vi "Main_Marvin Remake.vi"() -> ()   [LabVIEW 2017]
uses:
  PCAN_Driver/ControlCAN.llb/DevType.ctl
  PCAN_Driver/ControlCAN.llb/CAN Channel.ctl
  PCAN_Driver/ControlCAN.llb/VCI_INIT_CONFIG.ctl
  PCAN_Driver/ControlCAN.llb/InitFlag.ctl
  PCAN_Driver/ControlCAN.llb/Fliter.ctl
  PCAN_Driver/ControlCAN.llb/Mode.ctl
  <vilib>/Utility/miscctls.llb/LVRowAndColumnTypeDef.ctl
  <vilib>/Utility/config.llb/Read Key (String).vi
  <vilib>/Utility/config.llb/Write Key (String).vi
  <vilib>/Utility/cursorutil.llb/Set Cursor (Icon Pict).vi
  PCAN_Driver/ControlCAN.lvlib
  <vilib>/Utility/config.llb/NI_LVConfig.lvlib
panel:
  out "UUT from ID":u8
  out "UUT SN Report":string
  out "Automation":bool
  out "Test Failed":bool
  out "AuxiOFFResult":bool
  out "AuxiONResult":bool
  out "SensCalResult":bool
  out "VisualInspectionResult":bool
  out "BurnResult":bool
  out "BurnSpeed":bool
  out "BurnTemp":bool
  out "BurnDC":bool
  out "TempControlResult":bool
  out "MotorTempResult":bool
  out "StopTimeResult":bool
  out "SpeedResult":bool=TRUE
  out "VenableDirectionResult":bool
  out "VenableResult":bool
  out "ComTestResult":bool=TRUE
  out "UUT SoftwareVer":string
  out "Next SN":i32
  in  "SetSN":bool
  out "Current SN":i32
  out "Cal":dbl
  out "AO[1]Meas":dbl
  out "FullSpeed2 Speed":dbl
  out "FullSpeed2 Current":dbl
  out "FullSpeed1 Current":dbl
  out "FullSpeed1 Speed":dbl
  out "MaxBurnInTempVal":dbl
  in  "Stop Burn-in":bool
  out "VISA Tester":refnum<visa-resource-name>
  out "UUT":u8
  out "CAN Status":bool
  in  "Channel 2":T1 caption="Channel" items=["Channel 1", "Channel 2"]
  out "Config_CANAT":T7 {"DevType" items=["USB-CAN"=3, "USB-CAN2"=4]; "CanIndex" items=["通道1", "通道2"]; "VCI_INIT_CONFIG"."Fliter" items=["接收所有类型"=3, "只接收标准帧"=4, "只接收扩展帧"=7]; "VCI_INIT_CONFIG"."Mode" items=["正常工作", "自测模式（环回）", "仅侦听模式"]; "VCI_INIT_CONFIG"."InitFlag" items=["使用Flash参数", "使用界面设置参数"]}
  out "Array":u64[][](array[numeric]) format="%016x"
  out "Motor Phase Current RMS":dbl
  out "Ambient Temperature":dbl
  out "Speed error":bool
  out "Commutation err":bool
  out "Under voltage/Over voltage":bool
  out "Derated drive temp":bool
  out "Motor Over temperature":bool
  out "Motor Sensor temp Fauilre":bool
  out "Drive Over temperature":bool
  out "Drive Sensor temp Failure":bool
  out "Ambient Over temp":bool
  out "Ambient Sensor temp":bool
  out "DC Voltage":dbl
  out "DC Current":dbl
  out "Power transistor Heat sink Temp.":dbl
  out "Motor Stator Temp.":dbl
  out "Motor Speed RPM":dbl
  out "ECS State":u16
  out "UUT":string="EBAY"
  in  "Logger Path":path
  in  "Report":bool
  in  "Start":bool
  in  "ATR":string[][](table)=[["Test Communication", "-", "-", "-", "-", ""], ["Set S/N", "-", "-", "-", "-", ""], ["Set Board Number", "-", "-", "-", "-", ""], [" ", "", "", "", "", ""], ["Test Communication", "-", "-", "-", "-", ""], ["Get S/N", "-", "-", "-", "", ""], ["Get Board Number", "-", "-", "-", "", ""], ["Get FW", "-", "-", "-", "", ""], ["Enable Motor", "", "", "", "", ""], ["Small position command", "", "", "", "", ""], ["Measure delta", "", "", "", "", ""], ["Velocity command", "", "", "", "", ""]]
  in  "Settings":bool
  in  "Refresh Button":bool
  out "Status":bool
  in  "VISA Marvin":refnum<visa-resource-name>="COM6"
  in  "Serial Com":bool
  in  "Help Button":bool
  out "Pannel User Message":string
  in  "Stop Button":bool
  # "Marvin"
  # "REDLER TECHNOLOGIES LTD"
  # "ver 1.2j"
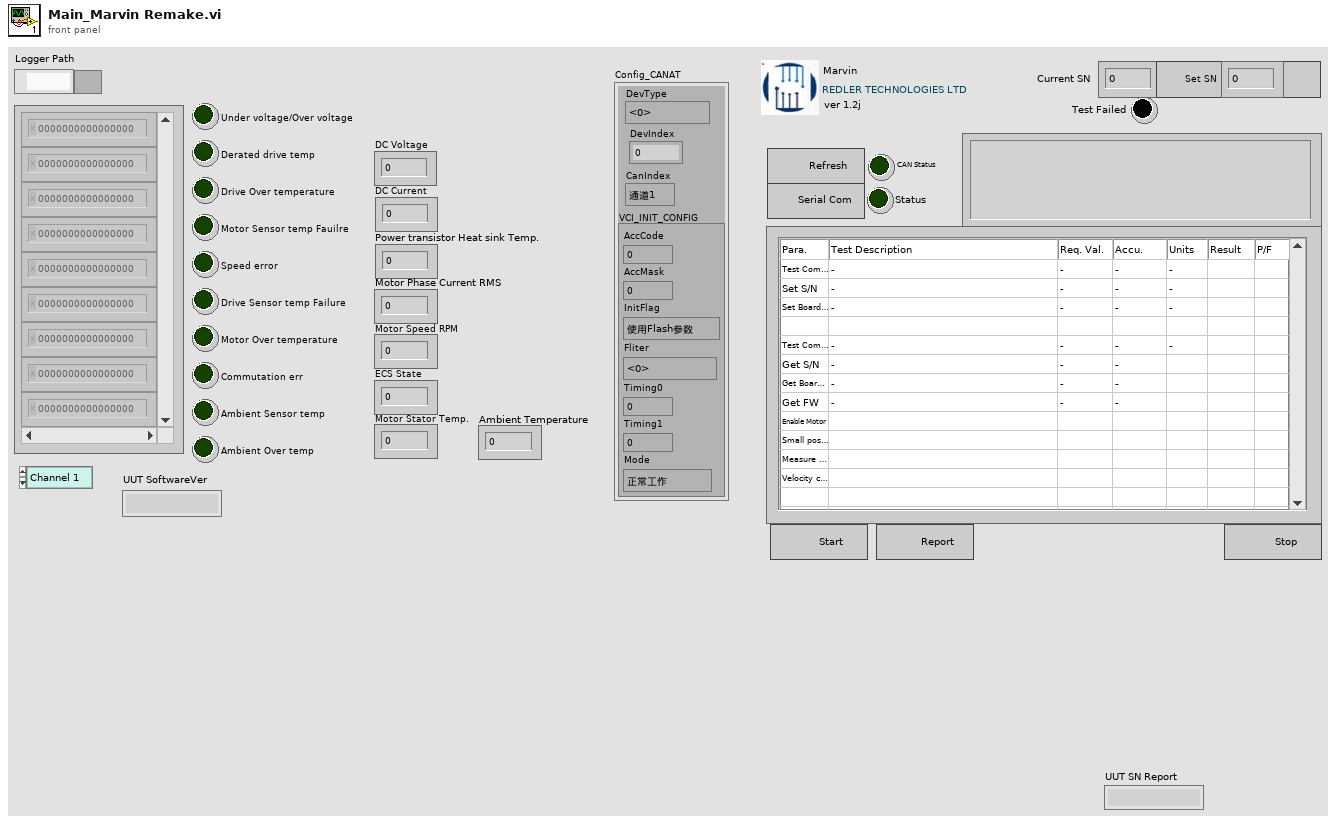
[diagram p1: front panel]
types:
  T1 = typedef "ControlCAN.lvlib/CAN Channel.ctl" = u32
  T2 = typedef "ControlCAN.lvlib/DevType.ctl" = u32
  T3 = typedef "ControlCAN.lvlib/VCI_INIT_CONFIG.ctl" = cluster{"AccCode":u32, "AccMask":u32, "InitFlag":T4, "Fliter":T5, "Timing0":u8, "Timing1":u8, "Mode":T6}
  T4 = typedef "ControlCAN.lvlib/InitFlag.ctl" = u32
  T5 = typedef "ControlCAN.lvlib/Fliter.ctl" = u8
  T6 = typedef "ControlCAN.lvlib/Mode.ctl" = u8
  T7 = cluster{"DevType":T2, "DevIndex":u32, "CanIndex":T1, "VCI_INIT_CONFIG":T3}
  T8 = cluster{"VISA":refnum<visa-resource-name>, "Array Test":enum16{"Auxiliary", "Temp Sens Cal", "Com Test", "Enable Test", "Speed Command", "Stop Time", "Temp Control", "Burn in", "Visual Inspec", "Empty"}[]}
  T9 = cluster{"ID":u32, "MSGTYPE":u8, "LEN":u8, "aDATA":u8[]}[]
  T10 = enum16{"Erase ATR Table", "Stop", "MainProgram", "Initialize"}
  T11 = enum16{"K15", "K16", "K17", "Venable", "Firmeware", "Fan", "Power", "120C", "110C", "100C", "90C", "80C", "70C", "60C", "50C", "40C", "30C", "25C", "20C", "10C", "0C"}
  T12 = enum16{"Stop", "Result", "FullSpeed2", "MD[1]=1", "FullSpeed1", "MD[1]=0"}
  T13 = enum8{"Term1", "Term2", "Current", "Fan", "TempCPU"}
  T14 = enum16{"Stop", "AO[1]=Meas.", "TA[5]", "AO[1]=0", "Start"}
  T15 = enum16{"Stop", "BurnIn", "Ambient Temp", "MotorSpeed", "DC Current Measure", "Start"}
  T16 = enum16{"Auxiliary", "Temp Sens Cal", "Com Test", "Enable Test", "Speed Command", "Stop Time", "Temp Control", "Burn in", "Visual Inspec", "Empty"}[]
  T17 = enum16{"K15", "K16", "K17", "Venable", "Firmeware", "Fan", "Power", "120C", "110C", "100C", "90C", "80C", "70C", "60C", "50C", "40C", "30C", "25C", "20C", "10C", "0C"}[]
  T18 = enum8{"Enabled", "Disabled", "Disabled and Grayed Out"}
  T19 = typedef "LVRowAndColumnTypeDef.ctl" = cluster{"Row":i32, "Column":i32}
  T20 = enum16{"Auxiliary", "Temp Sens Cal", "Com Test", "Enable Test", "Speed Command", "Stop Time", "Temp Control", "Burn in", "Visual Inspec", "Empty"}
  T21 = cluster{"ID":u32, "MSGTYPE":u8, "LEN":u8, "aDATA":u8[]}
  T22 = enum16{"open", "replace", "create", "open or create", "replace or create", "replace or create with confirmation"}
  T23 = enum32{"Invalid", "Standard", "Closed", "Hidden", "Minimized", "Maximized"}
  T24 = typedef "NI_LVConfig.lvlib/Config Data RefNum.ctl" = refnum<k1>
  T25 = typedef "ControlCAN.lvlib/VCI_CAN_OBJ.ctl" = cluster{"ID":u32, "TimeStamp":u32, "TimeFlag":u8, "SendType":u8, "RemoteFlag":u8, "ExternFlag":u8, "DataLen":u8, "Data":u8[], "Reserved":u8[]}
  T26 = cluster{"Type":enum16{"接收", "发送"}, "Channel":T1, "Time":timestamp, "VCI_CAN_OBJ":T25}[]
  T27 = cluster{"Type":enum16{"接收", "发送"}, "Channel":T1, "Time":timestamp, "VCI_CAN_OBJ":T25}
  T28 = typedef "LVPoint32TypeDef.ctl" = cluster{"Horizontal":i32, "Vertical":i32}
  T29 = enum8{"Term1", "Term2", "Current", "Fan", "TempCPU"}[]
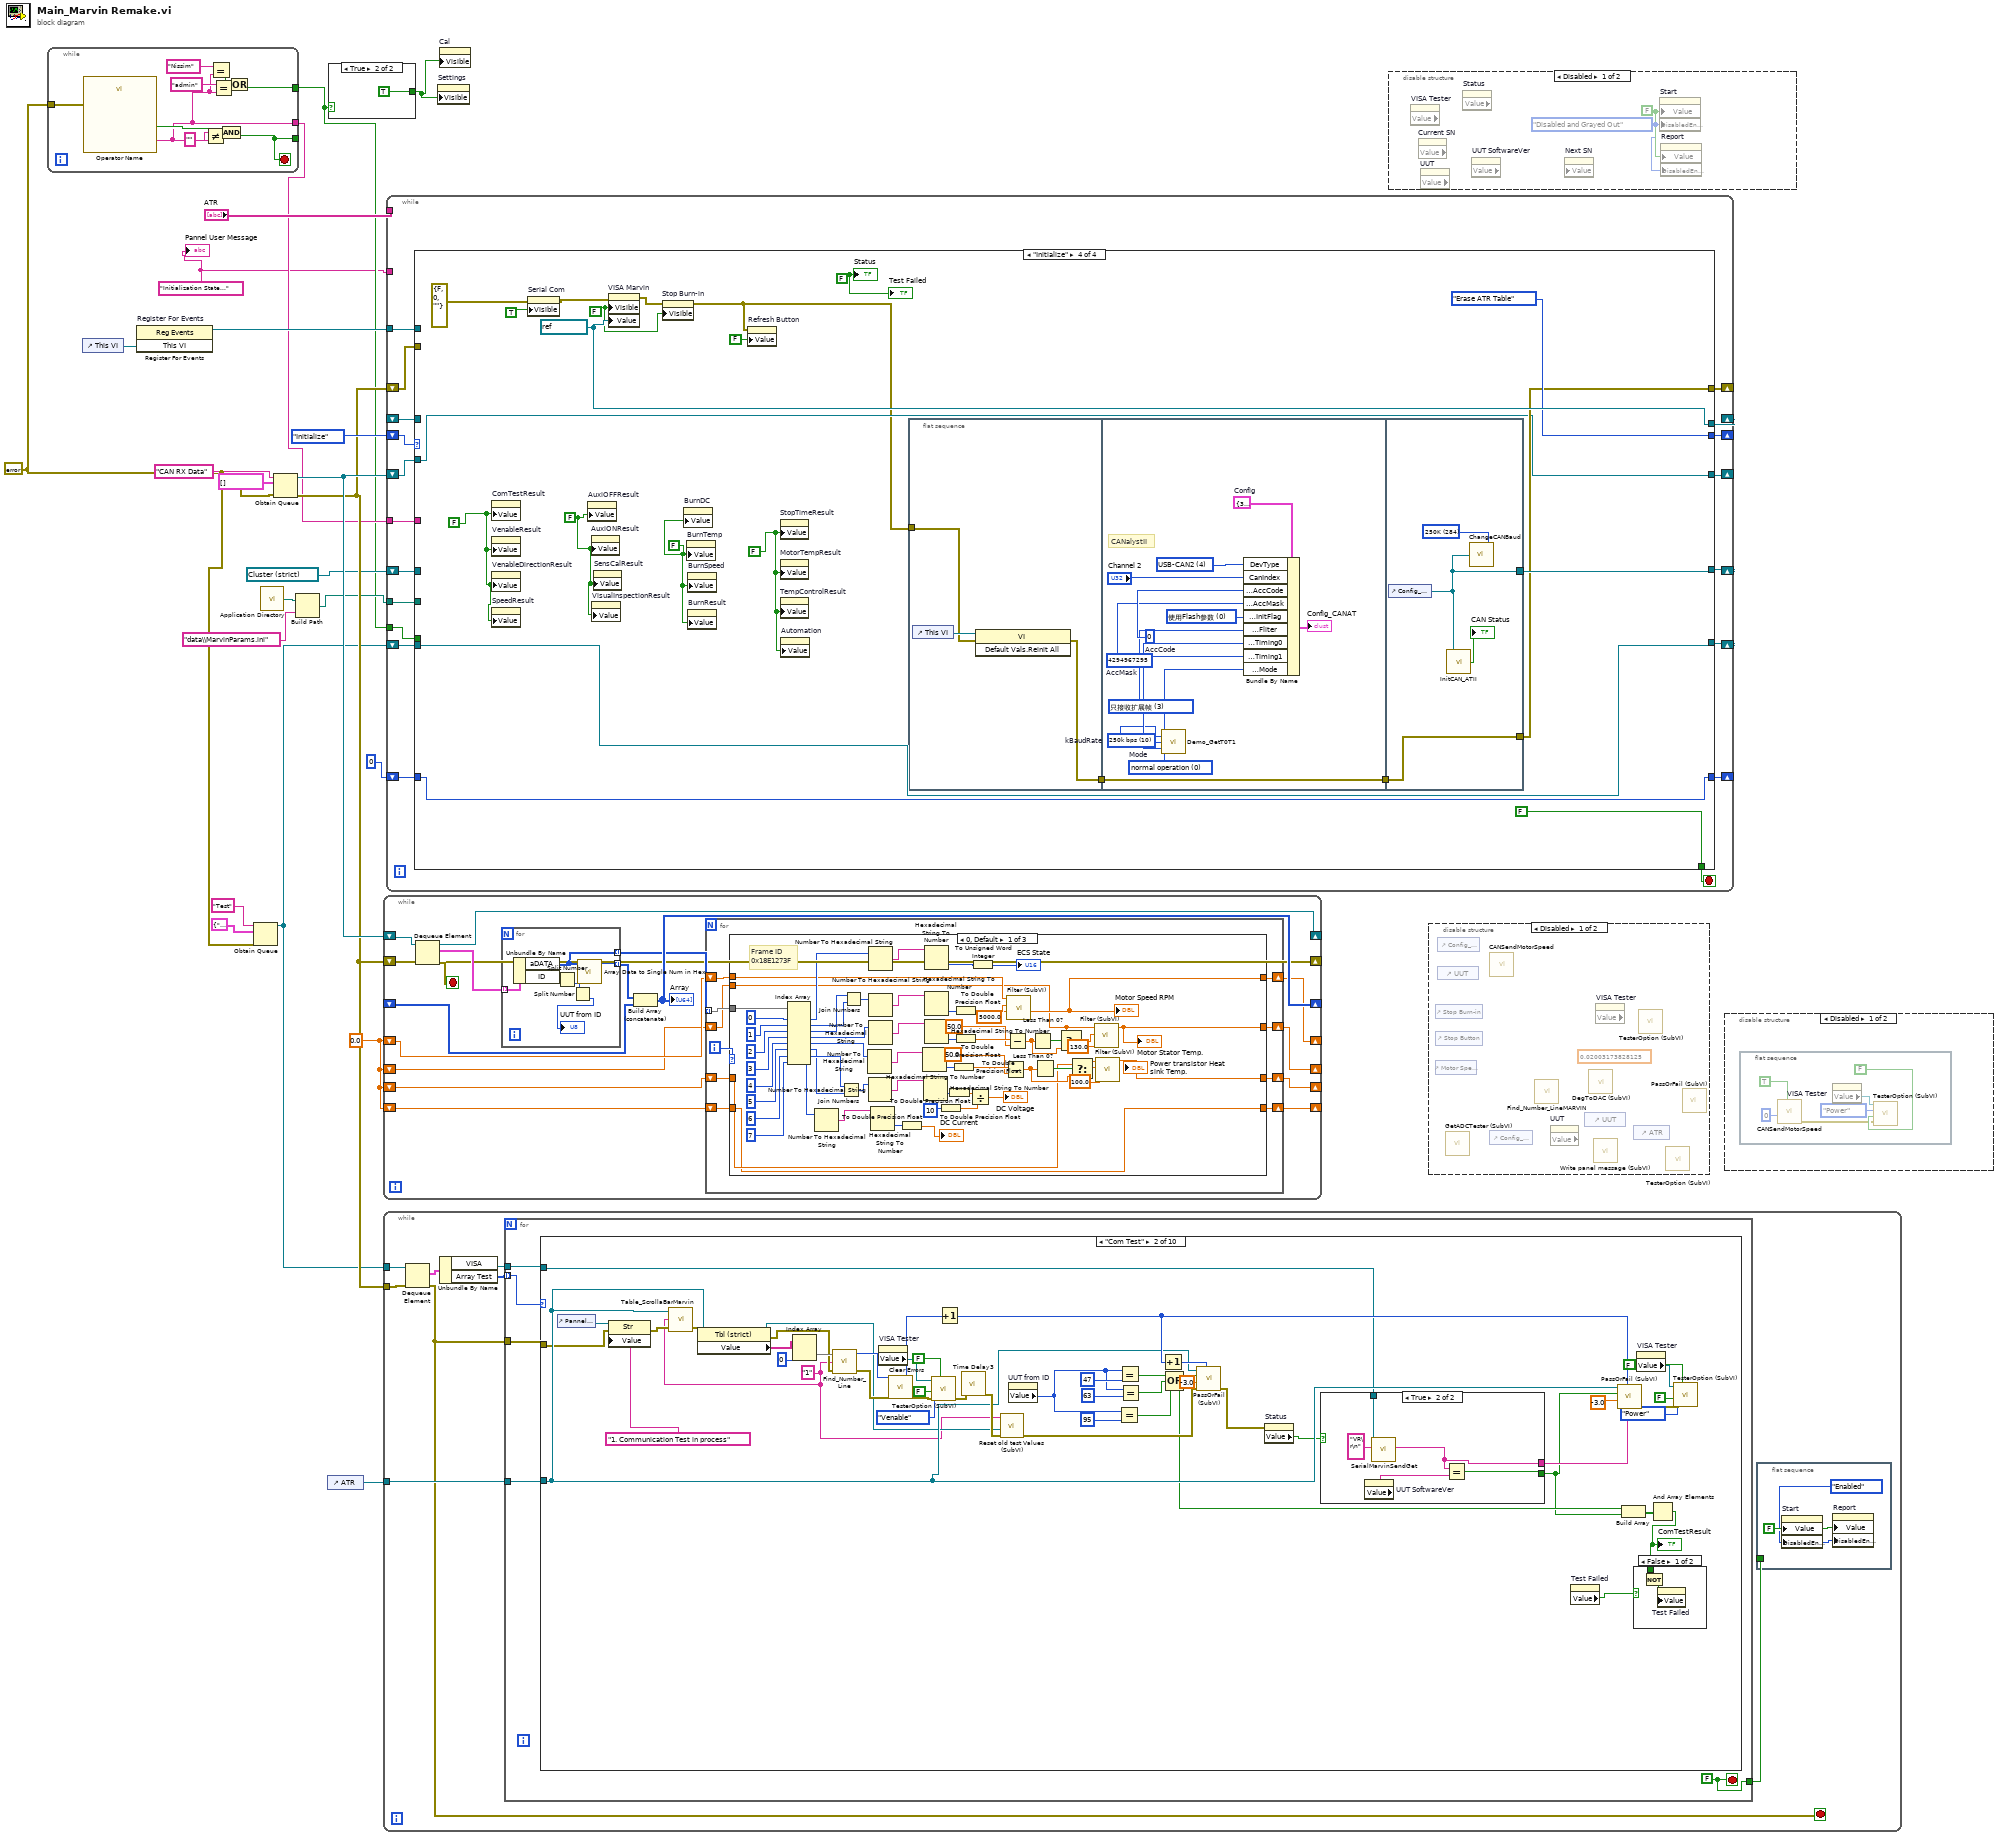
[diagram p0: block diagram]
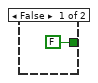
[diagram p2: hidden frame]
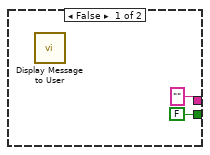
[diagram p8: hidden frame]
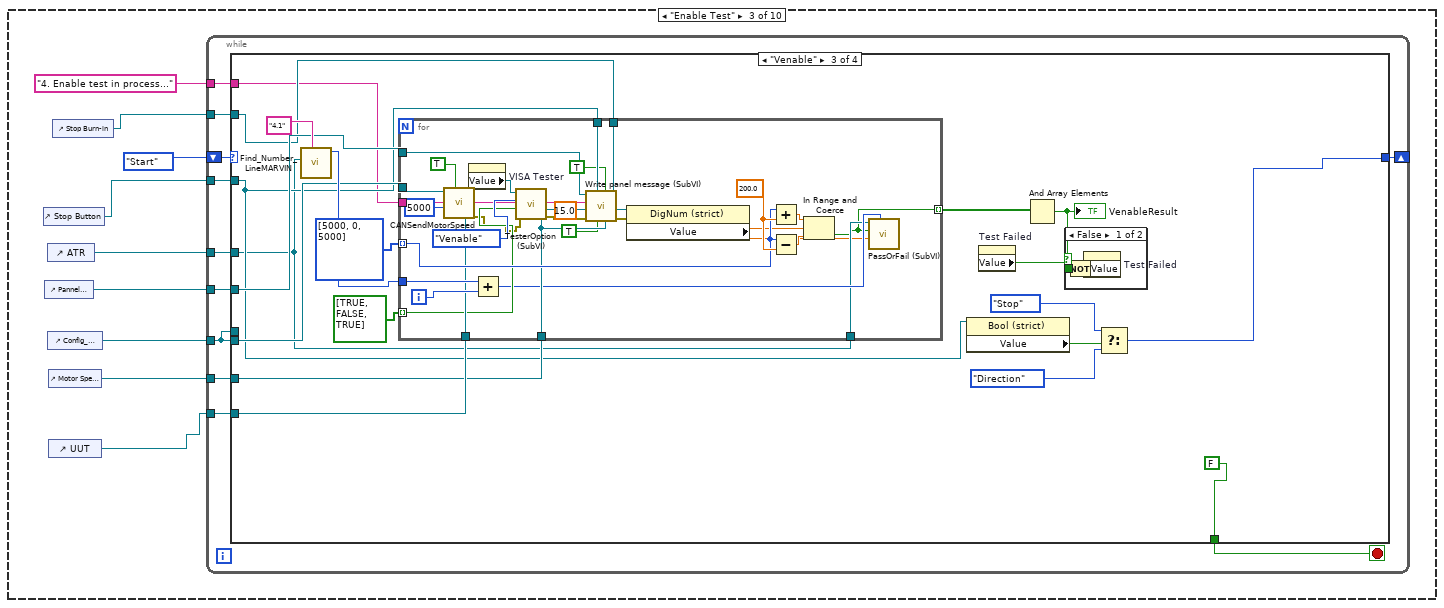
[diagram p9: hidden frame]
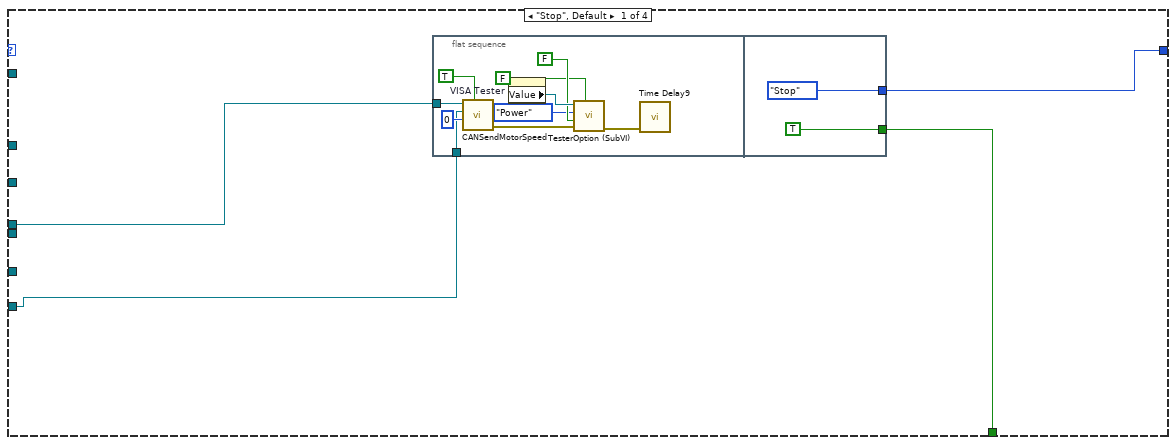
[diagram p10: hidden frame]
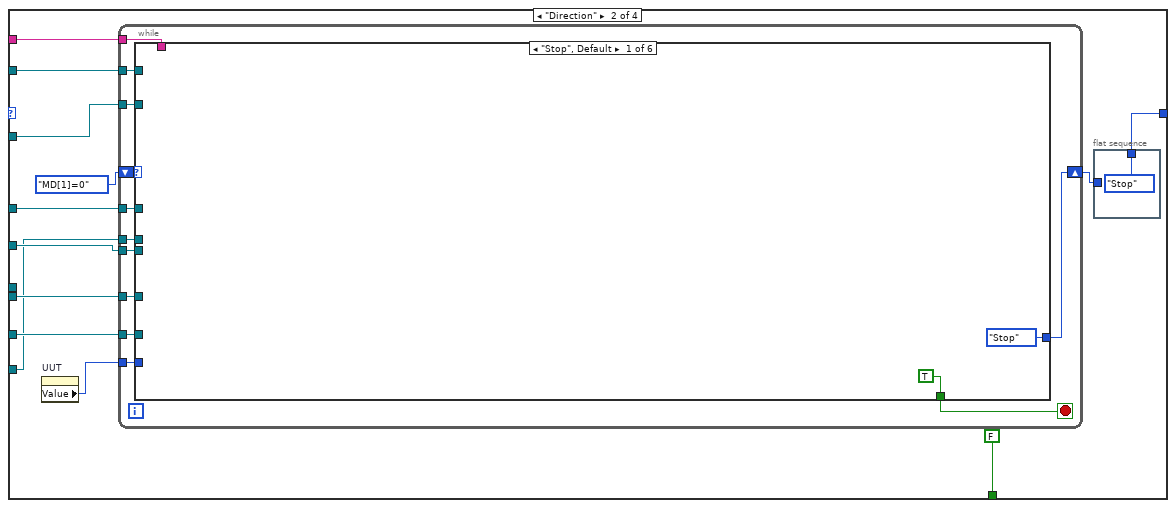
[diagram p11: hidden frame]
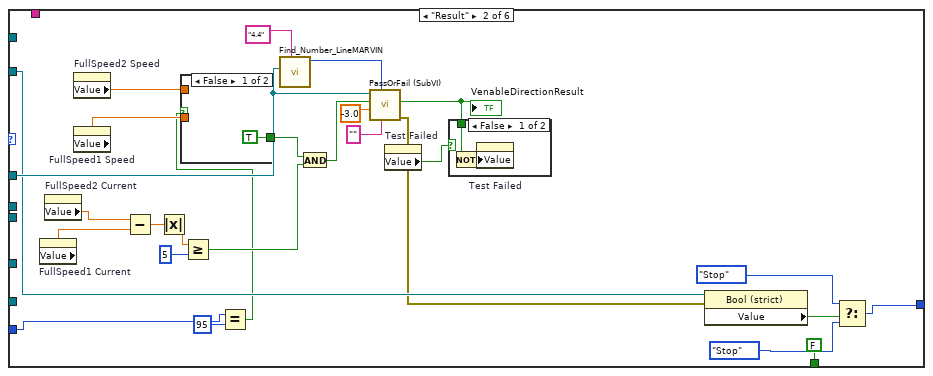
[diagram p12: hidden frame]
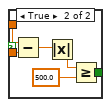
[diagram p14: hidden frame]
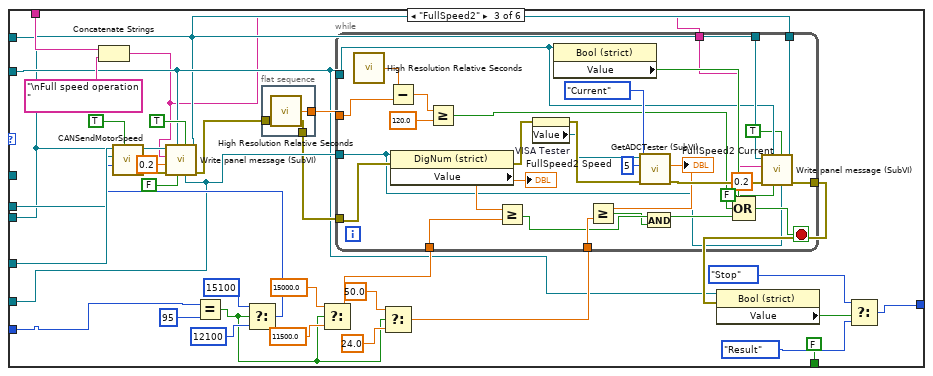
[diagram p15: hidden frame]
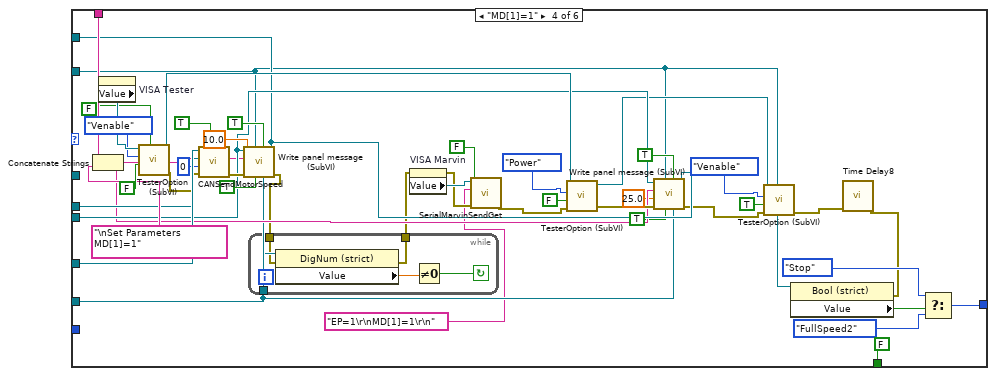
[diagram p16: hidden frame]
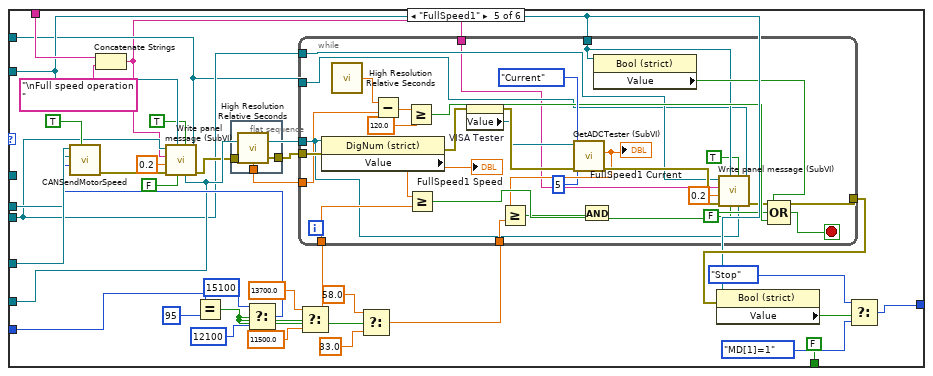
[diagram p17: hidden frame]
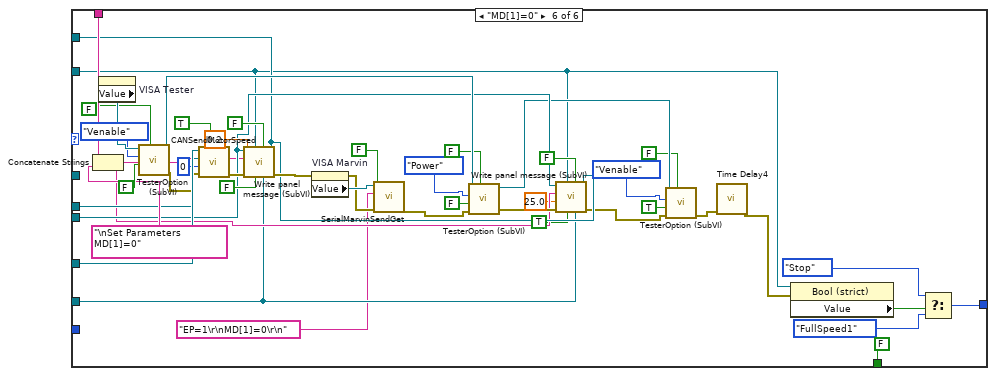
[diagram p18: hidden frame]
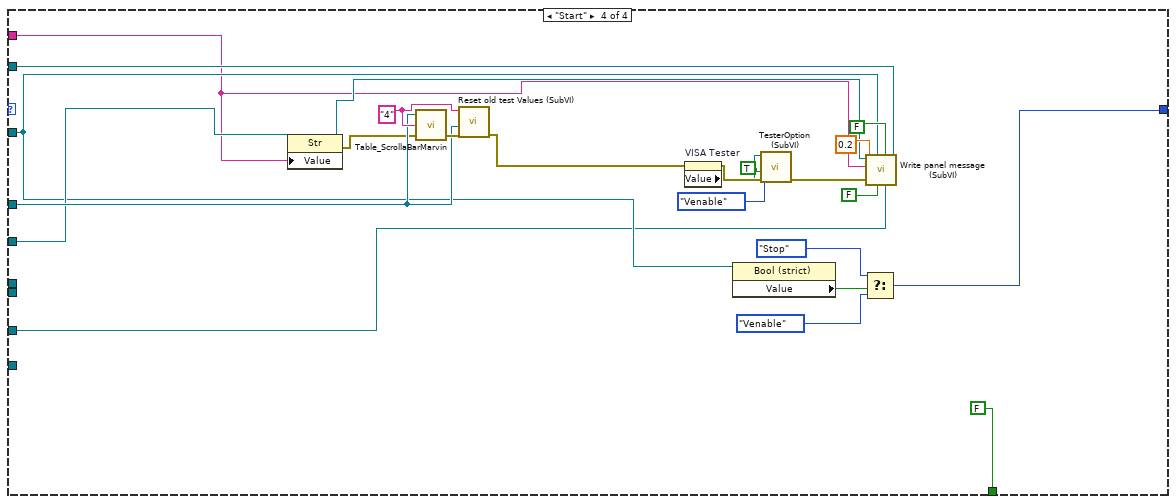
[diagram p20: hidden frame]
diagram:
  w1 = "Initialization State..."
  w12 = 0.0
  w11 = errorcluster {"status"=FALSE, "code"=0, "source"=""} ("error in (no error)")
  n1 = while {
    tunnel: [w31] -> _
    tunnel: [w27] -> w6
    tunnel: [w28] -> w2
    tunnel: w11 -> [w24]
    stop <- w31 stop-if-true
    n2 = call "Operator Name"("error in (no error)"=w24) -> ("Operator Name"=w27:string, "OK"=w32:bool)  [unwired: 16 in, 1 out]
    n3 = Not Equal?(x=w27, y="") -> (x != y?=w33:bool)
    n4 = Equal?(x="Nissim", y=w27) -> (x = y?=w25:bool)
    n5 = Equal?(x="admin", y=w27) -> (x = y?=w29:bool)
    n6 = And(x=w32, y=w33) -> (x .and. y?=w31:bool)
    n7 = Or(x=w25, y=w29) -> (x .or. y?=w28:bool)
  }
  n8 = control-ref of="This VI"() -> (w8:refnum<vi>)
  n9 = register-events "Register For Events"(w8) -> (reference out=w7:refnum<event-registration>)  [unwired: 2 in, 1 out]
  n10 = Obtain Queue(name (unnamed)="Test", element data type=T8 {"VISA"="COM1", "Array Test"=[]}, error in (no error)=w11) -> (queue out=w16:refnum<queue>)  [unwired: 2 in, 2 out]
  n11 = call <vilib>:"Application Directory.vi"() -> ("Application Directory"=w10:path)
  n12 = Obtain Queue(name (unnamed)="CAN RX Data", element data type=T9 [], error in (no error)=w11) -> (queue out=w20:refnum<queue>, error out=w17:errorcluster)  [unwired: 2 in, 1 out]
  n13 = Build Path(base path=w10, name or relative path="data\\MarvinParams.ini") -> (appended path=w4:path)
  n14 = control-ref of="ATR"() -> (w18:refnum<vi>)
  n15 = case shown="True" w2 {
    tunnel: [FALSE TRUE] -> w3
    frame False {
    }
    frame True {
    }
  }
  n16 = while {
    shift-right: [w51] -> _
    shift-left: w20 -> [w53]
    shift-right: [w49] -> _
    shift-left: _ -> [w50]
    shift-right: [w45] -> _
    shift-left: w17 -> [w45]
    shift-right: [w43] -> _
    shift-left: w12 -> [w44]
    shift-right: [w42] -> _
    shift-left: w12 -> [w41]
    shift-right: [w40] -> _
    shift-left: w12 -> [w39]
    shift-right: [w38] -> _
    shift-left: w12 -> [w37]
    stop <- w52 stop-if-true
    n17 = Dequeue Element(queue=w53, error in (no error)=w45) -> (queue out=w51:refnum<queue>, element=w46:T9, error out=w52:errorcluster)  [unwired: 1 in, 1 out]
    n18 = for {
      tunnel: [w185] -> w48 mode=indexing
      tunnel: w46 -> [w184] mode=indexing
      tunnel: [w183] -> w47 mode=indexing
      n19 = Unbundle By Name(w184) -> ("aDATA"=w183:u8[], "ID"=w181:u32)
      n20 = Split Number(x=w181) -> (lo(x)=w182:u16)  [unwired: 1 out]
      n21 = Split Number(x=w182) -> (lo(x)=→"UUT from ID":u8)  [unwired: 1 out]
      n22 = call "Array Data to Single Num in Hex.vi"("aDATA"=w183) -> ("Numeric"=w185:u64)  [unwired: 10 in]
    }
    n23 = Build Array (concatenate)(w48, w50) -> (w49:u64[][])
    "Array" <- w49
    n24 = for {
      tunnel: w47 -> [w63] mode=indexing
      shift-right: [w60] -> w43
      shift-left: w44 -> [w61]
      shift-right: [w59] -> w42
      shift-left: w41 -> [w58]
      shift-right: [w57] -> w40
      shift-left: w39 -> [w56]
      shift-right: [w55] -> w38
      shift-left: w37 -> [w54]
      i -> [w62]
      n25 = case shown="0, Default" w62 {
        tunnel: w63 -> [w103 w136 w175]
        tunnel: w61 -> [w77 w125 w164]
        tunnel: [w75 w125 w164] -> w60
        tunnel: [w72 w124 w163] -> w59
        tunnel: w58 -> [w71 w124 w163]
        tunnel: [w66 w123 w162] -> w57
        tunnel: w56 -> [w65 w123 w162]
        tunnel: [w64 w122 w157] -> w55
        tunnel: w54 -> [w64 w122 w156]
        frame 0, Default {
          # "Frame ID\n0x18E1273F"
          n26 = Index Array(array=w103, index #1=0 ("index"), index #2=1 ("index"), index #3=2 ("index"), index #4=3 ("index"), index #5=4 ("index"), index #6=5 ("index"), index #7=6 ("index"), index #8=7 ("index")) -> (element #1=w87:u8, element #2=w89:u8, element #3=w90:u8, element #4=w94:u8, element #5=w97:u8, element #6=w101:u8, element #7=w102:u8, element #8=w100:u8)
          n27 = Number To Hexadecimal String(2:w100) -> (0:w114:string)  [unwired: 1 in]
          n28 = Join Numbers(hi=w102, lo=w101) -> ((hi.lo)=w121:u16)
          n29 = Join Numbers(hi=w90, lo=w89) -> ((hi.lo)=w91:u16)
          n30 = Number To Hexadecimal String(2:w97) -> (0:w98:string)  [unwired: 1 in]
          n31 = Number To Hexadecimal String(2:w121) -> (0:w120:string)  [unwired: 1 in]
          n32 = Number To Hexadecimal String(2:w87) -> (0:w88:string)  [unwired: 1 in]
          n33 = Number To Hexadecimal String(2:w91) -> (0:w92:string)  [unwired: 1 in]
          n34 = Number To Hexadecimal String(2:w94) -> (0:w95:string)  [unwired: 1 in]
          n35 = Hexadecimal String To Number(string=w114) -> (number=w113:u32)  [unwired: 2 in, 1 out]
          n36 = To Double Precision Float(number=w113) -> (double precision float=→"DC Current":dbl)
          n37 = Hexadecimal String To Number(string=w98) -> (number=w99:u32)  [unwired: 2 in, 1 out]
          n38 = Hexadecimal String To Number(string=w120) -> (number=w119:u32)  [unwired: 2 in, 1 out]
          n39 = Hexadecimal String To Number(string=w88) -> (number=w85:u32)  [unwired: 2 in, 1 out]
          n40 = Hexadecimal String To Number(string=w92) -> (number=w93:u32)  [unwired: 2 in, 1 out]
          n41 = Hexadecimal String To Number(string=w95) -> (number=w96:u32)  [unwired: 2 in, 1 out]
          n42 = To Double Precision Float(number=u32 10 ("y")) -> (double precision float=w117:dbl)
          n43 = To Double Precision Float(number=w119) -> (double precision float=w116:dbl)
          n44 = To Double Precision Float(number=w99) -> (double precision float=w82:dbl)
          n45 = To Double Precision Float(number=w93) -> (double precision float=w78:dbl)
          n46 = To Double Precision Float(number=w96) -> (double precision float=w84:dbl)
          n47 = Divide(x=w116, y=w117) -> (x/y=→"DC Voltage":dbl)
          n48 = To Unsigned Word Integer(number=w85) -> (unsigned 16bit integer=→"ECS State":u16)
          n49 = Subtract(x=w82, y=50.0 ("x")) -> (x-y=w70:dbl)
          n50 = Subtract(x=w84, y=50.0 ("x")) -> (x-y=w73:dbl)
          n51 = call "Filter (SubVI).vi"("Delta"=5000.0, "NewVal"=w78, "OldVal"=w77) -> ("Val"=w75:dbl)  [unwired: 8 in]
          "Motor Speed RPM" <- w75
          n52 = Less Than 0?(x=w73) -> (x < 0?=w80:bool)
          n53 = Less Than 0?(x=w70) -> (x < 0?=w79:bool)
          n54 = Select(t=w71, s=w80, f=w73) -> (s? t:f=w74:dbl)
          n55 = Select(t=w65, s=w79, f=w70) -> (s? t:f=w69:dbl)
          n56 = call "Filter (SubVI).vi"("Delta"=130.0, "NewVal"=w74, "OldVal"=w71) -> ("Val"=w72:dbl)  [unwired: 8 in]
          "Motor Stator Temp." <- w72
          n57 = call "Filter (SubVI).vi"("Delta"=100.0, "NewVal"=w69, "OldVal"=w65) -> ("Val"=w66:dbl)  [unwired: 8 in]
          "Power transistor Heat sink Temp." <- w66
        }
        frame 1 {
          # "Framde ID\n0x18E3273F"
          n58 = control-ref of="UUT"() -> (w126:refnum<vi>)
          n59 = property on="Property Node" class="DigNum (strict)"(reference=w126) -> ("Value"=w127:u8)  [unwired: 1 in, 2 out]
          n60 = Index Array(array=w136, index #1=0 ("index"), index #2=1 ("index")) -> (element #1=w134:u8, element #2=w129:u8)
          n61 = Number To Boolean Array(number=w134) -> (Boolean array=w133:bool[])
          n62 = Number To Boolean Array(number=w129) -> (Boolean array=w131:bool[])
          n63 = Boolean To (0,1)(Boolean=w131) -> (0, 1=w128:i16[])
          n64 = Boolean To (0,1)(Boolean=w133) -> (0, 1=w132:i16[])
          n65 = case shown="95" w127 {
            tunnel: w128 -> [_ w137]
            frame 0, Default {
            }
            frame 95 {
              n66 = for {
                tunnel: w137 -> [w142] mode=indexing
                i -> [w138]
                stop <- w140 stop-if-true
                n67 = Not Equal To 0?(x=w142) -> (x != 0?=w141:bool)
                n68 = case shown="0, Default" w138 {
                  tunnel: w141 -> [w143 w144]
                  frame 0, Default {
                    "Ambient Sensor temp" <- w143
                  }
                  frame 1 {
                    "Ambient Over temp" <- w144
                  }
                }
                n69 = Equal?(x=w138, y=1.0) -> (x = y?=w140:bool)
              }
            }
          }
          n70 = for {
            tunnel: w132 -> [w146] mode=indexing
            i -> [w147]
            n71 = Not Equal To 0?(x=w146) -> (x != 0?=w145:bool)
            n72 = case shown="1" w147 {
              tunnel: w145 -> [w148 w149 w150 w151 w152 w153 w154 w155]
              frame 0, Default {
                "Drive Sensor temp Failure" <- w148
              }
              frame 1 {
                "Drive Over temperature" <- w149
              }
              frame 2 {
                "Motor Sensor temp Fauilre" <- w150
              }
              frame 3 {
                "Motor Over temperature" <- w151
              }
              frame 4 {
                "Derated drive temp" <- w152
              }
              frame 5 {
                "Under voltage/Over voltage" <- w153
              }
              frame 6 {
                "Commutation err" <- w154
              }
              frame 7 {
                "Speed error" <- w155
              }
            }
          }
        }
        frame 2 {
          # "Frame ID\n0x18E2273F"
          n73 = Index Array(array=w175, index #1=0 ("index"), index #2=1 ("index")) -> (element #1=w172:u8, element #2=w169:u8)
          n74 = disable-structure shown="Enabled" {
            disable-tunnel: [w178 w179] -> w173
            disable-tunnel: w172 -> [w177 w179]
            frame Disabled {
              n75 = Number To Hexadecimal String(2:w177) -> (0:w176:string)  [unwired: 1 in]
              n76 = Hexadecimal String To Number(string=w176) -> (number=w178:u32)  [unwired: 2 in, 1 out]
            }
            frame Enabled {
            }
          }
          n77 = Number To Hexadecimal String(2:w169) -> (0:w167:string)  [unwired: 1 in]
          n78 = Hexadecimal String To Number(string=w167) -> (number=w168:u32)  [unwired: 2 in, 1 out]
          n79 = To Double Precision Float(number=w168) -> (double precision float=w166:dbl)
          n80 = To Double Precision Float(number=w173) -> (double precision float=→"Motor Phase Current RMS":dbl)
          n81 = Subtract(x=w166, y=50.0) -> (x-y=w160:dbl)
          n82 = Less Than 0?(x=w160) -> (x < 0?=w161:bool)
          n83 = Select(t=w156, s=w161, f=w160) -> (s? t:f=w159:dbl)
          n84 = call "Filter (SubVI).vi"("Delta"=65.0, "NewVal"=w159, "OldVal"=w156) -> ("Val"=w157:dbl)  [unwired: 8 in]
          "Ambient Temperature" <- w157
        }
      }
    }
  }
  n85 = while {
    tunnel: w18 -> [w193]
    tunnel: w17 -> [w191]
    tunnel: w16 -> [w192]
    stop <- w187 stop-if-true
    n86 = Dequeue Element(queue=w192, error in (no error)=w191) -> (element=w190:T8, error out=w187:errorcluster)  [unwired: 1 in, 2 out]
    n87 = Unbundle By Name(w190) -> ("VISA"=w189:refnum<visa-resource-name>, "Array Test"=w188:T16)
    n88 = for {
      tunnel: w188 -> [w197] mode=indexing
      tunnel: w189 -> [w200]
      tunnel: w193 -> [w199]
      tunnel: w187 -> [w198]
      tunnel: [w196] -> w186
      stop <- w196 stop-if-true
      w196 = FALSE
      n89 = case shown="\"Com Test\"" w197 {
        tunnel: w200 -> [_ w226 _ _ w831 _ _ _ w1406 _]
        tunnel: w199 -> [_ w233 _ w660 w827 w993 _ w1388 w1413 w1628]
        tunnel: w198 -> [_ w230 _ w675 w837 w991 _ w1387 w1411 w1627]
        frame "Empty", Default {
        }
        frame "Com Test" {
          w207 = "1" ("Test Paragraph")
          n90 = control-ref of="Pannel User Message"() -> (w231:refnum<vi>)
          n91 = property class="Str"(reference=w231, error in=w230, "Value"="1. Communication Test in process") -> (error out=w229:errorcluster)  [unwired: 1 out]
          n92 = call "Table_ScrollaBarMarvin.vi"("error in"=w229, "Line to focus"=w207, "reference in"=w233) -> ("error out"=w232:errorcluster)  [unwired: 2 out]
          n93 = property class="Tbl (strict)"(reference=w233, error in=w232) -> (reference out=w208:refnum<vi>, error out=w245:errorcluster, "Value"=w246:string[][])
          n94 = Index Array(array=w246, index (col)=0 ("disabled index (col)")) -> (element=w247:string[])  [unwired: 1 in]
          n95 = call "Find_Number_Line.vi"("error in"=w245, "Test Paragraph"=w207, "Row Headers[]"=w247) -> ("error out"=w243:errorcluster, "Line number"=w242:i32)  [unwired: 1 out]
          n96 = property on="VISA Tester" class="VISAName"() -> ("Value"=w219:refnum<visa-resource-name>)  [unwired: 2 in, 2 out]
          n97 = call <vilib>:"Clear Errors.vi"("error in (no error)"=w243) -> ("error out"=w221:errorcluster)  [unwired: 5 in, 1 out]
          n98 = call "TesterOption (SubVI).vi"("2 Options"=FALSE, "error in (no error)"=w221, "On/Off"=FALSE, "Tester Option"=T11."Venable", "VISA Refnum in"=w219) -> ("error out"=w220:errorcluster)  [unwired: 5 in, 1 out]
          n99 = Increment(x=w242) -> (x+1=w236:i32)
          n100 = call "Time Delay3"("error in (no error)"=w220) -> ("error out"=w234:errorcluster)  [unwired: 10 in]
          n101 = call "Reset old test Values (SubVI).vi"("error in"=w234, "Atr in"=w208, "Test Paragraph"=w207) -> ("error out"=w209:errorcluster)  [unwired: 8 in]
          n102 = property on="UUT from ID" class="DigNum (strict)"() -> ("Value"=w201:u8)  [unwired: 2 in, 2 out]
          n103 = Equal?(x=w201, y=u8 95) -> (x = y?=w224:bool)
          n104 = Equal?(x=w201, y=u8 47) -> (x = y?=w238:bool)
          n105 = Equal?(x=w201, y=u8 63) -> (x = y?=w237:bool)
          n106 = Increment(x=w236) -> (x+1=w235:i32)
          n107 = Compound Arithmetic op=OR(w238, w237, w224) -> (w205:bool)
          n108 = call "PassOrFail (SubVI).vi"("index (row)"=w235, "error in (no error)"=w209, "Data in"=-3.0, "Pass?Fail"=w205, "Table in"=w233) -> ("error out"=w225:errorcluster)  [unwired: 6 in]
          n109 = property on="Status" class="Bool (strict)"(error in=w225) -> ("Value"=w227:bool)  [unwired: 1 in, 2 out]
          n110 = case shown="True" w227 {
            tunnel: w226 -> [_ w256]
            tunnel: [FALSE w253] -> w204
            tunnel: ["" ("read buffer") w252] -> w223
            frame False {
              n111 = call "Display Message to User"() -> ()  [unwired: 10 in, 2 out]
            }
            frame True {
              n112 = property on="UUT SoftwareVer" class="Str"() -> ("Value"=w254:string)  [unwired: 2 in, 2 out]
              n113 = call "SerialMarvinSendGet.vi"("write buffer"="VR\r\n", "VISA resource name"=w256) -> ("read buffer"=w252:string)  [unwired: 8 in, 1 out]
              n114 = Equal?(x=w252, y=w254) -> (x = y?=w253:bool)
            }
          }
          n115 = property on="Test Failed" class="Bool (strict)"() -> ("Value"=w202:bool)  [unwired: 2 in, 2 out]
          n116 = call "PassOrFail (SubVI).vi"("String Res"=w223, "index (row)"=w236, "Data in"=-3.0, "Pass?Fail"=w204, "Table in"=w233) -> ("error out"=w215:errorcluster)  [unwired: 6 in]
          n117 = Build Array(w205, w204) -> (w206:bool[])
          n118 = property on="VISA Tester" class="VISAName"() -> ("Value"=w214:refnum<visa-resource-name>)  [unwired: 2 in, 2 out]
          n119 = And Array Elements(Boolean array=w206) -> (logical AND=w203:bool)
          "ComTestResult" <- w203
          n120 = case shown="False" w202 {
            tunnel: w203 -> [w249 _]
            frame False {
              n121 = Not(x=w249) -> (.not. x?=w248:bool)
              n122 = property on="Test Failed" class="Bool (strict)"("Value"=w248) -> ()  [unwired: 2 in, 2 out]
            }
            frame True {
            }
          }
          n123 = call "TesterOption (SubVI).vi"("2 Options"=FALSE, "error in (no error)"=w215, "On/Off"=FALSE, "Tester Option"=T11."Power", "VISA Refnum in"=w214) -> ()  [unwired: 5 in, 2 out]
        }
        frame "Enable Test" {
          n124 = control-ref of="Stop Button"() -> (w259:refnum<vi>)
          n125 = control-ref of="Pannel User Message"() -> (w261:refnum<vi>)
          n126 = control-ref of="ATR"() -> (w260:refnum<vi>)
          n127 = control-ref of="Config_CANAT"() -> (w262:refnum<vi>)
          n128 = control-ref of="Motor Speed RPM"() -> (w263:refnum<vi>)
          n129 = control-ref of="UUT"() -> (w264:refnum<vi>)
          n130 = control-ref of="Stop Burn-in"() -> (w265:refnum<vi>)
          n131 = while {
            shift-right: [w270] -> _
            shift-left: enum16{"Stop", "Direction", "Venable", "Start"}."Start" -> [w276]
            tunnel: w259 -> [w275]
            tunnel: w260 -> [w274]
            tunnel: w261 -> [w273]
            tunnel: w262 -> [w266]
            tunnel: w263 -> [w272]
            tunnel: w264 -> [w267]
            tunnel: w265 -> [w269]
            tunnel: "4. Enable test in process..." ("Strin") -> [w268]
            stop <- w271 stop-if-true
            n132 = case shown="\"Venable\"" w276 {
              tunnel: w275 -> [_ w303 w592 w639]
              tunnel: w274 -> [_ w298 w590 w646]
              tunnel: w273 -> [_ w301 w594 w645]
              tunnel: w266 -> [_ w304 w597 _]
              tunnel: w272 -> [_ w300 w595 w637]
              tunnel: w267 -> [w277 w294 w596 _]
              tunnel: [w280 FALSE FALSE FALSE] -> w271
              tunnel: [w278 w297 w591 w643] -> w270
              tunnel: w269 -> [_ w302 w593 w638]
              tunnel: w268 -> [_ w299 w589 w636]
              tunnel: w266 -> [w279 _ _ _]
              frame "Stop", Default {
                n133 = flat-sequence {
                  tunnel: w277 -> [w286]
                  tunnel: w279 -> [w285]
                  tunnel: [TRUE] -> w280
                  tunnel: [enum16{"Stop", "Direction", "Venable", "Start"}."Stop"] -> w278
                  frame #0 {
                    n134 = call "CANSendMotorSpeed.vi"("Remote"=TRUE, "Motor Speed RPM"=u16 0, "UUT"=w286, "CAN Cluster in"=w285) -> ("error out"=w289:errorcluster)  [unwired: 7 in]
                    n135 = property on="VISA Tester" class="VISAName"() -> ("Value"=w290:refnum<visa-resource-name>)  [unwired: 2 in, 2 out]
                    n136 = call "TesterOption (SubVI).vi"("2 Options"=FALSE, "error in (no error)"=w289, "On/Off"=FALSE, "Tester Option"=T11."Power", "VISA Refnum in"=w290) -> ("error out"=w281:errorcluster)  [unwired: 5 in, 1 out]
                    n137 = call "Time Delay9"("error in (no error)"=w281) -> ()  [unwired: 10 in, 1 out]
                  }
                  frame #1 {
                  }
                }
              }
              frame "Direction" {
                n138 = property on="UUT" class="DigNum (strict)"() -> ("Value"=w293:u8)  [unwired: 2 in, 2 out]
                n139 = while {
                  shift-right: [w317] -> w296
                  shift-left: T12."MD[1]=0" -> [w318]
                  tunnel: w304 -> [w315]
                  tunnel: w294 -> [w314]
                  tunnel: w303 -> [w313]
                  tunnel: w302 -> [w312]
                  tunnel: w301 -> [w311]
                  tunnel: w300 -> [w310]
                  tunnel: w299 -> [w309]
                  tunnel: w298 -> [w308]
                  tunnel: w293 -> [w307]
                  stop <- w316 stop-if-true
                  n140 = case shown="\"Stop\", Default" w318 {
                    tunnel: [T12."Stop" w343 w387 w466 w504 w584] -> w317
                    tunnel: [TRUE FALSE FALSE FALSE FALSE FALSE] -> w316
                    tunnel: w315 -> [_ _ w385 w460 w502 w578]
                    tunnel: w314 -> [_ _ w381 w439 w498 w556]
                    tunnel: w313 -> [_ w330 w360 w430 w480 w546]
                    tunnel: w312 -> [_ _ w358 w440 w478 w557]
                    tunnel: w311 -> [_ _ w359 w441 w479 w558]
                    tunnel: w310 -> [_ _ w376 w428 w494 w552]
                    tunnel: w309 -> [_ _ w371 w449 w492 w566]
                    tunnel: w308 -> [_ w334 _ _ _ _]
                    tunnel: w307 -> [_ w321 w356 _ w473 _]
                    frame "Stop", Default {
                    }
                    frame "Result" {
                      n141 = property on="FullSpeed1 Current" class="DigNum (strict)"() -> ("Value"=w338:dbl)  [unwired: 2 in, 2 out]
                      n142 = property on="FullSpeed2 Current" class="DigNum (strict)"() -> ("Value"=w339:dbl)  [unwired: 2 in, 2 out]
                      n143 = property on="FullSpeed2 Speed" class="DigNum (strict)"() -> ("Value"=w341:dbl)  [unwired: 2 in, 2 out]
                      n144 = property on="FullSpeed1 Speed" class="DigNum (strict)"() -> ("Value"=w340:dbl)  [unwired: 2 in, 2 out]
                      n145 = Subtract(x=w339, y=w338) -> (x-y=w337:dbl)
                      n146 = Absolute Value(x=w337) -> (abs(x)=w326:dbl)
                      n147 = Greater Or Equal?(x=w326, y=u32 5) -> (x >= y?=w332:bool)
                      n148 = Equal?(x=w321, y=u8 95) -> (x = y?=w324:bool)
                      n149 = case shown="False" w324 {
                        tunnel: w341 -> [_ w354]
                        tunnel: w340 -> [_ w353]
                        tunnel: [TRUE w350] -> w333
                        frame False {
                        }
                        frame True {
                          n150 = Subtract(x=w354, y=w353) -> (x-y=w355:dbl)
                          n151 = Absolute Value(x=w355) -> (abs(x)=w352:dbl)
                          n152 = Greater Or Equal?(x=w352, y=500.0) -> (x >= y?=w350:bool)
                        }
                      }
                      n153 = call "Find_Number_LineMARVIN.vi"("Test Paragraph"="4.4", "TableIn"=w334) -> ("Line number"=w331:i32)  [unwired: 3 in, 3 out]
                      n154 = And(x=w333, y=w332) -> (x .and. y?=w323:bool)
                      "VenableDirectionResult" <- w323
                      n155 = call "PassOrFail (SubVI).vi"("String Res"="", "index (row)"=w331, "Data in"=-3.0, "Pass?Fail"=w323, "Table in"=w334) -> ("error out"=w329:errorcluster)  [unwired: 6 in]
                      n156 = property on="Test Failed" class="Bool (strict)"() -> ("Value"=w322:bool)  [unwired: 2 in, 2 out]
                      n157 = case shown="False" w322 {
                        tunnel: w323 -> [w348 _]
                        frame False {
                          n158 = Not(x=w348) -> (.not. x?=w347:bool)
                          n159 = property on="Test Failed" class="Bool (strict)"("Value"=w347) -> ()  [unwired: 2 in, 2 out]
                        }
                        frame True {
                        }
                      }
                      n160 = property class="Bool (strict)"(reference=w330, error in=w329) -> ("Value"=w346:bool)  [unwired: 2 out]
                      n161 = Select(t=T12."Stop", s=w346, f=T12."Stop") -> (s? t:f=w343:T12)
                    }
                    frame "FullSpeed2" {
                      n162 = Concatenate Strings(w371, "\nFull speed operation " ("string")) -> (w357:string)
                      n163 = Equal?(x=w356, y=u8 95) -> (x = y?=w366:bool)
                      n164 = Select(t=u16 15100, s=w366, f=u16 12100 ("y")) -> (s? t:f=w380:u16)
                      n165 = call "CANSendMotorSpeed.vi"("Remote"=TRUE, "Motor Speed RPM"=w380, "UUT"=w381, "CAN Cluster in"=w385) -> ("error out"=w378:errorcluster)  [unwired: 7 in]
                      n166 = call "Write panel message (SubVI).vi"("Stop BurnIn"=w358, 4:"rpm"=w376, 5:"rpm"=TRUE ("rpm"), "PrintTime"=FALSE, "Stop"=w360, "error in (no error)"=w378, "Time to wait"=0.2, "Strin"=w357, "String in"=w359) -> ("error out"=w363:errorcluster)  [unwired: 2 in]
                      n167 = flat-sequence {
                        tunnel: w363 -> [w392]
                        tunnel: [w392] -> w362
                        tunnel: [w391] -> w361
                        frame #0 {
                          n168 = call <vilib>:"High Resolution Relative Seconds.vi"() -> ("relative seconds"=w391:dbl)
                        }
                      }
                      n169 = Select(t=15000.0, s=w366, f=11500.0) -> (s? t:f=w365:dbl)
                      n170 = Select(t=50.0, s=w366, f=24.0) -> (s? t:f=w364:dbl)
                      n171 = while {
                        tunnel: w376 -> [w394]
                        tunnel: w362 -> [w422]
                        tunnel: [w402] -> w373
                        tunnel: w365 -> [w415]
                        tunnel: w364 -> [w414]
                        tunnel: w361 -> [w410]
                        tunnel: w360 -> [w400]
                        tunnel: w359 -> [w401]
                        tunnel: w358 -> [w398]
                        tunnel: w357 -> [w397]
                        stop <- w412 stop-if-true
                        n172 = call <vilib>:"High Resolution Relative Seconds.vi"() -> ("relative seconds"=w411:dbl)
                        n173 = Subtract(x=w411, y=w410) -> (x-y=w409:dbl)
                        n174 = property class="DigNum (strict)"(reference=w394, error in=w422) -> (error out=w421:errorcluster, "Value"=w416:dbl)  [unwired: 1 out]
                        "FullSpeed2 Speed" <- w416
                        n175 = Greater Or Equal?(x=w409, y=120.0) -> (x >= y?=w407:bool)
                        n176 = Greater Or Equal?(x=w416, y=w415) -> (x >= y?=w406:bool)
                        n177 = property on="VISA Tester" class="VISAName"(error in=w421) -> (error out=w420:errorcluster, "Value"=w419:refnum<visa-resource-name>)  [unwired: 1 in, 1 out]
                        n178 = property class="Bool (strict)"(reference=w400) -> ("Value"=w405:bool)  [unwired: 1 in, 2 out]
                        n179 = call "GetADCTester (SubVI).vi"("error in (no error)"=w420, "GetADCTester"=T13."Current", "TimeToGet"=5, "VISA Refnum in"=w419) -> ("error out"=w417:errorcluster, "ADCValOutput Single"=w413:dbl)  [unwired: 5 in, 1 out]
                        "FullSpeed2 Current" <- w413
                        n180 = Greater Or Equal?(x=w413, y=w414) -> (x >= y?=w403:bool)
                        n181 = And(x=w406, y=w403) -> (x .and. y?=w404:bool)
                        n182 = Compound Arithmetic op=OR(w405, w407, w404) -> (w412:bool)
                        n183 = call "Write panel message (SubVI).vi"("Stop BurnIn"=w398, 4:"rpm"=w394, 5:"rpm"=TRUE ("rpm"), "PrintTime"=FALSE, "Stop"=w400, "error in (no error)"=w417, "Time to wait"=0.2, "Strin"=w397, "String in"=w401) -> ("error out"=w402:errorcluster)  [unwired: 2 in]
                      }
                      n184 = property class="Bool (strict)"(reference=w360, error in=w373) -> ("Value"=w390:bool)  [unwired: 2 out]
                      n185 = Select(t=T12."Stop", s=w390, f=T12."Result") -> (s? t:f=w387:T12)
                    }
                    frame "MD[1]=1" {
                      n186 = Concatenate Strings(w449, "\nSet Parameters MD[1]=1" ("Strin")) -> (w438:string)
                      n187 = property on="VISA Tester" class="VISAName"() -> ("Value"=w454:refnum<visa-resource-name>)  [unwired: 2 in, 2 out]
                      n188 = call "TesterOption (SubVI).vi"("2 Options"=FALSE, "On/Off"=FALSE, "Tester Option"=T11."Venable", "VISA Refnum in"=w454) -> ("error out"=w455:errorcluster, "VISA Refnum out"=w445:refnum<visa-resource-name>)  [unwired: 6 in]
                      n189 = call "CANSendMotorSpeed.vi"("Remote"=TRUE, "error in (no error)"=w455, "Motor Speed RPM"=u16 0, "UUT"=w439, "CAN Cluster in"=w460) -> ("error out"=w457:errorcluster)  [unwired: 6 in]
                      n190 = call "Write panel message (SubVI).vi"("Stop BurnIn"=w440, 4:"rpm"=w428, 5:"rpm"=TRUE ("rpm"), "PrintTime"=TRUE, "Stop"=w430, "error in (no error)"=w457, "Time to wait"=10.0, "Strin"=w438, "String in"=w441) -> ("error out"=w427:errorcluster)  [unwired: 2 in]
                      n191 = while {
                        tunnel: w428 -> [w472]
                        tunnel: w427 -> [w469]
                        tunnel: [w468] -> w426
                        stop <- w470 continue-if-true
                        n192 = property class="DigNum (strict)"(reference=w472, error in=w469) -> (error out=w468:errorcluster, "Value"=w471:dbl)  [unwired: 1 out]
                        n193 = Not Equal To 0?(x=w471) -> (x != 0?=w470:bool)
                      }
                      n194 = property on="VISA Marvin" class="VISAName"(error in=w426) -> (error out=w456:errorcluster, "Value"=w462:refnum<visa-resource-name>)  [unwired: 1 in, 1 out]
                      n195 = call "SerialMarvinSendGet.vi"("error in (no error)"=w456, "Clear Log"=FALSE, "write buffer"="EP=1\r\nMD[1]=1\r\n", "VISA resource name"=w462) -> ("error out"=w444:errorcluster)  [unwired: 6 in, 1 out]
                      n196 = call "TesterOption (SubVI).vi"("error in (no error)"=w444, "On/Off"=FALSE, "Tester Option"=T11."Power", "VISA Refnum in"=w445) -> ("error out"=w442:errorcluster, "VISA Refnum out"=w431:refnum<visa-resource-name>)  [unwired: 6 in]
                      n197 = call "Write panel message (SubVI).vi"("Stop BurnIn"=w440, 4:"rpm"=w428, 5:"rpm"=TRUE ("rpm"), "PrintTime"=TRUE, "Stop"=w430, "error in (no error)"=w442, "Time to wait"=25.0, "Strin"=w438, "String in"=w441) -> ("error out"=w432:errorcluster)  [unwired: 2 in]
                      n198 = call "TesterOption (SubVI).vi"("error in (no error)"=w432, "On/Off"=TRUE, "Tester Option"=T11."Venable", "VISA Refnum in"=w431) -> ("error out"=w429:errorcluster)  [unwired: 6 in, 1 out]
                      n199 = call "Time Delay8"("error in (no error)"=w429) -> ("error out"=w424:errorcluster)  [unwired: 10 in]
                      n200 = property class="Bool (strict)"(reference=w430, error in=w424) -> ("Value"=w467:bool)  [unwired: 2 out]
                      n201 = Select(t=T12."Stop", s=w467, f=T12."FullSpeed2") -> (s? t:f=w466:T12)
                    }
                    frame "FullSpeed1" {
                      n202 = Concatenate Strings(w492, "\nFull speed operation " ("string")) -> (w477:string)
                      n203 = Equal?(x=w473, y=u8 95) -> (x = y?=w490:bool)
                      n204 = flat-sequence {
                        tunnel: w483 -> [w509]
                        tunnel: [w509] -> w482
                        tunnel: [w508] -> w481
                        frame #0 {
                          n205 = call <vilib>:"High Resolution Relative Seconds.vi"() -> ("relative seconds"=w508:dbl)
                        }
                      }
                      n206 = Select(t=u16 15100, s=w490, f=u16 12100 ("y")) -> (s? t:f=w497:u16)
                      n207 = call "CANSendMotorSpeed.vi"("Remote"=TRUE, "Motor Speed RPM"=w497, "UUT"=w498, "CAN Cluster in"=w502) -> ("error out"=w495:errorcluster)  [unwired: 7 in]
                      n208 = call "Write panel message (SubVI).vi"("Stop BurnIn"=w478, 4:"rpm"=w494, 5:"rpm"=TRUE ("rpm"), "PrintTime"=FALSE, "Stop"=w480, "error in (no error)"=w495, "Time to wait"=0.2, "Strin"=w477, "String in"=w479) -> ("error out"=w483:errorcluster)  [unwired: 2 in]
                      n209 = Select(t=13700.0, s=w490, f=11500.0) -> (s? t:f=w485:dbl)
                      n210 = Select(t=58.0, s=w490, f=33.0) -> (s? t:f=w484:dbl)
                      n211 = while {
                        tunnel: w494 -> [w511]
                        tunnel: w482 -> [w539]
                        tunnel: [w519] -> w493
                        tunnel: w485 -> [w531]
                        tunnel: w484 -> [w528]
                        tunnel: w481 -> [w526]
                        tunnel: w480 -> [w517]
                        tunnel: w479 -> [w518]
                        tunnel: w478 -> [w515]
                        tunnel: w477 -> [w514]
                        stop <- w533 stop-if-true
                        n212 = property class="DigNum (strict)"(reference=w511, error in=w539) -> (error out=w538:errorcluster, "Value"=w532:dbl)  [unwired: 1 out]
                        "FullSpeed1 Speed" <- w532
                        n213 = call <vilib>:"High Resolution Relative Seconds.vi"() -> ("relative seconds"=w527:dbl)
                        n214 = Subtract(x=w527, y=w526) -> (x-y=w525:dbl)
                        n215 = Greater Or Equal?(x=w525, y=120.0) -> (x >= y?=w523:bool)
                        n216 = Greater Or Equal?(x=w532, y=w531) -> (x >= y?=w530:bool)
                        n217 = property on="VISA Tester" class="VISAName"(error in=w538) -> (error out=w537:errorcluster, "Value"=w536:refnum<visa-resource-name>)  [unwired: 1 in, 1 out]
                        n218 = call "GetADCTester (SubVI).vi"("error in (no error)"=w537, "GetADCTester"=T13."Current", "TimeToGet"=5, "VISA Refnum in"=w536) -> ("error out"=w534:errorcluster, "ADCValOutput Single"=w529:dbl)  [unwired: 5 in, 1 out]
                        "FullSpeed1 Current" <- w529
                        n219 = Greater Or Equal?(x=w529, y=w528) -> (x >= y?=w520:bool)
                        n220 = And(x=w520, y=w530) -> (x .and. y?=w521:bool)
                        n221 = property class="Bool (strict)"(reference=w517) -> ("Value"=w522:bool)  [unwired: 1 in, 2 out]
                        n222 = call "Write panel message (SubVI).vi"("Stop BurnIn"=w515, 4:"rpm"=w511, 5:"rpm"=TRUE ("rpm"), "PrintTime"=FALSE, "Stop"=w517, "error in (no error)"=w534, "Time to wait"=0.2, "Strin"=w514, "String in"=w518) -> ("error out"=w519:errorcluster)  [unwired: 2 in]
                        n223 = Compound Arithmetic op=OR(w522, w521, w523) -> (w533:bool)
                      }
                      n224 = property class="Bool (strict)"(reference=w480, error in=w493) -> ("Value"=w507:bool)  [unwired: 2 out]
                      n225 = Select(t=T12."Stop", s=w507, f=T12."MD[1]=1") -> (s? t:f=w504:T12)
                    }
                    frame "MD[1]=0" {
                      n226 = Concatenate Strings(w566, "\nSet Parameters MD[1]=0" ("Strin")) -> (w555:string)
                      n227 = property on="VISA Tester" class="VISAName"() -> ("Value"=w572:refnum<visa-resource-name>)  [unwired: 2 in, 2 out]
                      n228 = call "TesterOption (SubVI).vi"("2 Options"=FALSE, "On/Off"=FALSE, "Tester Option"=T11."Venable", "VISA Refnum in"=w572) -> ("error out"=w573:errorcluster, "VISA Refnum out"=w562:refnum<visa-resource-name>)  [unwired: 6 in]
                      n229 = call "CANSendMotorSpeed.vi"("Remote"=TRUE, "error in (no error)"=w573, "Motor Speed RPM"=u16 0, "UUT"=w556, "CAN Cluster in"=w578) -> ("error out"=w575:errorcluster)  [unwired: 6 in]
                      n230 = call "Write panel message (SubVI).vi"("Stop BurnIn"=w557, 4:"rpm"=w552, 5:"rpm"=FALSE ("rpm"), "PrintTime"=FALSE, "Stop"=w546, "error in (no error)"=w575, "Time to wait"=0.2, "Strin"=w555, "String in"=w558) -> ("error out"=w569:errorcluster)  [unwired: 2 in]
                      n231 = property on="VISA Marvin" class="VISAName"(error in=w569) -> (error out=w574:errorcluster, "Value"=w580:refnum<visa-resource-name>)  [unwired: 1 in, 1 out]
                      n232 = call "SerialMarvinSendGet.vi"("error in (no error)"=w574, "Clear Log"=FALSE, "write buffer"="EP=1\r\nMD[1]=0\r\n", "VISA resource name"=w580) -> ("error out"=w561:errorcluster)  [unwired: 6 in, 1 out]
                      n233 = call "TesterOption (SubVI).vi"("2 Options"=FALSE, "error in (no error)"=w561, "On/Off"=FALSE, "Tester Option"=T11."Power", "VISA Refnum in"=w562) -> ("error out"=w559:errorcluster, "VISA Refnum out"=w547:refnum<visa-resource-name>)  [unwired: 5 in]
                      n234 = call "Write panel message (SubVI).vi"("Stop BurnIn"=w557, 4:"rpm"=w552, 5:"rpm"=FALSE ("rpm"), "PrintTime"=TRUE, "Stop"=w546, "error in (no error)"=w559, "Time to wait"=25.0, "Strin"=w555, "String in"=w558) -> ("error out"=w548:errorcluster)  [unwired: 2 in]
                      n235 = call "TesterOption (SubVI).vi"("2 Options"=FALSE, "error in (no error)"=w548, "On/Off"=TRUE, "Tester Option"=T11."Venable", "VISA Refnum in"=w547) -> ("error out"=w545:errorcluster)  [unwired: 5 in, 1 out]
                      n236 = call "Time Delay4"("error in (no error)"=w545) -> ("error out"=w541:errorcluster)  [unwired: 10 in]
                      n237 = property class="Bool (strict)"(reference=w546, error in=w541) -> ("Value"=w585:bool)  [unwired: 2 out]
                      n238 = Select(t=T12."Stop", s=w585, f=T12."FullSpeed1") -> (s? t:f=w584:T12)
                    }
                  }
                }
                n239 = flat-sequence {
                  tunnel: [enum16{"Stop", "Direction", "Venable", "Start"}."Stop"] -> w297
                  tunnel: w296 -> [_]
                  frame #0 {
                  }
                }
              }
              frame "Venable" {
                n240 = call "Find_Number_LineMARVIN.vi"("Test Paragraph"="4.1", "TableIn"=w590) -> ("Line number"=w598:i32)  [unwired: 3 in, 3 out]
                n241 = for {
                  tunnel: u16[] [5000, 0, 5000] -> [w629] mode=indexing
                  tunnel: bool[] [TRUE, FALSE, TRUE] -> [w624] mode=indexing
                  tunnel: w598 -> [w630]
                  tunnel: w597 -> [w628]
                  tunnel: w596 -> [w627]
                  tunnel: w595 -> [w615]
                  tunnel: w594 -> [w619]
                  tunnel: w592 -> [w618]
                  tunnel: w593 -> [w617]
                  tunnel: w590 -> [w611]
                  tunnel: w589 -> [w609]
                  tunnel: [w608] -> w588 mode=indexing
                  i -> [w631]
                  w633 = 200.0 ("y")
                  n242 = call "CANSendMotorSpeed.vi"("Remote"=TRUE, "Motor Speed RPM"=u16 5000, "UUT"=w627, "CAN Cluster in"=w628) -> ("error out"=w623:errorcluster)  [unwired: 7 in]
                  n243 = property on="VISA Tester" class="VISAName"() -> ("Value"=w622:refnum<visa-resource-name>)  [unwired: 2 in, 2 out]
                  n244 = Add(x=w630, y=w631) -> (x+y=w612:i32)
                  n245 = call "TesterOption (SubVI).vi"("error in (no error)"=w623, "On/Off"=w624, "Tester Option"=T11."Venable", "VISA Refnum in"=w622) -> ("error out"=w621:errorcluster)  [unwired: 6 in, 1 out]
                  n246 = call "Write panel message (SubVI).vi"("Stop BurnIn"=w617, 4:"rpm"=w615, 5:"rpm"=TRUE ("rpm"), "PrintTime"=TRUE, "Stop"=w618, "error in (no error)"=w621, "Time to wait"=15.0, "Strin"=w609, "String in"=w619) -> ("error out"=w620:errorcluster)  [unwired: 2 in]
                  n247 = property class="DigNum (strict)"(reference=w615, error in=w620) -> ("Value"=w610:dbl)  [unwired: 2 out]
                  n248 = Add(x=w629, y=w633) -> (x+y=w635:dbl)
                  n249 = Subtract(x=w629, y=w633) -> (x-y=w634:dbl)
                  n250 = In Range and Coerce(upper limit=w635, x=w610, lower limit=w634) -> (In Range?=w608:bool)  [unwired: 1 out]
                  n251 = call "PassOrFail (SubVI).vi"("index (row)"=w612, "Data in"=w610, "Pass?Fail"=w608, "Table in"=w611) -> ()  [unwired: 7 in, 1 out]
                }
                n252 = property class="Bool (strict)"(reference=w592) -> ("Value"=w605:bool)  [unwired: 1 in, 2 out]
                n253 = property on="Test Failed" class="Bool (strict)"() -> ("Value"=w586:bool)  [unwired: 2 in, 2 out]
                n254 = And Array Elements(Boolean array=w588) -> (logical AND=w587:bool)
                "VenableResult" <- w587
                n255 = case shown="False" w586 {
                  tunnel: w587 -> [w607 _]
                  frame False {
                    n256 = Not(x=w607) -> (.not. x?=w606:bool)
                    n257 = property on="Test Failed" class="Bool (strict)"("Value"=w606) -> ()  [unwired: 2 in, 2 out]
                  }
                  frame True {
                  }
                }
                n258 = Select(t=enum16{"Stop", "Direction", "Venable", "Start"}."Stop", s=w605, f=enum16{"Stop", "Direction", "Venable", "Start"}."Direction") -> (s? t:f=w591:enum16{"Stop", "Direction", "Venable", "Start"})
              }
              frame "Start" {
                w654 = "4" ("Test Paragraph")
                n259 = property class="Str"(reference=w645, "Value"=w636) -> (reference out=w655:refnum<vi>, error out=w642:errorcluster)  [unwired: 1 in]
                n260 = call "Table_ScrollaBarMarvin.vi"("error in"=w642, "Line to focus"=w654, "reference in"=w646) -> ("error out"=w651:errorcluster)  [unwired: 2 out]
                n261 = call "Reset old test Values (SubVI).vi"("error in"=w651, "Atr in"=w646, "Test Paragraph"=w654) -> ("error out"=w650:errorcluster)  [unwired: 8 in]
                n262 = property on="VISA Tester" class="VISAName"(error in=w650) -> (error out=w649:errorcluster, "Value"=w648:refnum<visa-resource-name>)  [unwired: 1 in, 1 out]
                n263 = property class="Bool (strict)"(reference=w639) -> ("Value"=w659:bool)  [unwired: 1 in, 2 out]
                n264 = call "TesterOption (SubVI).vi"("error in (no error)"=w649, "On/Off"=TRUE, "Tester Option"=T11."Venable", "VISA Refnum in"=w648) -> ("error out"=w647:errorcluster)  [unwired: 6 in, 1 out]
                n265 = Select(t=enum16{"Stop", "Direction", "Venable", "Start"}."Stop", s=w659, f=enum16{"Stop", "Direction", "Venable", "Start"}."Venable") -> (s? t:f=w643:enum16{"Stop", "Direction", "Venable", "Start"})
                n266 = call "Write panel message (SubVI).vi"("Stop BurnIn"=w638, 4:"rpm"=w637, 5:"rpm"=FALSE ("rpm"), "PrintTime"=FALSE, "Stop"=w639, "error in (no error)"=w647, "Time to wait"=0.2, "Strin"=w636, "String in"=w655) -> ()  [unwired: 2 in, 1 out]
              }
            }
          }
        }
        frame "Speed Command" {
          w664 = "5. Speed Command Test in process..." ("Value")
          w661 = "5" ("Test Paragraph")
          n267 = control-ref of="Pannel User Message"() -> (w676:refnum<vi>)
          n268 = property class="Str"(reference=w676, error in=w675, "Value"=w664) -> (error out=w674:errorcluster)  [unwired: 1 out]
          n269 = call "Table_ScrollaBarMarvin.vi"("error in"=w674, "Line to focus"=w661, "reference in"=w660) -> ("error out"=w677:errorcluster)  [unwired: 2 out]
          n270 = property class="Tbl (strict)"(reference=w660, error in=w677) -> (error out=w679:errorcluster, "Value"=w680:string[][])  [unwired: 1 out]
          n271 = Index Array(array=w680, index (col)=0 ("disabled index (col)")) -> (element=w681:string[])  [unwired: 1 in]
          n272 = call "Find_Number_Line.vi"("error in"=w679, "Test Paragraph"=w661, "Row Headers[]"=w681) -> ("error out"=w662:errorcluster, "Line number"=w665:i32)  [unwired: 1 out]
          n273 = call "Reset old test Values (SubVI).vi"("error in"=w662, "Atr in"=w660, "Test Paragraph"=w661) -> ()  [unwired: 8 in, 1 out]
          n274 = control-ref of="Pannel User Message"() -> (w669:refnum<vi>)
          n275 = control-ref of="Stop Burn-in"() -> (w673:refnum<vi>)
          n276 = control-ref of="Config_CANAT"() -> (w670:refnum<vi>)
          n277 = control-ref of="Motor Speed RPM"() -> (w671:refnum<vi>)
          n278 = control-ref of="UUT"() -> (w672:refnum<vi>)
          n279 = control-ref of="Stop Button"() -> (w667:refnum<vi>)
          n280 = control-ref of="ATR"() -> (w668:refnum<vi>)
          n281 = property on="UUT" class="DigNum (strict)"() -> ("Value"=w663:u8)  [unwired: 2 in, 2 out]
          n282 = while {
            shift-right: [w693] -> _
            shift-left: enum16{"Stop", "StopTime", "Speeds", "Start"}."Start" -> [w694]
            tunnel: w667 -> [w692]
            tunnel: w668 -> [w691]
            tunnel: w669 -> [w690]
            tunnel: w670 -> [w689]
            tunnel: w671 -> [w688]
            tunnel: w672 -> [w687]
            tunnel: w673 -> [w686]
            tunnel: w665 -> [w685]
            tunnel: w664 -> [w684]
            tunnel: w663 -> [w682]
            stop <- w683 stop-if-true
            n283 = case shown="\"Start\"" w694 {
              tunnel: [w698 w728 w772 w818] -> w693
              tunnel: w692 -> [_ w723 w776 w816]
              tunnel: w691 -> [_ w713 w780 _]
              tunnel: w690 -> [_ w724 w777 _]
              tunnel: w689 -> [w696 w726 w779 _]
              tunnel: w688 -> [_ w721 w774 _]
              tunnel: w687 -> [w697 w725 w771 _]
              tunnel: w686 -> [_ w722 w775 _]
              tunnel: w685 -> [_ _ w781 _]
              tunnel: w684 -> [_ _ w778 _]
              tunnel: [w695 w727 w773 FALSE ("Value")] -> w683
              tunnel: w682 -> [_ _ w764 _]
              frame "Stop", Default {
                n284 = flat-sequence {
                  tunnel: w697 -> [w701]
                  tunnel: w696 -> [w700]
                  tunnel: [enum16{"Stop", "StopTime", "Speeds", "Start"}."Stop"] -> w698
                  tunnel: [TRUE] -> w695
                  frame #0 {
                    n285 = call "CANSendMotorSpeed.vi"("Remote"=TRUE, "Motor Speed RPM"=u16 0, "UUT"=w701, "CAN Cluster in"=w700) -> ("error out"=w706:errorcluster)  [unwired: 7 in]
                    n286 = property on="VISA Tester" class="VISAName"() -> ("Value"=w707:refnum<visa-resource-name>)  [unwired: 2 in, 2 out]
                    n287 = call "TesterOption (SubVI).vi"("2 Options"=FALSE, "error in (no error)"=w706, "On/Off"=FALSE, "Tester Option"=T11."Power", "VISA Refnum in"=w707) -> ()  [unwired: 5 in, 2 out]
                  }
                  frame #1 {
                  }
                }
              }
              frame "StopTime" {
                n288 = call "Table_ScrollaBarMarvin.vi"("Line to focus"="6", "reference in"=w713) -> ("error out"=w714:errorcluster)  [unwired: 1 in, 2 out]
                n289 = call "CANSendMotorSpeed.vi"("Remote"=TRUE, "error in (no error)"=w714, "Motor Speed RPM"=u16 0, "UUT"=w725, "CAN Cluster in"=w726) -> ("error out"=w732:errorcluster)  [unwired: 6 in]
                n290 = flat-sequence {
                  tunnel: [w760] -> w731
                  tunnel: w732 -> [w759]
                  tunnel: [w759] -> w733
                  frame #0 {
                    n291 = call <vilib>:"High Resolution Relative Seconds.vi"() -> ("relative seconds"=w760:dbl)
                  }
                }
                n292 = while {
                  tunnel: [w755] -> w727
                  tunnel: w724 -> [w753]
                  tunnel: w723 -> [w752]
                  tunnel: w722 -> [w750]
                  tunnel: w721 -> [w749]
                  tunnel: "6. Stop Time Test in process...\n" ("Value") -> [w737]
                  tunnel: [w745] -> w711
                  tunnel: w733 -> [w757]
                  tunnel: [w746] -> w719
                  tunnel: w731 -> [w756]
                  tunnel: [w744] -> w715
                  stop <- w736 stop-if-true
                  n293 = call "Write panel message (SubVI).vi"("Stop BurnIn"=w750, 4:"rpm"=w749, 5:"rpm"=TRUE ("rpm"), "PrintTime"=FALSE, "Stop"=w752, "error in (no error)"=w757, "Time to wait"=0.1, "Strin"=w737, "String in"=w753) -> ("error out"=w754:errorcluster)  [unwired: 2 in]
                  n294 = control-ref of="Motor Speed RPM"() -> (w743:refnum<vi>)
                  n295 = property class="DigNum (strict)"(reference=w743, error in=w754) -> (error out=w746:errorcluster, "Value"=w742:dbl)  [unwired: 1 out]
                  n296 = call <vilib>:"High Resolution Relative Seconds.vi"() -> ("relative seconds"=w740:dbl)
                  n297 = property class="Bool (strict)"(reference=w752) -> ("Value"=w755:bool)  [unwired: 1 in, 2 out]
                  n298 = Subtract(x=w740, y=w756) -> (x-y=w744:dbl)
                  n299 = Greater Or Equal?(x=w744, y=50.0) -> (x >= y?=w738:bool)
                  n300 = Less Or Equal?(x=w742, y=0.0) -> (x <= y?=w745:bool)
                  n301 = Compound Arithmetic op=OR(w745, w738, w755) -> (w736:bool)
                }
                "StopTimeResult" <- w711
                n302 = call "Find_Number_LineMARVIN.vi"("Test Paragraph"="6.1", "TableIn"=w713) -> ("Line number"=w716:i32)  [unwired: 3 in, 3 out]
                n303 = property on="Test Failed" class="Bool (strict)"() -> ("Value"=w710:bool)  [unwired: 2 in, 2 out]
                n304 = call "PassOrFail (SubVI).vi"("index (row)"=w716, "error in (no error)"=w719, "Data in"=w715, "Pass?Fail"=w711, "Table in"=w713) -> ("error out"=w718:errorcluster)  [unwired: 6 in]
                n305 = flat-sequence {
                  tunnel: [enum16{"Stop", "StopTime", "Speeds", "Start"}."Stop"] -> w728
                  tunnel: w718 -> [_]
                  frame #0 {
                  }
                }
                n306 = case shown="False" w710 {
                  tunnel: w711 -> [w735 _]
                  frame False {
                    n307 = Not(x=w735) -> (.not. x?=w734:bool)
                    n308 = property on="Test Failed" class="Bool (strict)"("Value"=w734) -> ()  [unwired: 2 in, 2 out]
                  }
                  frame True {
                  }
                }
              }
              frame "Speeds" {
                n309 = Equal?(x=w764, y=u8 95) -> (x = y?=w769:bool)
                n310 = Select(t=u16[] [6000, 11500, 15100], s=w769, f=u16[] [6000, 9000, 12100]) -> (s? t:f=w766:u16[])
                n311 = for {
                  tunnel: w766 -> [w809] mode=indexing
                  tunnel: w781 -> [w802]
                  tunnel: w780 -> [w801]
                  tunnel: w771 -> [w800]
                  tunnel: w779 -> [w799]
                  tunnel: w778 -> [w798]
                  tunnel: w777 -> [w797]
                  tunnel: w776 -> [w796]
                  tunnel: w775 -> [w794]
                  tunnel: w774 -> [w792]
                  tunnel: [w790] -> w773
                  tunnel: [w789] -> w765
                  tunnel: [w788] -> w763 mode=indexing
                  i -> [w808]
                  stop <- w790 stop-if-true
                  w810 = 200.0 ("y")
                  n312 = Increment(x=w808) -> (x+1=w807:i32)
                  n313 = Add(x=w802, y=w807) -> (x+y=w803:i32)
                  n314 = call "CANSendMotorSpeed.vi"("Remote"=TRUE, "Motor Speed RPM"=w809, "UUT"=w800, "CAN Cluster in"=w799) -> ("error out"=w814:errorcluster)  [unwired: 7 in]
                  n315 = control-ref of="Motor Speed RPM"() -> (w815:refnum<vi>)
                  n316 = call "Write panel message (SubVI).vi"("Stop BurnIn"=w794, 4:"rpm"=w792, 5:"rpm"=TRUE ("rpm"), "PrintTime"=TRUE, "Stop"=w796, "error in (no error)"=w814, "Time to wait"=25.0 ("Delay Time (sec)"), "Strin"=w798, "String in"=w797) -> ("error out"=w806:errorcluster)  [unwired: 2 in]
                  n317 = property class="DigNum (strict)"(reference=w815, error in=w806) -> (error out=w813:errorcluster, "Value"=w791:dbl)  [unwired: 1 out]
                  n318 = property class="Bool (strict)"(reference=w796) -> ("Value"=w790:bool)  [unwired: 1 in, 2 out]
                  n319 = Add(x=w809, y=w810) -> (x+y=w812:dbl)
                  n320 = Subtract(x=w809, y=w810) -> (x-y=w811:dbl)
                  n321 = In Range and Coerce(upper limit=w812, x=w791, lower limit=w811) -> (In Range?=w788:bool)  [unwired: 1 out]
                  n322 = call "PassOrFail (SubVI).vi"("index (row)"=w803, "error in (no error)"=w813, "Data in"=w791, "Pass?Fail"=w788, "Table in"=w801) -> ("error out"=w789:errorcluster)  [unwired: 6 in]
                }
                n323 = flat-sequence {
                  tunnel: w773 -> [w787]
                  tunnel: [w785] -> w772
                  tunnel: w765 -> [_]
                  frame #0 {
                    n324 = Select(t=enum16{"Stop", "StopTime", "Speeds", "Start"}."Stop", s=w787, f=enum16{"Stop", "StopTime", "Speeds", "Start"}."StopTime") -> (s? t:f=w785:enum16{"Stop", "StopTime", "Speeds", "Start"})
                  }
                }
                n325 = property on="Test Failed" class="Bool (strict)"() -> ("Value"=w761:bool)  [unwired: 2 in, 2 out]
                n326 = And Array Elements(Boolean array=w763) -> (logical AND=w762:bool)
                "SpeedResult" <- w762
                n327 = case shown="False" w761 {
                  tunnel: w762 -> [w783 _]
                  frame False {
                    n328 = Not(x=w783) -> (.not. x?=w782:bool)
                    n329 = property on="Test Failed" class="Bool (strict)"("Value"=w782) -> ()  [unwired: 2 in, 2 out]
                  }
                  frame True {
                  }
                }
              }
              frame "Start" {
                n330 = property on="VISA Tester" class="VISAName"() -> ("Value"=w826:refnum<visa-resource-name>)  [unwired: 2 in, 2 out]
                n331 = call "TesterOption (SubVI).vi"("2 Options"=FALSE, "On/Off"=TRUE, "Tester Option"=T11."Venable", "VISA Refnum in"=w826) -> ("error out"=w817:errorcluster)  [unwired: 6 in, 1 out]
                n332 = property class="Bool (strict)"(reference=w816, error in=w817) -> ("Value"=w822:bool)  [unwired: 2 out]
                n333 = Select(t=enum16{"Stop", "StopTime", "Speeds", "Start"}."Stop", s=w822, f=enum16{"Stop", "StopTime", "Speeds", "Start"}."Speeds") -> (s? t:f=w818:enum16{"Stop", "StopTime", "Speeds", "Start"})
              }
            }
          }
        }
        frame "Stop Time" {
          w830 = "3. Motor Temperature test in process..." ("Value")
          w828 = "3" ("Test Paragraph")
          n334 = control-ref of="Pannel User Message"() -> (w838:refnum<vi>)
          n335 = property class="Str"(reference=w838, error in=w837, "Value"=w830) -> (error out=w836:errorcluster)  [unwired: 1 out]
          n336 = call "Table_ScrollaBarMarvin.vi"("error in"=w836, "Line to focus"=w828, "reference in"=w827) -> ("error out"=w840:errorcluster)  [unwired: 2 out]
          n337 = property class="Tbl (strict)"(reference=w827, error in=w840) -> (reference out=w833:refnum<vi>, error out=w842:errorcluster, "Value"=w843:string[][])
          n338 = Index Array(array=w843, index (col)=0 ("disabled index (col)")) -> (element=w844:string[])  [unwired: 1 in]
          n339 = call "Find_Number_LineMARVIN.vi"("Test Paragraph"=w828, "error in"=w842, "TableIn"=w827, "Row Headers[]"=w844) -> ("error out"=w839:errorcluster, "Line number"=w832:i32)  [unwired: 1 in, 2 out]
          n340 = call "Reset old test Values (SubVI).vi"("error in"=w839, "Atr in"=w827, "Test Paragraph"=w828) -> ("error out"=w829:errorcluster)  [unwired: 8 in]
          n341 = property on="Status" class="Bool (strict)"(error in=w829) -> (error out=w834:errorcluster, "Value"=w835:bool)  [unwired: 1 in, 1 out]
          n342 = case shown="True" w835 {
            selector: w835 -> [w848 _]
            tunnel: w834 -> [w850 _]
            tunnel: w833 -> [w847 _]
            tunnel: w832 -> [w846 w853]
            tunnel: w831 -> [_ w858]
            tunnel: w830 -> [_ w854]
            frame False {
              n343 = flat-sequence {
                tunnel: w850 -> [w851]
                tunnel: [w851] -> w849
                frame #0 {
                  n344 = One Button Dialog(message="Please establish RS connection.") -> ()  [unwired: 1 in, 1 out]
                }
              }
              n345 = Increment(x=w846) -> (x+1=w845:i32)
              n346 = call "PassOrFail (SubVI).vi"("index (row)"=w845, "error in (no error)"=w849, "Pass?Fail"=w848, "Table in"=w847) -> ()  [unwired: 7 in, 1 out]
            }
            frame True {
              n347 = control-ref of="Stop Burn-in"() -> (w860:refnum<vi>)
              n348 = control-ref of="Pannel User Message"() -> (w862:refnum<vi>)
              n349 = control-ref of="Config_CANAT"() -> (w856:refnum<vi>)
              n350 = control-ref of="ATR"() -> (w863:refnum<vi>)
              n351 = control-ref of="Motor Speed RPM"() -> (w864:refnum<vi>)
              n352 = control-ref of="UUT"() -> (w855:refnum<vi>)
              n353 = control-ref of="Stop Button"() -> (w861:refnum<vi>)
              n354 = property on="VISA Tester" class="VISAName"() -> ("Value"=w857:refnum<visa-resource-name>)  [unwired: 2 in, 2 out]
              n355 = while {
                shift-right: [w868] -> _
                shift-left: T14."Start" -> [w878]
                tunnel: w860 -> [w877]
                tunnel: w861 -> [w876]
                tunnel: w862 -> [w875]
                tunnel: w863 -> [w874]
                tunnel: w864 -> [w873]
                tunnel: w858 -> [w872]
                tunnel: w857 -> [w871]
                tunnel: w856 -> [w870]
                tunnel: w855 -> [w869]
                tunnel: w854 -> [w866]
                tunnel: w853 -> [w865]
                stop <- w867 stop-if-true
                n356 = case shown="\"TA[5]\"" w878 {
                  tunnel: w877 -> [_ w902 w963]
                  tunnel: w876 -> [_ w894 w965]
                  tunnel: w875 -> [_ w903 w967]
                  tunnel: w874 -> [_ w892 _]
                  tunnel: w873 -> [_ w901 w962]
                  tunnel: w872 -> [_ w906 _]
                  tunnel: w871 -> [w881 w905 w956]
                  tunnel: w870 -> [_ _ w973]
                  tunnel: w869 -> [_ _ w972]
                  tunnel: [w879 w895 w958] -> w868
                  tunnel: [w880 FALSE FALSE] -> w867
                  tunnel: w866 -> [_ w904 _]
                  tunnel: w865 -> [_ w891 _]
                  frame "Stop", Default {
                    n357 = flat-sequence {
                      tunnel: w881 -> [w882]
                      tunnel: [TRUE] -> w880
                      tunnel: [T14."Stop"] -> w879
                      frame #0 {
                        n358 = call "TesterOption (SubVI).vi"("2 Options"=FALSE, "On/Off"=FALSE, "Tester Option"=T11."Power", "VISA Refnum in"=w882) -> ()  [unwired: 6 in, 2 out]
                      }
                      frame #1 {
                      }
                    }
                  }
                  frame "TA[5]" {
                    w907 = T17 [enum."60C", enum."90C", enum."120C"] items=["K15", "K16", "K17", "Venable", "Firmeware", "Fan", "Power", "120C", "110C", "100C", "90C", "80C", "70C", "60C", "50C", "40C", "30C", "25C", "20C", "10C", "0C"]
                    n359 = for {
                      tunnel: w907 -> [w933] mode=indexing
                      tunnel: w906 -> [w932]
                      tunnel: w905 -> [w931]
                      tunnel: w904 -> [w930]
                      tunnel: w903 -> [w929]
                      tunnel: w894 -> [w928]
                      tunnel: w902 -> [w927]
                      tunnel: w901 -> [w926]
                      tunnel: dbl[] [60.0, 90.0, 120.0] -> [w916] mode=indexing
                      tunnel: [w915] -> w893
                      tunnel: w892 -> [w922]
                      tunnel: w891 -> [w921]
                      tunnel: [w910] -> w890 mode=indexing
                      i -> [w919]
                      w914 = 3.0 ("y")
                      n360 = for {
                        N: 5 -> [_]
                        tunnel: w933 -> [w935]
                        tunnel: w932 -> [w951]
                        tunnel: w931 -> [w947]
                        tunnel: w930 -> [w945]
                        tunnel: w929 -> [w944]
                        tunnel: w928 -> [w943]
                        tunnel: w927 -> [w941]
                        tunnel: w926 -> [w938]
                        tunnel: [w937] -> w925 mode=indexing
                        tunnel: [w936] -> w923
                        n361 = call "TesterOption (SubVI).vi"("2 Options"=FALSE, "On/Off"=TRUE, "Tester Option"=w935, "VISA Refnum in"=w947) -> ("error out"=w948:errorcluster)  [unwired: 6 in, 1 out]
                        n362 = call "Write panel message (SubVI).vi"("Stop BurnIn"=w941, 4:"rpm"=w938, 5:"rpm"=FALSE ("rpm"), "PrintTime"=FALSE, "Stop"=w943, "error in (no error)"=w948, "Time to wait"=1.0, "Strin"=w945, "String in"=w944) -> ("error out"=w946:errorcluster)  [unwired: 2 in]
                        n363 = call "SerialMarvinSendGet.vi"("error in (no error)"=w946, "write buffer"="TA[2]\r\n", "VISA resource name"=w951) -> ("error out"=w936:errorcluster, "read buffer"=w949:string)  [unwired: 7 in]
                        n364 = Fract/Exp String To Number(string=w949) -> (number=w937:dbl)  [unwired: 3 in, 1 out]
                      }
                      n365 = Increment(x=w919) -> (x+1=w918:i32)
                      n366 = Add Array Elements(numeric array=w925) -> (sum=w924:dbl)
                      n367 = Add(x=w916, y=w914) -> (x+y=w913:dbl)
                      n368 = Subtract(x=w916, y=w914) -> (x-y=w912:dbl)
                      n369 = Divide(x=w924, y=5.0) -> (x/y=w911:dbl)
                      n370 = In Range and Coerce(upper limit=w913, x=w911, lower limit=w912) -> (In Range?=w910:bool)  [unwired: 1 out]
                      n371 = Add(x=w921, y=w918) -> (x+y=w920:i32)
                      n372 = call "PassOrFail (SubVI).vi"("index (row)"=w920, "error in (no error)"=w923, "Data in"=w911, "Pass?Fail"=w910, "Table in"=w922) -> ("error out"=w915:errorcluster)  [unwired: 6 in]
                    }
                    n373 = property class="Bool (strict)"(reference=w894, error in=w893) -> ("Value"=w899:bool)  [unwired: 2 out]
                    n374 = Select(t=T14."Stop", s=w899, f=T14."Stop") -> (s? t:f=w895:T14)
                    n375 = property on="Test Failed" class="Bool (strict)"() -> ("Value"=w888:bool)  [unwired: 2 in, 2 out]
                    n376 = And Array Elements(Boolean array=w890) -> (logical AND=w889:bool)
                    "MotorTempResult" <- w889
                    n377 = case shown="False" w888 {
                      tunnel: w889 -> [w908 _]
                      frame False {
                        n378 = Not(x=w908) -> (.not. x?=w909:bool)
                        n379 = property on="Test Failed" class="Bool (strict)"("Value"=w909) -> ()  [unwired: 2 in, 2 out]
                      }
                      frame True {
                      }
                    }
                  }
                  frame "Start" {
                    n380 = call "Write panel message (SubVI).vi"("Stop BurnIn"=w963, 4:"rpm"=w962, 5:"rpm"=FALSE ("rpm"), "PrintTime"=FALSE, "Stop"=w965, "Time to wait"=0.1, "Strin"="3. Motor Temperature test in process...\nInitialization state...", "String in"=w967) -> ("error out"=w968:errorcluster)  [unwired: 3 in]
                    n381 = call "TesterOption (SubVI).vi"("2 Options"=FALSE, "error in (no error)"=w968, "On/Off"=FALSE, "Tester Option"=T11."Venable", "VISA Refnum in"=w956) -> ("error out"=w970:errorcluster)  [unwired: 5 in, 1 out]
                    n382 = call "CANSendMotorSpeed.vi"("Remote"=TRUE, "error in (no error)"=w970, "Motor Speed RPM"=u16 0, "UUT"=w972, "CAN Cluster in"=w973) -> ("error out"=w955:errorcluster)  [unwired: 6 in]
                    n383 = property class="Bool (strict)"(reference=w965, error in=w955) -> ("Value"=w977:bool)  [unwired: 2 out]
                    n384 = Select(t=T14."Stop", s=w977, f=T14."TA[5]") -> (s? t:f=w958:T14)
                  }
                }
              }
            }
          }
        }
        frame "Temp Control" {
          w980 = "7. Temperature controle test in process..." ("Value")
          w978 = "7" ("Test Paragraph")
          n385 = control-ref of="Pannel User Message"() -> (w992:refnum<vi>)
          n386 = property class="Str"(reference=w992, error in=w991, "Value"=w980) -> (error out=w990:errorcluster)  [unwired: 1 out]
          n387 = control-ref of="Pannel User Message"() -> (w985:refnum<vi>)
          n388 = control-ref of="Motor Speed RPM"() -> (w983:refnum<vi>)
          n389 = control-ref of="Stop Button"() -> (w987:refnum<vi>)
          n390 = control-ref of="ATR"() -> (w986:refnum<vi>)
          n391 = control-ref of="Config_CANAT"() -> (w984:refnum<vi>)
          n392 = control-ref of="UUT"() -> (w982:refnum<vi>)
          n393 = control-ref of="Stop Burn-in"() -> (w981:refnum<vi>)
          n394 = call "Table_ScrollaBarMarvin.vi"("error in"=w990, "Line to focus"=w978, "reference in"=w993) -> ("error out"=w989:errorcluster)  [unwired: 2 out]
          n395 = call "Reset old test Values (SubVI).vi"("error in"=w989, "Atr in"=w993, "Test Paragraph"=w978) -> ("error out"=w979:errorcluster)  [unwired: 8 in]
          n396 = while {
            tunnel: w979 -> [w1005]
            shift-right: [w1003] -> _
            shift-left: enum16{"Stop", "Algorithm", "Start"}."Start" -> [w1004]
            tunnel: w987 -> [w1002]
            tunnel: w986 -> [w1001]
            tunnel: w985 -> [w1000]
            tunnel: w984 -> [w999]
            tunnel: w983 -> [w998]
            tunnel: w982 -> [w997]
            tunnel: w981 -> [w995]
            tunnel: w980 -> [w994]
            stop <- w996 stop-if-true
            n397 = case shown="\"Algorithm\"" w1004 {
              tunnel: w1005 -> [_ _ w1126]
              tunnel: [w1006 w1026 w1115] -> w1003
              tunnel: w1002 -> [_ w1037 w1119]
              tunnel: w1001 -> [_ w1033 _]
              tunnel: w1000 -> [_ w1038 _]
              tunnel: w999 -> [w1009 _ w1111]
              tunnel: w998 -> [_ w1034 _]
              tunnel: w997 -> [w1008 _ w1110]
              tunnel: [w1007 FALSE FALSE] -> w996
              tunnel: w995 -> [_ w1036 _]
              tunnel: w994 -> [_ w1035 _]
              frame "Stop", Default {
                n398 = flat-sequence {
                  tunnel: w1009 -> [w1014]
                  tunnel: w1008 -> [w1011]
                  tunnel: [TRUE] -> w1007
                  tunnel: [enum16{"Stop", "Algorithm", "Start"}."Stop"] -> w1006
                  frame #0 {
                    n399 = property on="VISA Tester" class="VISAName"() -> ("Value"=w1018:refnum<visa-resource-name>)  [unwired: 2 in, 2 out]
                    n400 = call "TesterOption (SubVI).vi"("2 Options"=FALSE, "On/Off"=FALSE, "Tester Option"=T11."Power", "VISA Refnum in"=w1018) -> ("error out"=w1012:errorcluster)  [unwired: 6 in, 1 out]
                    n401 = call "CANSendMotorSpeed.vi"("Remote"=TRUE, "error in (no error)"=w1012, "Motor Speed RPM"=u16 0, "UUT"=w1011, "CAN Cluster in"=w1014) -> ()  [unwired: 6 in, 1 out]
                  }
                  frame #1 {
                  }
                  frame #2 {
                  }
                }
              }
              frame "Algorithm" {
                # "Speed Goal"
                # "Speed Ind"
                # "Temp Goal"
                # "50 Deg"
                n402 = for {
                  tunnel: w1038 -> [w1067]
                  tunnel: w1037 -> [w1066]
                  tunnel: w1036 -> [w1065]
                  tunnel: w1035 -> [w1064]
                  tunnel: w1034 -> [w1063]
                  tunnel: w1033 -> [w1050]
                  tunnel: string[] ["7.1", "7.3", "7.5", "7.7", "7.9"] -> [w1048] mode=indexing
                  shift-right: [w1060] -> _
                  shift-left: 1202.0 ("Rt") -> [w1061]
                  tunnel: dbl[] [68.0, 68.0, 88.0, 80.0, 60.0] -> [w1059] mode=indexing
                  tunnel: dbl[] [6000.0, 11500.0, 15100.0, 11500.0, 6000.0] -> [w1058] mode=indexing
                  tunnel: dbl[] [6000.0, 6400.0, 11700.0, 14600.0, 11000.0] -> [w1057] mode=indexing
                  tunnel: [w1045] -> w1027
                  tunnel: [w1044] -> w1023 mode=indexing
                  tunnel: [w1043] -> w1024 mode=indexing
                  i -> [w1046]
                  stop <- w1062 stop-if-true
                  n403 = call <vilib>:"High Resolution Relative Seconds.vi"() -> ("relative seconds"=w1056:dbl)
                  n404 = while {
                    tunnel: w1067 -> [w1095]
                    tunnel: w1066 -> [w1087]
                    tunnel: w1065 -> [w1094]
                    tunnel: w1064 -> [w1073]
                    tunnel: w1063 -> [w1096]
                    shift-right: [w1092] -> w1060
                    shift-left: w1061 -> [w1091]
                    tunnel: w1046 -> [w1093]
                    tunnel: w1059 -> [w1090]
                    tunnel: w1058 -> [w1089]
                    tunnel: w1057 -> [w1088]
                    tunnel: w1056 -> [w1084]
                    tunnel: [w1079] -> w1051
                    tunnel: [w1078] -> w1043
                    tunnel: [w1077] -> w1049
                    tunnel: [w1076] -> w1044
                    tunnel: [w1075] -> w1047
                    stop <- w1085 stop-if-true
                    n405 = call "DegToDAC (SubVI).vi"("R2"=0.0, "Rt"=w1091) -> ("error out"=w1103:errorcluster, "output array"=w1104:u8[])  [unwired: 8 in]
                    n406 = call <vilib>:"High Resolution Relative Seconds.vi"() -> ("relative seconds"=w1083:dbl)
                    n407 = property on="VISA Tester" class="VISAName"() -> ("Value"=w1106:refnum<visa-resource-name>)  [unwired: 2 in, 2 out]
                    n408 = Byte Array To String(unsigned byte array=w1104) -> (string=w1105:string)
                    n409 = Subtract(x=w1084, y=w1083) -> (x-y=w1082:dbl)
                    n410 = VISA Write(VISA resource name=w1106, write buffer=w1105, error in (no error)=w1103) -> (error out=w1102:errorcluster)  [unwired: 2 out]
                    n411 = Greater Or Equal?(x=w1082, y=120.0) -> (x >= y?=w1080:bool)
                    n412 = call <vilib>:"Clear Errors.vi"("error in (no error)"=w1102) -> ("error out"=w1101:errorcluster)  [unwired: 5 in, 1 out]
                    n413 = control-ref of="Ambient Temperature"() -> (w1074:refnum<vi>)
                    n414 = property class="DigNum (strict)"(reference=w1074) -> ("Value"=w1072:dbl)  [unwired: 1 in, 2 out]
                    n415 = property class="Bool (strict)"(reference=w1087) -> ("Value"=w1086:bool)  [unwired: 1 in, 2 out]
                    n416 = Number To Fractional String(number=w1072, precision (6)=i16 2) -> (F-format string=w1069:string)  [unwired: 2 in]
                    n417 = Concatenate Strings(w1073, "\nAmbient  Temp. [C]: " ("string"), w1069) -> (w1068:string)
                    n418 = call "Write panel message (SubVI).vi"("Stop BurnIn"=w1094, 4:"rpm"=w1096, 5:"rpm"=TRUE ("rpm"), "PrintTime"=TRUE, "Stop"=w1087, "error in (no error)"=w1101, "Time to wait"=3.0, "Strin"=w1068, "String in"=w1095) -> ("error out"=w1100:errorcluster)  [unwired: 2 in]
                    n419 = call "TempAlgoTest (SubVI).vi"("Temp"=w1074, "Speed Ind"=w1088, "Motor Speed RPM"=w1096, "Round"=w1093, "Temp Up In"=w1091, "error in (no error)"=w1100, "String in"=w1095, "Temp Goal"=w1090, "Stop"=w1087, "Speed Goal"=w1089, "Stop BurnIn"=w1094, "Strin"=w1068) -> (14:"Speed Pass/Fail"=w1078:bool, "Temp  Pass/Fail"=w1077:dbl, "Temp Up Out"=w1092:dbl, 17:"Speed Pass/Fail"=w1079:dbl, "Temp Pass/Fail"=w1076:bool, "error out"=w1075:errorcluster)  [unwired: 2 in]
                    n420 = Compound Arithmetic op=OR(w1080, w1078, w1086) -> (w1085:bool)
                  }
                  n421 = property class="Bool (strict)"(reference=w1066) -> ("Value"=w1062:bool)  [unwired: 1 in, 2 out]
                  n422 = call "Find_Number_LineMARVIN.vi"("Test Paragraph"=w1048, "error in"=w1047, "TableIn"=w1050) -> ("error out"=w1052:errorcluster, "Line number"=w1055:i32)  [unwired: 2 in, 2 out]
                  n423 = Increment(x=w1055) -> (x+1=w1054:i32)
                  n424 = call "PassOrFail (SubVI).vi"("index (row)"=w1054, "error in (no error)"=w1052, "Data in"=w1049, "Pass?Fail"=w1044, "Table in"=w1050) -> ("error out"=w1053:errorcluster)  [unwired: 6 in]
                  n425 = call "PassOrFail (SubVI).vi"("index (row)"=w1055, "error in (no error)"=w1053, "Data in"=w1051, "Pass?Fail"=w1043, "Table in"=w1050) -> ("error out"=w1045:errorcluster)  [unwired: 6 in]
                }
                n426 = property on="Test Failed" class="Bool (strict)"() -> ("Value"=w1021:bool)  [unwired: 2 in, 2 out]
                n427 = Build Array (concatenate)(w1024, w1023) -> (w1025:bool[])
                n428 = flat-sequence {
                  tunnel: w1027 -> [_]
                  tunnel: [enum16{"Stop", "Algorithm", "Start"}."Stop"] -> w1026
                  frame #0 {
                  }
                }
                n429 = And Array Elements(Boolean array=w1025) -> (logical AND=w1022:bool)
                "TempControlResult" <- w1022
                n430 = case shown="False" w1021 {
                  tunnel: w1022 -> [w1040 _]
                  frame False {
                    n431 = Not(x=w1040) -> (.not. x?=w1041:bool)
                    n432 = property on="Test Failed" class="Bool (strict)"("Value"=w1041) -> ()  [unwired: 2 in, 2 out]
                  }
                  frame True {
                  }
                }
              }
              frame "Start" {
                n433 = property on="VISA Tester" class="VISAName"() -> ("Value"=w1125:refnum<visa-resource-name>)  [unwired: 2 in, 2 out]
                n434 = call "TesterOption (SubVI).vi"("On/Off 2"=TRUE, "Tester Option 2"=T11."Venable", "2 Options"=TRUE, "error in (no error)"=w1126, "On/Off"=TRUE, "Tester Option"=T11."K16", "VISA Refnum in"=w1125) -> ("error out"=w1113:errorcluster)  [unwired: 3 in, 1 out]
                n435 = call "CANSendMotorSpeed.vi"("Remote"=FALSE, "error in (no error)"=w1113, "Motor Speed RPM"=u16 0, "UUT"=w1110, "CAN Cluster in"=w1111) -> ("error out"=w1112:errorcluster)  [unwired: 6 in]
                n436 = property class="Bool (strict)"(reference=w1119, error in=w1112) -> ("Value"=w1118:bool)  [unwired: 2 out]
                n437 = Select(t=enum16{"Stop", "Algorithm", "Start"}."Stop", s=w1118, f=enum16{"Stop", "Algorithm", "Start"}."Algorithm") -> (s? t:f=w1115:enum16{"Stop", "Algorithm", "Start"})
              }
            }
          }
        }
        frame "Burn in" {
          n438 = control-ref of="Stop Button"() -> (w1130:refnum<vi>)
          n439 = control-ref of="Pannel User Message"() -> (w1133:refnum<vi>)
          n440 = control-ref of="ATR"() -> (w1129:refnum<vi>)
          n441 = control-ref of="Config_CANAT"() -> (w1132:refnum<vi>)
          n442 = control-ref of="UUT"() -> (w1131:refnum<vi>)
          n443 = control-ref of="Stop Burn-in"() -> (w1128:refnum<vi>)
          n444 = property on="UUT" class="DigNum (strict)"() -> ("Value"=w1127:u8)  [unwired: 2 in, 2 out]
          n445 = while {
            tunnel: w1133 -> [w1144]
            tunnel: w1129 -> [w1143]
            tunnel: w1132 -> [w1142]
            tunnel: w1131 -> [w1141]
            tunnel: w1130 -> [w1140]
            shift-right: [w1139] -> _
            shift-left: T15."Start" -> [w1146]
            shift-right: [w1145] -> _
            shift-left: _ -> [w1137]
            tunnel: w1128 -> [w1136]
            tunnel: w1127 -> [w1135]
            stop <- w1138 stop-if-true
            n446 = case shown="\"Stop\", Default" w1146 {
              tunnel: [w1149 w1184 w1255 w1287 w1320 w1359] -> w1145
              tunnel: w1144 -> [_ w1176 _ _ _ w1358]
              tunnel: w1143 -> [_ w1179 w1228 w1274 w1306 w1345]
              tunnel: w1142 -> [_ w1175 _ _ _ w1357]
              tunnel: w1141 -> [_ w1172 _ _ _ w1336]
              tunnel: w1140 -> [_ _ w1257 w1289 w1324 w1351]
              tunnel: [w1147 T15."Stop" w1258 w1290 w1325 w1347] -> w1139
              tunnel: [w1148 FALSE FALSE FALSE FALSE FALSE] -> w1138
              tunnel: w1137 -> [w1149 w1184 w1255 w1287 w1320 _]
              tunnel: w1136 -> [_ _ _ _ _ w1341]
              tunnel: w1135 -> [_ w1164 w1219 w1266 w1298 w1335]
              frame "Stop", Default {
                n447 = flat-sequence {
                  tunnel: [TRUE] -> w1148
                  tunnel: [T15."Stop"] -> w1147
                  frame #0 {
                    n448 = property on="VISA Tester" class="VISAName"() -> ("Value"=w1153:refnum<visa-resource-name>)  [unwired: 2 in, 2 out]
                    n449 = call "TesterOption (SubVI).vi"("On/Off"=FALSE, "Tester Option"=T11."Power", "VISA Refnum in"=w1153) -> ("error out"=w1150:errorcluster)  [unwired: 7 in, 1 out]
                    n450 = property on="Stop Burn-in" class="Bool (strict)"(error in=w1150, "Visible"=FALSE) -> ()  [unwired: 1 in, 2 out]
                  }
                  frame #1 {
                  }
                }
              }
              frame "BurnIn" {
                w1168 = FALSE ("Stop Burn-in")
                n451 = control-ref of="Motor Speed RPM"() -> (w1178:refnum<vi>)
                n452 = control-ref of="Stop Button"() -> (w1177:refnum<vi>)
                n453 = property on="Stop Burn-in" class="Bool (strict)"("Visible"=TRUE) -> (error out=w1180:errorcluster)  [unwired: 2 in, 1 out]
                n454 = Equal?(x=w1164, y=u8 95) -> (x = y?=w1161:bool)
                n455 = Select(t="8. " ("Test Paragraph"), s=w1161, f="7. " ("Test Paragraph")) -> (s? t:f=w1160:string)
                n456 = Select(t="8.4" ("Test Paragraph"), s=w1161, f="7.4" ("Test Paragraph")) -> (s? t:f=w1165:string)
                n457 = call "Find_Number_LineMARVIN.vi"("Test Paragraph"=w1165, "error in"=w1180, "TableIn"=w1179) -> ("error out"=w1182:errorcluster, "Line number"=w1183:i32)  [unwired: 2 in, 2 out]
                n458 = Select(t=u16 15100, s=w1161, f=u16 12100 ("y")) -> (s? t:f=w1170:u16)
                n459 = for {
                  tunnel: w1182 -> [w1206]
                  tunnel: dbl[] [600.0, 600.0, 600.0] -> [w1210] mode=indexing
                  tunnel: w1183 -> [w1215]
                  tunnel: w1179 -> [w1205]
                  tunnel: w1178 -> [w1204]
                  tunnel: w1177 -> [w1203]
                  tunnel: w1176 -> [w1202]
                  tunnel: w1175 -> [w1198]
                  tunnel: w1172 -> [w1197]
                  tunnel: w1170 -> [w1196]
                  tunnel: [w1194] -> w1169
                  tunnel: w1160 -> [w1191]
                  tunnel: [w1190] -> w1159 mode=indexing
                  i -> [w1212]
                  n460 = call "CANSendMotorSpeed.vi"("Remote"=TRUE, "error in (no error)"=w1206, "Motor Speed RPM"=w1196, "UUT"=w1197, "CAN Cluster in"=w1198) -> ("error out"=w1200:errorcluster)  [unwired: 6 in]
                  n461 = control-ref of="Stop Burn-in"() -> (w1201:refnum<vi>)
                  n462 = Concatenate Strings(w1191, "Burn-in test in process..." ("Strin")) -> (w1192:string)
                  n463 = Add(x=w1215, y=w1212) -> (x+y=w1211:i32)
                  n464 = call "Write panel message (SubVI).vi"("Stop BurnIn"=w1201, 4:"rpm"=w1204, 5:"rpm"=TRUE ("rpm"), "PrintTime"=TRUE, "Stop"=w1203, "error in (no error)"=w1200, "Time to wait"=w1210, "Strin"=w1192, "String in"=w1202) -> ("error out"=w1207:errorcluster)  [unwired: 2 in]
                  n465 = control-ref of="Power transistor Heat sink Temp."() -> (w1216:refnum<vi>)
                  n466 = property on="MaxBurnInTempVal" class="DigNum (strict)"() -> ("Value"=w1214:dbl)  [unwired: 2 in, 2 out]
                  n467 = property class="DigNum (strict)"(reference=w1216, error in=w1207) -> (error out=w1195:errorcluster, "Value"=w1213:dbl)  [unwired: 1 out]
                  n468 = Less Or Equal?(x=w1213, y=w1214) -> (x <= y?=w1190:bool)
                  n469 = call "PassOrFail (SubVI).vi"("index (row)"=w1211, "error in (no error)"=w1195, "Data in"=w1213, "Pass?Fail"=w1190, "Table in"=w1205) -> ("error out"=w1194:errorcluster)  [unwired: 6 in]
                }
                n470 = property on="Test Failed" class="Bool (strict)"() -> ("Value"=w1157:bool)  [unwired: 2 in, 2 out]
                n471 = And Array Elements(Boolean array=w1159) -> (logical AND=w1158:bool)
                "BurnResult" <- w1158
                n472 = case shown="False" w1157 {
                  tunnel: w1158 -> [w1188 _]
                  frame False {
                    n473 = Not(x=w1188) -> (.not. x?=w1189:bool)
                    n474 = property on="Test Failed" class="Bool (strict)"("Value"=w1189) -> ()  [unwired: 2 in, 2 out]
                  }
                  frame True {
                  }
                }
                n475 = property on="Stop Burn-in" class="Bool (strict)"(error in=w1169, "Value"=w1168, "Visible"=w1168) -> ()  [unwired: 1 in, 2 out]
              }
              frame "Ambient Temp" {
                w1233 = 2 ("disabled index (col)")
                n476 = control-ref of="Power transistor Heat sink Temp."() -> (w1243:refnum<vi>)
                n477 = Equal?(x=w1219, y=u8 95) -> (x = y?=w1222:bool)
                n478 = Select(t="8.3" ("Test Paragraph"), s=w1222, f="7.3" ("Test Paragraph")) -> (s? t:f=w1220:string)
                n479 = call "Find_Number_LineMARVIN.vi"("Test Paragraph"=w1220, "TableIn"=w1228) -> ("error out"=w1254:errorcluster, "Line number"=w1234:i32)  [unwired: 3 in, 2 out]
                n480 = property class="DigNum (strict)"(reference=w1243, error in=w1254) -> (error out=w1245:errorcluster, "Value"=w1235:dbl)  [unwired: 1 out]
                n481 = Select(t=25.0 ("y"), s=w1222, f=25.0 ("y")) -> (s? t:f=w1244:dbl)
                n482 = Select(t=13.0 ("y"), s=w1222, f=13.0) -> (s? t:f=w1246:dbl)
                n483 = Add(x=w1244, y=w1246) -> (x+y=w1253:dbl)
                n484 = Subtract(x=w1244, y=w1246) -> (x-y=w1252:dbl)
                n485 = In Range and Coerce(upper limit=w1253, x=w1235, lower limit=w1252) -> (In Range?=w1218:bool)  [unwired: 1 out]
                "BurnTemp" <- w1218
                n486 = call "PassOrFail (SubVI).vi"("index (row)"=w1234, "error in (no error)"=w1245, "Data in"=w1235, "Pass?Fail"=w1218, "Table in"=w1228) -> ("error out"=w1225:errorcluster)  [unwired: 6 in]
                n487 = property class="Tbl (strict)"(reference=w1228, error in=w1225) -> (reference out=w1227:refnum<vi>, error out=w1242:errorcluster, "Value"=w1241:string[][])
                n488 = Add(x=w1235, y=25.0) -> (x+y=w1226:dbl)
                "MaxBurnInTempVal" <- w1226
                n489 = Number To Fractional String(number=w1226, precision (6)=i16 0) -> (F-format string=w1240:string)  [unwired: 2 in]
                n490 = Concatenate Strings("< " ("string"), w1240) -> (w1229:string)
                n491 = Increment(x=w1234) -> (x+1=w1232:i32)
                n492 = Increment(x=w1232) -> (x+1=w1231:i32)
                n493 = Increment(x=w1231) -> (x+1=w1230:i32)
                n494 = property on="Test Failed" class="Bool (strict)"() -> ("Value"=w1217:bool)  [unwired: 2 in, 2 out]
                n495 = Replace Array Subset(array=w1241, new element #1=w1229, index (row) #1=w1232, index (col) #1=w1233, new element #2=w1229, index (row) #2=w1231, index (col) #2=w1233, new element #3=w1229, index (row) #3=w1230, index (col) #3=w1233) -> (w1239:string[][])
                n496 = case shown="False" w1217 {
                  tunnel: w1218 -> [w1262 _]
                  frame False {
                    n497 = Not(x=w1262) -> (.not. x?=w1263:bool)
                    n498 = property on="Test Failed" class="Bool (strict)"("Value"=w1263) -> ()  [unwired: 2 in, 2 out]
                  }
                  frame True {
                  }
                }
                n499 = property class="Tbl (strict)"(reference=w1227, error in=w1242, "Value"=w1239) -> (error out=w1224:errorcluster)  [unwired: 1 out]
                n500 = property class="Bool (strict)"(reference=w1257, error in=w1224) -> ("Value"=w1261:bool)  [unwired: 2 out]
                n501 = Select(t=T15."Stop", s=w1261, f=T15."BurnIn") -> (s? t:f=w1258:T15)
              }
              frame "MotorSpeed" {
                n502 = control-ref of="Motor Speed RPM"() -> (w1272:refnum<vi>)
                n503 = Equal?(x=w1266, y=u8 95) -> (x = y?=w1269:bool)
                n504 = Select(t="8.2" ("Test Paragraph"), s=w1269, f="7.2" ("Test Paragraph")) -> (s? t:f=w1267:string)
                n505 = call "Find_Number_LineMARVIN.vi"("Test Paragraph"=w1267, "TableIn"=w1274) -> ("error out"=w1286:errorcluster, "Line number"=w1277:i32)  [unwired: 3 in, 2 out]
                n506 = property class="DigNum (strict)"(reference=w1272, error in=w1286) -> (error out=w1275:errorcluster, "Value"=w1276:dbl)  [unwired: 1 out]
                n507 = Select(t=15100.0 ("y"), s=w1269, f=12100.0 ("y")) -> (s? t:f=w1273:dbl)
                n508 = Select(t=200.0 ("y"), s=w1269, f=200.0) -> (s? t:f=w1278:dbl)
                n509 = Add(x=w1273, y=w1278) -> (x+y=w1285:dbl)
                n510 = Subtract(x=w1273, y=w1278) -> (x-y=w1284:dbl)
                n511 = In Range and Coerce(upper limit=w1285, x=w1276, lower limit=w1284) -> (In Range?=w1265:bool)  [unwired: 1 out]
                "BurnSpeed" <- w1265
                n512 = call "PassOrFail (SubVI).vi"("index (row)"=w1277, "error in (no error)"=w1275, "Data in"=w1276, "Pass?Fail"=w1265, "Table in"=w1274) -> ("error out"=w1271:errorcluster)  [unwired: 6 in]
                n513 = property class="Bool (strict)"(reference=w1289, error in=w1271) -> ("Value"=w1293:bool)  [unwired: 2 out]
                n514 = property on="Test Failed" class="Bool (strict)"() -> ("Value"=w1264:bool)  [unwired: 2 in, 2 out]
                n515 = Select(t=T15."Stop", s=w1293, f=T15."Ambient Temp") -> (s? t:f=w1290:T15)
                n516 = case shown="False" w1264 {
                  tunnel: w1265 -> [w1294 _]
                  frame False {
                    n517 = Not(x=w1294) -> (.not. x?=w1295:bool)
                    n518 = property on="Test Failed" class="Bool (strict)"("Value"=w1295) -> ()  [unwired: 2 in, 2 out]
                  }
                  frame True {
                  }
                }
              }
              frame "DC Current Measure" {
                n519 = property on="VISA Tester" class="VISAName"() -> (error out=w1318:errorcluster, "Value"=w1322:refnum<visa-resource-name>)  [unwired: 2 in, 1 out]
                n520 = call "GetADCTester (SubVI).vi"("error in (no error)"=w1318, "GetADCTester"=T13."Current", "TimeToGet"=10, "VISA Refnum in"=w1322) -> ("error out"=w1319:errorcluster, "ADCValOutput Single"=w1305:dbl)  [unwired: 5 in, 1 out]
                n521 = Equal?(x=w1298, y=u8 95) -> (x = y?=w1302:bool)
                n522 = Select(t="8.1" ("Test Paragraph"), s=w1302, f="7.1" ("Test Paragraph")) -> (s? t:f=w1300:string)
                n523 = call "Find_Number_LineMARVIN.vi"("Test Paragraph"=w1300, "error in"=w1319, "TableIn"=w1306) -> ("error out"=w1317:errorcluster, "Line number"=w1307:i32)  [unwired: 2 in, 2 out]
                n524 = Select(t=50.0 ("y"), s=w1302, f=28.0 ("y")) -> (s? t:f=w1309:dbl)
                n525 = Select(t=5.0 ("y"), s=w1302, f=3.0) -> (s? t:f=w1308:dbl)
                n526 = Add(x=w1309, y=w1308) -> (x+y=w1316:dbl)
                n527 = Subtract(x=w1309, y=w1308) -> (x-y=w1315:dbl)
                n528 = In Range and Coerce(upper limit=w1316, x=w1305, lower limit=w1315) -> (In Range?=w1297:bool)  [unwired: 1 out]
                "BurnDC" <- w1297
                n529 = property on="Test Failed" class="Bool (strict)"() -> ("Value"=w1296:bool)  [unwired: 2 in, 2 out]
                n530 = call "PassOrFail (SubVI).vi"("index (row)"=w1307, "error in (no error)"=w1317, "Data in"=w1305, "Pass?Fail"=w1297, "Table in"=w1306) -> ("error out"=w1304:errorcluster)  [unwired: 6 in]
                n531 = property class="Bool (strict)"(reference=w1324, error in=w1304) -> ("Value"=w1328:bool)  [unwired: 2 out]
                n532 = Select(t=T15."Stop", s=w1328, f=T15."MotorSpeed") -> (s? t:f=w1325:T15)
                n533 = case shown="False" w1296 {
                  tunnel: w1297 -> [w1329 _]
                  frame False {
                    n534 = Not(x=w1329) -> (.not. x?=w1330:bool)
                    n535 = property on="Test Failed" class="Bool (strict)"("Value"=w1330) -> ()  [unwired: 2 in, 2 out]
                  }
                  frame True {
                  }
                }
              }
              frame "Start" {
                w1332 = ". Burn-in test in process...\nFull Speed Operation" ("Value")
                n536 = Equal?(x=w1335, y=u8 95) -> (x = y?=w1337:bool)
                n537 = Select(t="8" ("Test Paragraph"), s=w1337, f="7" ("Test Paragraph")) -> (s? t:f=w1331:string)
                n538 = Concatenate Strings(w1331, w1332) -> (w1333:string)
                n539 = property class="Str"(reference=w1358, "Value"=w1333) -> (reference out=w1355:refnum<vi>, error out=w1340:errorcluster)  [unwired: 1 in]
                n540 = call "Find_Number_LineMARVIN.vi"("Test Paragraph"=w1331, "error in"=w1340, "TableIn"=w1345) -> ("error out"=w1365:errorcluster, "Line number"=w1366:i32)  [unwired: 2 in, 2 out]
                n541 = call "Table_ScrollaBarMarvin.vi"("error in"=w1365, "Line to focus"=w1331, "reference in"=w1345) -> ("error out"=w1367:errorcluster)  [unwired: 2 out]
                n542 = Select(t=u16 15100 ("y"), s=w1337, f=u16 12100 ("y")) -> (s? t:f=w1372:u16)
                n543 = call "Reset old test Values (SubVI).vi"("error in"=w1367, "Atr in"=w1345, "Test Paragraph"=w1331) -> ("error out"=w1368:errorcluster)  [unwired: 8 in]
                n544 = Increment(x=w1366) -> (x+1=w1359:i32)
                n545 = property on="VISA Tester" class="VISAName"(error in=w1368) -> (error out=w1369:errorcluster, "Value"=w1370:refnum<visa-resource-name>)  [unwired: 1 in, 1 out]
                n546 = call "TesterOption (SubVI).vi"("2 Options"=FALSE, "error in (no error)"=w1369, "On/Off"=TRUE, "Tester Option"=T11."Venable", "VISA Refnum in"=w1370) -> ("error out"=w1371:errorcluster)  [unwired: 5 in, 1 out]
                n547 = call "CANSendMotorSpeed.vi"("Remote"=TRUE, "error in (no error)"=w1371, "Motor Speed RPM"=w1372, "UUT"=w1336, "CAN Cluster in"=w1357) -> ("error out"=w1356:errorcluster)  [unwired: 6 in]
                n548 = control-ref of="Motor Speed RPM"() -> (w1344:refnum<vi>)
                n549 = call "Write panel message (SubVI).vi"("Stop BurnIn"=w1341, 4:"rpm"=w1344, 5:"rpm"=TRUE ("rpm"), "PrintTime"=TRUE, "Stop"=w1351, "error in (no error)"=w1356, "Time to wait"=50.0, "Strin"=w1332, "String in"=w1355) -> ("error out"=w1343:errorcluster)  [unwired: 2 in]
                n550 = property class="Bool (strict)"(reference=w1351, error in=w1343) -> ("Value"=w1350:bool)  [unwired: 2 out]
                n551 = Select(t=T15."Stop", s=w1350, f=T15."DC Current Measure") -> (s? t:f=w1347:T15)
              }
            }
          }
        }
        frame "Visual Inspec" {
          n552 = property on="VISA Tester" class="VISAName"() -> ("Value"=w1386:refnum<visa-resource-name>)  [unwired: 2 in, 2 out]
          n553 = call "TesterOption (SubVI).vi"("2 Options"=FALSE, "error in (no error)"=w1387, "On/Off"=FALSE, "Tester Option"=T11."Power", "VISA Refnum in"=w1386) -> ("error out"=w1382:errorcluster)  [unwired: 5 in, 1 out]
          n554 = local read "UUT"() -> (w1375:u8)
          n555 = Equal?(x=w1375, y=u8 95) -> (x = y?=w1373:bool)
          n556 = case shown="False" w1373 {
            tunnel: w1388 -> [w1392 w1396]
            tunnel: w1382 -> [w1391 w1395]
            tunnel: [w1389 w1394] -> w1380
            tunnel: [w1390 w1393] -> w1378
            frame False {
              n557 = call "VisualInspectionAHU.vi"("error in (no error)"=w1391, "TableRef"=w1392) -> ("error out"=w1390:errorcluster, "VisualInspectionResult"=w1389:bool)  [unwired: 8 in]
            }
            frame True {
              n558 = call "VisualInspectionEBAY.vi"("error in (no error)"=w1395, "TableRef"=w1396) -> ("error out"=w1393:errorcluster, "VisualInspectionResult"=w1394:bool)  [unwired: 8 in]
            }
          }
          "VisualInspectionResult" <- w1380
          n559 = property on="Test Failed" class="Bool (strict)"(error in=w1378) -> (error out=w1377:errorcluster, "Value"=w1379:bool)  [unwired: 1 in, 1 out]
          n560 = case shown="False" w1379 {
            tunnel: w1380 -> [w1399 _]
            tunnel: w1377 -> [w1397 w1400]
            tunnel: [w1397 w1400] -> w1376
            frame False {
              n561 = Not(x=w1399) -> (.not. x?=w1398:bool)
              n562 = property on="Test Failed" class="Bool (strict)"("Value"=w1398) -> ()  [unwired: 2 in, 2 out]
            }
            frame True {
            }
          }
          n563 = property on="Automation" class="Bool (strict)"(error in=w1376) -> ("Value"=w1381:bool)  [unwired: 1 in, 2 out]
          n564 = case shown="True" w1381 {
            frame False {
            }
            frame True {
              w1401 = TRUE ("Value (Signaling)")
              n565 = property on="SetSN" class="Bool (strict)"("Val(Sgnl)"=w1401, "Value"=w1401) -> ()  [unwired: 2 in, 2 out]
            }
          }
        }
        frame "Temp Sens Cal" {
          w1405 = "2. Temperature sensor calibration test in process..." ("Value")
          w1403 = "2" ("Test Paragraph")
          n566 = control-ref of="Pannel User Message"() -> (w1412:refnum<vi>)
          n567 = property class="Str"(reference=w1412, error in=w1411, "Value"=w1405) -> (error out=w1410:errorcluster)  [unwired: 1 out]
          n568 = call "Table_ScrollaBarMarvin.vi"("error in"=w1410, "Line to focus"=w1403, "reference in"=w1413) -> ("error out"=w1415:errorcluster)  [unwired: 2 out]
          n569 = property class="Tbl (strict)"(reference=w1413, error in=w1415) -> (reference out=w1402:refnum<vi>, error out=w1417:errorcluster, "Value"=w1418:string[][])
          n570 = Index Array(array=w1418, index (col)=0 ("disabled index (col)")) -> (element=w1419:string[])  [unwired: 1 in]
          n571 = call "Find_Number_Line.vi"("error in"=w1417, "Test Paragraph"=w1403, "Row Headers[]"=w1419) -> ("error out"=w1414:errorcluster, "Line number"=w1407:i32)  [unwired: 1 out]
          n572 = property on="Status" class="Bool (strict)"(error in=w1414) -> (error out=w1408:errorcluster, "Value"=w1409:bool)  [unwired: 1 in, 1 out]
          n573 = call "Reset old test Values (SubVI).vi"("error in"=w1408, "Atr in"=w1402, "Test Paragraph"=w1403) -> ("error out"=w1404:errorcluster)  [unwired: 8 in]
          n574 = case shown="True" w1409 {
            selector: w1409 -> [w1423 _]
            tunnel: w1404 -> [w1425 _]
            tunnel: w1402 -> [w1422 _]
            tunnel: w1407 -> [w1421 _]
            tunnel: w1406 -> [_ w1432]
            tunnel: w1405 -> [_ w1428]
            frame False {
              n575 = flat-sequence {
                tunnel: w1425 -> [w1426]
                tunnel: [w1426] -> w1424
                frame #0 {
                  n576 = One Button Dialog(message="Please establish RS connection.") -> ()  [unwired: 1 in, 1 out]
                }
              }
              n577 = Increment(x=w1421) -> (x+1=w1420:i32)
              n578 = call "PassOrFail (SubVI).vi"("index (row)"=w1420, "error in (no error)"=w1424, "Pass?Fail"=w1423, "Table in"=w1422) -> ()  [unwired: 7 in, 1 out]
            }
            frame True {
              n579 = control-ref of="Stop Burn-in"() -> (w1434:refnum<vi>)
              n580 = control-ref of="Pannel User Message"() -> (w1436:refnum<vi>)
              n581 = control-ref of="Config_CANAT"() -> (w1430:refnum<vi>)
              n582 = control-ref of="ATR"() -> (w1437:refnum<vi>)
              n583 = control-ref of="Motor Speed RPM"() -> (w1438:refnum<vi>)
              n584 = control-ref of="UUT"() -> (w1429:refnum<vi>)
              n585 = control-ref of="Stop Button"() -> (w1435:refnum<vi>)
              n586 = property on="VISA Tester" class="VISAName"() -> ("Value"=w1431:refnum<visa-resource-name>)  [unwired: 2 in, 2 out]
              n587 = while {
                shift-right: [w1441] -> _
                shift-left: T14."Start" -> [w1451]
                tunnel: w1434 -> [w1450]
                tunnel: w1435 -> [w1449]
                tunnel: w1436 -> [w1448]
                tunnel: w1437 -> [w1447]
                tunnel: w1438 -> [w1446]
                tunnel: w1432 -> [w1445]
                tunnel: w1431 -> [w1444]
                tunnel: w1430 -> [w1443]
                tunnel: w1429 -> [w1442]
                tunnel: w1428 -> [w1439]
                stop <- w1440 stop-if-true
                n588 = case shown="\"AO[1]=Meas.\"" w1451 {
                  tunnel: w1450 -> [_ w1487 w1516 w1571 w1601]
                  tunnel: w1449 -> [_ w1488 w1508 w1557 w1603]
                  tunnel: w1448 -> [_ w1485 w1517 w1569 w1605]
                  tunnel: w1447 -> [_ w1465 _ _ _]
                  tunnel: w1446 -> [_ w1489 w1515 w1572 w1600]
                  tunnel: w1445 -> [_ w1498 w1520 w1581 w1597]
                  tunnel: w1444 -> [w1454 w1494 w1519 w1577 w1585]
                  tunnel: w1443 -> [_ _ _ _ w1611]
                  tunnel: w1442 -> [_ _ _ _ w1610]
                  tunnel: [w1452 w1474 w1509 w1560 w1588] -> w1441
                  tunnel: [w1453 FALSE FALSE FALSE FALSE] -> w1440
                  tunnel: w1439 -> [_ _ w1518 _ _]
                  frame "Stop", Default {
                    n589 = flat-sequence {
                      tunnel: w1454 -> [w1455]
                      tunnel: [TRUE] -> w1453
                      tunnel: [T14."Stop"] -> w1452
                      frame #0 {
                        n590 = call "TesterOption (SubVI).vi"("2 Options"=FALSE, "On/Off"=FALSE, "Tester Option"=T11."Power", "VISA Refnum in"=w1455) -> ()  [unwired: 6 in, 2 out]
                      }
                      frame #1 {
                      }
                    }
                  }
                  frame "AO[1]=Meas." {
                    n591 = property on="AO[1]Meas" class="DigNum (strict)"() -> ("Value"=w1468:dbl)  [unwired: 2 in, 2 out]
                    n592 = Number To Fractional String(number=w1468) -> (F-format string=w1476:string)  [unwired: 3 in]
                    n593 = Search and Replace String(input string="EP=1\r\nAO[1]=0\r\n" ("write buffer"), search string="0", replace string=w1476) -> (result string=w1475:string)  [unwired: 5 in, 3 out]
                    n594 = call "SerialMarvinSendGet.vi"("Clear Log"=FALSE, "write buffer"=w1475, "VISA resource name"=w1498) -> ("error out"=w1493:errorcluster)  [unwired: 7 in, 1 out]
                    n595 = call "TesterOption (SubVI).vi"("2 Options"=FALSE, "error in (no error)"=w1493, "On/Off"=FALSE, "Tester Option"=T11."Power", "VISA Refnum in"=w1494) -> ("error out"=w1492:errorcluster, "VISA Refnum out"=w1479:refnum<visa-resource-name>)  [unwired: 5 in]
                    n596 = call "Write panel message (SubVI).vi"("Stop BurnIn"=w1487, 4:"rpm"=w1489, 5:"rpm"=FALSE ("rpm"), "PrintTime"=TRUE, "Stop"=w1488, "error in (no error)"=w1492, "Time to wait"=20.0, "Strin"="2. Temperature sensor calibration test in process...\nSet Parameters...", "String in"=w1485) -> ("error out"=w1480:errorcluster)  [unwired: 2 in]
                    n597 = call "TesterOption (SubVI).vi"("2 Options"=FALSE, "error in (no error)"=w1480, "On/Off"=FALSE, "Tester Option"=T11."Venable", "VISA Refnum in"=w1479) -> ("error out"=w1473:errorcluster)  [unwired: 5 in, 1 out]
                    n598 = flat-sequence {
                      tunnel: [T14."Stop"] -> w1474
                      tunnel: w1466 -> [_]
                      frame #0 {
                      }
                    }
                    n599 = In Range and Coerce(upper limit=0.1, x=w1468, lower limit=-0.1) -> (In Range?=w1463:bool)  [unwired: 1 out]
                    "SensCalResult" <- w1463
                    n600 = property on="Test Failed" class="Bool (strict)"() -> ("Value"=w1462:bool)  [unwired: 2 in, 2 out]
                    n601 = call "Find_Number_LineMARVIN.vi"("Test Paragraph"="2.1", "error in"=w1473, "TableIn"=w1465) -> ("error out"=w1467:errorcluster, "Line number"=w1471:i32)  [unwired: 2 in, 2 out]
                    n602 = case shown="False" w1462 {
                      tunnel: w1463 -> [w1500 _]
                      frame False {
                        n603 = Not(x=w1500) -> (.not. x?=w1501:bool)
                        n604 = property on="Test Failed" class="Bool (strict)"("Value"=w1501) -> ()  [unwired: 2 in, 2 out]
                      }
                      frame True {
                      }
                    }
                    n605 = call "PassOrFail (SubVI).vi"("Test#"="2", "index (row)"=w1471, "error in (no error)"=w1467, "Data in"=w1468, "Pass?Fail"=w1463, "Table in"=w1465) -> ("error out"=w1466:errorcluster)  [unwired: 5 in]
                  }
                  frame "TA[5]" {
                    w1521 = T17 [enum."50C", enum."80C", enum."100C", enum."120C"] items=["K15", "K16", "K17", "Venable", "Firmeware", "Fan", "Power", "120C", "110C", "100C", "90C", "80C", "70C", "60C", "50C", "40C", "30C", "25C", "20C", "10C", "0C"]
                    n606 = for {
                      tunnel: w1521 -> [w1536] mode=indexing
                      tunnel: w1520 -> [w1535]
                      tunnel: w1519 -> [w1534]
                      tunnel: w1518 -> [w1533]
                      tunnel: w1517 -> [w1532]
                      tunnel: w1508 -> [w1531]
                      tunnel: w1516 -> [w1530]
                      tunnel: w1515 -> [w1529]
                      tunnel: dbl[] [0.59774, 0.65238, 0.68545, 0.71584] -> [w1524] mode=indexing
                      tunnel: [w1523] -> w1504 mode=indexing
                      tunnel: [w1522] -> w1507
                      n607 = for {
                        N: 5 -> [_]
                        tunnel: w1536 -> [w1554]
                        tunnel: w1535 -> [w1553]
                        tunnel: w1534 -> [w1549]
                        tunnel: w1533 -> [w1547]
                        tunnel: w1532 -> [w1546]
                        tunnel: w1531 -> [w1545]
                        tunnel: w1530 -> [w1543]
                        tunnel: w1529 -> [w1540]
                        tunnel: [w1539] -> w1528 mode=indexing
                        tunnel: [w1538] -> w1522
                        n608 = call "TesterOption (SubVI).vi"("2 Options"=FALSE, "On/Off"=TRUE, "Tester Option"=w1554, "VISA Refnum in"=w1549) -> ("error out"=w1550:errorcluster)  [unwired: 6 in, 1 out]
                        n609 = call "Write panel message (SubVI).vi"("Stop BurnIn"=w1543, 4:"rpm"=w1540, 5:"rpm"=FALSE ("rpm"), "PrintTime"=FALSE, "Stop"=w1545, "error in (no error)"=w1550, "Time to wait"=1.0, "Strin"=w1547, "String in"=w1546) -> ("error out"=w1548:errorcluster)  [unwired: 2 in]
                        n610 = call "SerialMarvinSendGet.vi"("error in (no error)"=w1548, "write buffer"="TA[5]\r\n", "VISA resource name"=w1553) -> ("error out"=w1538:errorcluster, "read buffer"=w1551:string)  [unwired: 7 in]
                        n611 = Fract/Exp String To Number(string=w1551) -> (number=w1539:dbl)  [unwired: 3 in, 1 out]
                      }
                      n612 = Add Array Elements(numeric array=w1528) -> (sum=w1527:dbl)
                      n613 = Divide(x=w1527, y=5.0) -> (x/y=w1525:dbl)
                      n614 = Subtract(x=w1525, y=w1524) -> (x-y=w1523:dbl)
                    }
                    n615 = property class="Bool (strict)"(reference=w1508, error in=w1507) -> ("Value"=w1513:bool)  [unwired: 2 out]
                    n616 = Select(t=T14."Stop", s=w1513, f=T14."AO[1]=Meas.") -> (s? t:f=w1509:T14)
                    n617 = Array Size(array=w1504) -> (size(s)=w1503:i32)
                    n618 = Add Array Elements(numeric array=w1504) -> (sum=w1506:dbl)
                    n619 = Divide(x=w1506, y=w1503) -> (x/y=→"AO[1]Meas":dbl)
                  }
                  frame "AO[1]=0" {
                    n620 = call "SerialMarvinSendGet.vi"("write buffer"="EP=1\r\nAO[1]=0\r\n", "VISA resource name"=w1581) -> ("error out"=w1576:errorcluster)  [unwired: 8 in, 1 out]
                    n621 = call "TesterOption (SubVI).vi"("2 Options"=FALSE, "error in (no error)"=w1576, "On/Off"=FALSE, "Tester Option"=T11."Power", "VISA Refnum in"=w1577) -> ("error out"=w1575:errorcluster, "VISA Refnum out"=w1563:refnum<visa-resource-name>)  [unwired: 5 in]
                    n622 = call "Write panel message (SubVI).vi"("Stop BurnIn"=w1571, 4:"rpm"=w1572, 5:"rpm"=FALSE ("rpm"), "PrintTime"=TRUE, "Stop"=w1557, "error in (no error)"=w1575, "Time to wait"=20.0, "Strin"="2. Temperature sensor calibration test in process...\nSet Parameters...", "String in"=w1569) -> ("error out"=w1564:errorcluster)  [unwired: 2 in]
                    n623 = call "TesterOption (SubVI).vi"("2 Options"=FALSE, "error in (no error)"=w1564, "On/Off"=FALSE, "Tester Option"=T11."Venable", "VISA Refnum in"=w1563) -> ("error out"=w1558:errorcluster)  [unwired: 5 in, 1 out]
                    n624 = property class="Bool (strict)"(reference=w1557, error in=w1558) -> ("Value"=w1562:bool)  [unwired: 2 out]
                    n625 = Select(t=T14."Stop", s=w1562, f=T14."TA[5]") -> (s? t:f=w1560:T14)
                  }
                  frame "Start" {
                    n626 = call "Write panel message (SubVI).vi"("Stop BurnIn"=w1601, 4:"rpm"=w1600, 5:"rpm"=FALSE ("rpm"), "PrintTime"=FALSE, "Stop"=w1603, "Time to wait"=0.1, "Strin"="2. Temperature sensor calibration test in process...\nInitialization state...", "String in"=w1605) -> ("error out"=w1606:errorcluster)  [unwired: 3 in]
                    n627 = call "TesterOption (SubVI).vi"("2 Options"=FALSE, "error in (no error)"=w1606, "On/Off"=FALSE, "Tester Option"=T11."Venable", "VISA Refnum in"=w1585) -> ("error out"=w1608:errorcluster)  [unwired: 5 in, 1 out]
                    n628 = call "CANSendMotorSpeed.vi"("Remote"=TRUE, "error in (no error)"=w1608, "Motor Speed RPM"=u16 0, "UUT"=w1610, "CAN Cluster in"=w1611) -> ("error out"=w1595:errorcluster)  [unwired: 6 in]
                    n629 = call "SerialMarvinSendGet.vi"("error in (no error)"=w1595, "write buffer"="AO[1]\r\n", "VISA resource name"=w1597) -> ("error out"=w1584:errorcluster, "read buffer"=w1594:string)  [unwired: 7 in]
                    n630 = Equal?(x=w1594, y="0.0") -> (x = y?=w1586:bool)
                    n631 = property class="Bool (strict)"(reference=w1603, error in=w1584) -> ("Value"=w1615:bool)  [unwired: 2 out]
                    n632 = Select(t=T14."TA[5]", s=w1586, f=T14."AO[1]=0") -> (s? t:f=w1590:T14)
                    n633 = Select(t=T14."Stop", s=w1615, f=w1590) -> (s? t:f=w1588:T14)
                  }
                }
              }
            }
          }
        }
        frame "Auxiliary" {
          w1619 = "9. Auxiliary test in process..." ("Value")
          w1631 = "9" ("Test Paragraph")
          n634 = control-ref of="Pannel User Message"() -> (w1630:refnum<vi>)
          n635 = property class="Str"(reference=w1630, error in=w1627, "Value"=w1619) -> (error out=w1629:errorcluster)  [unwired: 1 out]
          n636 = call "Table_ScrollaBarMarvin.vi"("error in"=w1629, "Line to focus"=w1631, "reference in"=w1628) -> ("error out"=w1637:errorcluster)  [unwired: 2 out]
          n637 = property class="Tbl (strict)"(reference=w1628, error in=w1637) -> (reference out=w1626:refnum<vi>, error out=w1636:errorcluster, "Value"=w1635:string[][])
          n638 = Index Array(array=w1635, index (col)=0 ("disabled index (col)")) -> (element=w1634:string[])  [unwired: 1 in]
          n639 = call "Find_Number_Line.vi"("error in"=w1636, "Test Paragraph"=w1631, "Row Headers[]"=w1634) -> ("error out"=w1632:errorcluster, "Line number"=w1617:i32)  [unwired: 1 out]
          n640 = call "Reset old test Values (SubVI).vi"("error in"=w1632, "Atr in"=w1626, "Test Paragraph"=w1631) -> ("error out"=w1624:errorcluster)  [unwired: 8 in]
          n641 = property on="VISA Tester" class="VISAName"() -> ("Value"=w1618:refnum<visa-resource-name>)  [unwired: 2 in, 2 out]
          n642 = control-ref of="Stop Burn-in"() -> (w1621:refnum<vi>)
          n643 = control-ref of="Stop Button"() -> (w1622:refnum<vi>)
          n644 = control-ref of="Pannel User Message"() -> (w1623:refnum<vi>)
          n645 = control-ref of="ATR"() -> (w1616:refnum<vi>)
          n646 = control-ref of="Config_CANAT"() -> ()  [unwired: 1 out]
          n647 = control-ref of="Motor Speed RPM"() -> (w1620:refnum<vi>)
          n648 = while {
            shift-right: [w1642] -> _
            shift-left: enum16{"Stop", "CoolingON", "HotGunON", "Start"}."Start" -> [w1649]
            tunnel: w1624 -> [w1640]
            tunnel: w1623 -> [w1648]
            tunnel: w1622 -> [w1647]
            tunnel: w1621 -> [w1646]
            tunnel: w1620 -> [w1645]
            tunnel: w1619 -> [w1644]
            tunnel: w1618 -> [w1643]
            tunnel: w1617 -> [w1639]
            tunnel: w1616 -> [w1638]
            stop <- w1641 stop-if-true
            n649 = case shown="\"Stop\", Default" w1649 {
              tunnel: w1648 -> [_ w1696 w1778 w1840]
              tunnel: w1647 -> [_ w1688 w1770 w1826]
              tunnel: w1646 -> [_ w1695 w1777 w1839]
              tunnel: w1645 -> [_ w1694 w1776 w1835]
              tunnel: w1644 -> [_ w1681 w1763 w1834]
              tunnel: w1643 -> [_ w1682 w1764 w1827]
              tunnel: [w1651 w1684 w1766 w1822] -> w1642
              tunnel: [w1650 FALSE FALSE FALSE] -> w1641
              tunnel: w1640 -> [_ w1680 w1762 _]
              tunnel: w1639 -> [_ w1674 w1757 _]
              tunnel: w1638 -> [_ w1670 w1754 _]
              frame "Stop", Default {
                n650 = flat-sequence {
                  tunnel: [enum16{"Stop", "CoolingON", "HotGunON", "Start"}."Stop"] -> w1651
                  tunnel: [TRUE] -> w1650
                  frame #0 {
                    n651 = property on="VISA Tester" class="VISAName"() -> ("Value"=w1655:refnum<visa-resource-name>)  [unwired: 2 in, 2 out]
                    n652 = call "TesterOption (SubVI).vi"("2 Options"=FALSE, "On/Off"=FALSE, "Tester Option"=T11."Power", "VISA Refnum in"=w1655) -> ()  [unwired: 6 in, 2 out]
                  }
                  frame #1 {
                  }
                }
              }
              frame "CoolingON" {
                n653 = while {
                  tunnel: w1696 -> [w1731]
                  tunnel: w1695 -> [w1730]
                  tunnel: w1694 -> [w1726]
                  tunnel: [w1722] -> w1677
                  tunnel: w1688 -> [w1713]
                  tunnel: w1682 -> [w1723]
                  tunnel: w1681 -> [w1717]
                  tunnel: w1680 -> [w1714]
                  shift-right: [w1706] -> _
                  shift-left: 0.0 -> [w1707]
                  shift-right: [w1700] -> w1665
                  shift-left: 0.0 ("Value") -> [w1704]
                  tunnel: [w1701] -> w1661
                  stop <- w1711 stop-if-true
                  n654 = control-ref of="Power transistor Heat sink Temp."() -> (w1724:refnum<vi>)
                  n655 = property class="DigNum (strict)"(reference=w1724, error in=w1714) -> (error out=w1720:errorcluster, "Value"=w1700:dbl)  [unwired: 1 out]
                  n656 = Equal?(x=w1700, y=w1704) -> (x = y?=w1703:bool)
                  n657 = Number To Fractional String(number=w1700, precision (6)=i16 2) -> (F-format string=w1716:string)  [unwired: 2 in]
                  n658 = case shown="True" w1703 {
                    tunnel: w1707 -> [_ w1737]
                    tunnel: [0.0 w1735] -> w1706
                    tunnel: [FALSE w1734] -> w1705
                    frame False {
                    }
                    frame True {
                      n659 = Increment(x=w1737) -> (x+1=w1735:dbl)
                      n660 = Greater Or Equal?(x=w1735, y=300.0) -> (x >= y?=w1734:bool)
                    }
                  }
                  n661 = Concatenate Strings(w1717, "\nPCB Temperature [C]: " ("string"), w1716) -> (w1715:string)
                  n662 = call "Write panel message (SubVI).vi"("Stop BurnIn"=w1730, 4:"rpm"=w1726, 5:"rpm"=FALSE ("rpm"), "PrintTime"=FALSE, "Stop"=w1713, "error in (no error)"=w1720, "Time to wait"=0.2, "Strin"=w1715, "String in"=w1731) -> ("error out"=w1719:errorcluster)  [unwired: 2 in]
                  n663 = property class="Bool (strict)"(reference=w1713) -> ("Value"=w1712:bool)  [unwired: 1 in, 2 out]
                  n664 = Less Or Equal?(x=w1700, y=53.0) -> (x <= y?=w1702:bool)
                  n665 = call "GetADCTester (SubVI).vi"("error in (no error)"=w1719, "GetADCTester"=T13."Fan", "VISA Refnum in"=w1723) -> ("error out"=w1722:errorcluster, "ADCValOutput Single"=w1709:dbl)  [unwired: 6 in, 1 out]
                  n666 = Greater?(x=w1709, y=u32 2400) -> (0:w1701:bool)
                  n667 = Compound Arithmetic op=OR(w1701, w1712, w1702, w1705) -> (w1711:bool)
                }
                n668 = In Range and Coerce(upper limit=57.0, x=w1665, lower limit=53.0) -> (In Range?=w1660:bool)  [unwired: 1 out]
                n669 = Build Array(w1661, w1660) -> (w1662:bool[])
                n670 = And Array Elements(Boolean array=w1662) -> (logical AND=w1659:bool)
                "AuxiOFFResult" <- w1659
                n671 = Add(x=w1674, y=3) -> (x+y=w1672:i32)
                n672 = call "PassOrFail (SubVI).vi"("index (row)"=w1672, "error in (no error)"=w1677, "Data in"=w1665, "Pass?Fail"=w1660, "Table in"=w1670) -> ("error out"=w1676:errorcluster)  [unwired: 6 in]
                n673 = Select(t="OFF", s=w1661, f="ON") -> (s? t:f=w1666:string)
                n674 = Increment(x=w1672) -> (x+1=w1671:i32)
                n675 = property on="Test Failed" class="Bool (strict)"() -> ("Value"=w1658:bool)  [unwired: 2 in, 2 out]
                n676 = call "PassOrFail (SubVI).vi"("String Res"=w1666, "index (row)"=w1671, "error in (no error)"=w1676, "Data in"=-3.0, "Pass?Fail"=w1661, "Table in"=w1670) -> ("error out"=w1675:errorcluster)  [unwired: 5 in]
                n677 = case shown="False" w1658 {
                  tunnel: w1659 -> [w1698 _]
                  frame False {
                    n678 = Not(x=w1698) -> (.not. x?=w1699:bool)
                    n679 = property on="Test Failed" class="Bool (strict)"("Value"=w1699) -> ()  [unwired: 2 in, 2 out]
                  }
                  frame True {
                  }
                }
                n680 = call "TesterOption (SubVI).vi"("On/Off 2"=TRUE, "Tester Option 2"=T11."Power", "2 Options"=FALSE, "error in (no error)"=w1675, "On/Off"=FALSE, "Tester Option"=T11."Venable", "VISA Refnum in"=w1682) -> ("error out"=w1687:errorcluster)  [unwired: 3 in, 1 out]
                n681 = property class="Bool (strict)"(reference=w1688, error in=w1687) -> ("Value"=w1697:bool)  [unwired: 2 out]
                n682 = Select(t=enum16{"Stop", "CoolingON", "HotGunON", "Start"}."Stop", s=w1697, f=enum16{"Stop", "CoolingON", "HotGunON", "Start"}."Stop") -> (s? t:f=w1684:enum16{"Stop", "CoolingON", "HotGunON", "Start"})
              }
              frame "HotGunON" {
                n683 = while {
                  tunnel: w1778 -> [w1813]
                  tunnel: w1777 -> [w1812]
                  tunnel: w1776 -> [w1808]
                  tunnel: [w1804] -> w1746
                  tunnel: w1770 -> [w1795]
                  tunnel: w1764 -> [w1805]
                  tunnel: w1763 -> [w1799]
                  tunnel: w1762 -> [w1796]
                  shift-right: [w1788] -> _
                  shift-left: 0.0 -> [w1789]
                  shift-right: [w1785] -> _
                  shift-left: 0.0 ("Value") -> [w1786]
                  tunnel: [w1783] -> w1741
                  stop <- w1793 stop-if-true
                  n684 = control-ref of="Power transistor Heat sink Temp."() -> (w1806:refnum<vi>)
                  n685 = property class="DigNum (strict)"(reference=w1806, error in=w1796) -> (error out=w1802:errorcluster, "Value"=w1785:dbl)  [unwired: 1 out]
                  n686 = Equal?(x=w1785, y=w1786) -> (x = y?=w1784:bool)
                  n687 = Number To Fractional String(number=w1785, precision (6)=i16 2) -> (F-format string=w1798:string)  [unwired: 2 in]
                  n688 = case shown="True" w1784 {
                    tunnel: w1789 -> [_ w1819]
                    tunnel: [0.0 w1817] -> w1788
                    tunnel: [FALSE w1816] -> w1787
                    frame False {
                    }
                    frame True {
                      n689 = Increment(x=w1819) -> (x+1=w1817:dbl)
                      n690 = Greater Or Equal?(x=w1817, y=300.0) -> (x >= y?=w1816:bool)
                    }
                  }
                  n691 = Concatenate Strings(w1799, "\nPCB Temperature [C]: " ("string"), w1798) -> (w1797:string)
                  n692 = call "Write panel message (SubVI).vi"("Stop BurnIn"=w1812, 4:"rpm"=w1808, 5:"rpm"=FALSE ("rpm"), "PrintTime"=FALSE, "Stop"=w1795, "error in (no error)"=w1802, "Time to wait"=0.2, "Strin"=w1797, "String in"=w1813) -> ("error out"=w1801:errorcluster)  [unwired: 2 in]
                  n693 = property class="Bool (strict)"(reference=w1795) -> ("Value"=w1794:bool)  [unwired: 1 in, 2 out]
                  n694 = call "GetADCTester (SubVI).vi"("error in (no error)"=w1801, "GetADCTester"=T13."Fan", "VISA Refnum in"=w1805) -> ("error out"=w1804:errorcluster, "ADCValOutput Single"=w1791:dbl)  [unwired: 6 in, 1 out]
                  n695 = Greater Or Equal?(x=w1785, y=61.0) -> (x >= y?=w1782:bool)
                  n696 = Less?(x=w1791, y=u32 100) -> (x < y?=w1783:bool)
                  n697 = Compound Arithmetic op=OR(w1783, w1794, w1782, w1787) -> (w1793:bool)
                }
                n698 = control-ref of="Power transistor Heat sink Temp."() -> (w1747:refnum<vi>)
                n699 = call "Time Delay2"("error in (no error)"=w1746) -> ("error out"=w1743:errorcluster)  [unwired: 10 in]
                n700 = property class="DigNum (strict)"(reference=w1747, error in=w1743) -> (error out=w1745:errorcluster, "Value"=w1744:dbl)  [unwired: 1 out]
                n701 = In Range and Coerce(upper limit=62.0, x=w1744, lower limit=58.0) -> (In Range?=w1740:bool)  [unwired: 1 out]
                n702 = Build Array(w1741, w1740) -> (w1742:bool[])
                n703 = property on="Test Failed" class="Bool (strict)"() -> ("Value"=w1738:bool)  [unwired: 2 in, 2 out]
                n704 = Increment(x=w1757) -> (x+1=w1756:i32)
                n705 = call "PassOrFail (SubVI).vi"("index (row)"=w1756, "error in (no error)"=w1745, "Data in"=w1744, "Pass?Fail"=w1740, "Table in"=w1754) -> ("error out"=w1759:errorcluster)  [unwired: 6 in]
                n706 = And Array Elements(Boolean array=w1742) -> (logical AND=w1739:bool)
                "AuxiONResult" <- w1739
                n707 = Increment(x=w1756) -> (x+1=w1755:i32)
                n708 = Select(t="ON", s=w1741, f="OFF") -> (s? t:f=w1752:string)
                n709 = call "PassOrFail (SubVI).vi"("String Res"=w1752, "index (row)"=w1755, "error in (no error)"=w1759, "Data in"=-3.0, "Pass?Fail"=w1741, "Table in"=w1754) -> ("error out"=w1758:errorcluster)  [unwired: 5 in]
                n710 = case shown="False" w1738 {
                  tunnel: w1739 -> [w1780 _]
                  frame False {
                    n711 = Not(x=w1780) -> (.not. x?=w1781:bool)
                    n712 = property on="Test Failed" class="Bool (strict)"("Value"=w1781) -> ()  [unwired: 2 in, 2 out]
                  }
                  frame True {
                  }
                }
                n713 = call "TesterOption (SubVI).vi"("On/Off 2"=TRUE, "Tester Option 2"=T11."Fan", "2 Options"=FALSE, "error in (no error)"=w1758, "On/Off"=FALSE, "Tester Option"=T11."Venable", "VISA Refnum in"=w1764) -> ("error out"=w1769:errorcluster)  [unwired: 3 in, 1 out]
                n714 = property class="Bool (strict)"(reference=w1770, error in=w1769) -> ("Value"=w1779:bool)  [unwired: 2 out]
                n715 = Select(t=enum16{"Stop", "CoolingON", "HotGunON", "Start"}."Stop", s=w1779, f=enum16{"Stop", "CoolingON", "HotGunON", "Start"}."CoolingON") -> (s? t:f=w1766:enum16{"Stop", "CoolingON", "HotGunON", "Start"})
              }
              frame "Start" {
                n716 = call "Write panel message (SubVI).vi"("Stop BurnIn"=w1839, 4:"rpm"=w1835, 5:"rpm"=FALSE ("rpm"), "PrintTime"=FALSE, "Stop"=w1826, "Time to wait"=0.1, "Strin"=w1834, "String in"=w1840) -> ("error out"=w1833:errorcluster)  [unwired: 3 in]
                n717 = call "TesterOption (SubVI).vi"("On/Off 2"=TRUE, "Tester Option 2"=T11."Fan", "2 Options"=TRUE, "error in (no error)"=w1833, "On/Off"=FALSE, "Tester Option"=T11."Venable", "VISA Refnum in"=w1827) -> ("error out"=w1825:errorcluster)  [unwired: 3 in, 1 out]
                n718 = call "Time Delay"("error in (no error)"=w1825) -> ("error out"=w1820:errorcluster)  [unwired: 10 in]
                n719 = property class="Bool (strict)"(reference=w1826, error in=w1820) -> ("Value"=w1841:bool)  [unwired: 2 out]
                n720 = Select(t=enum16{"Stop", "CoolingON", "HotGunON", "Start"}."Stop", s=w1841, f=enum16{"Stop", "CoolingON", "HotGunON", "Start"}."HotGunON") -> (s? t:f=w1822:enum16{"Stop", "CoolingON", "HotGunON", "Start"})
              }
            }
          }
        }
      }
    }
    n721 = flat-sequence {
      tunnel: w186 -> [_]
      frame #0 {
        w194 = T18."Enabled" ("Disabled")
        w195 = FALSE ("Start")
        n722 = property on="Start" class="Bool (strict)"("Value"=w195, "DisabledEnum"=w194) -> ()  [unwired: 2 in, 2 out]
        n723 = property on="Report" class="Bool (strict)"("Value"=w195, "DisabledEnum"=w194) -> ()  [unwired: 2 in, 2 out]
      }
    }
  }
  n724 = while {
    shift-right: [w1860] -> _
    shift-left: T10."Initialize" -> [w1859]
    shift-right: [w1856] -> _
    shift-left: w17 -> [w1857]
    shift-right: [w1855] -> _
    shift-left: _ -> [w1854]
    shift-right: [w1853] -> _
    shift-left: w20 -> [w1851]
    shift-right: [w1852] -> _
    shift-left: refnum<vi> refnum ("Config_CANAT") -> [w1850]
    shift-right: [w1848] -> _
    shift-left: w16 -> [w1849]
    tunnel: "ATR" -> [_]
    tunnel: w7 -> [w1847]
    tunnel: w6 -> [w1846]
    shift-right: [w1844] -> _
    shift-left: 0 -> [w1845]
    tunnel: w4 -> [w1843]
    tunnel: w2 -> [w1842]
    tunnel: w1 -> [_]
    stop <- w1858 stop-if-true
    n725 = case shown="\"Initialize\"" w1859 {
      tunnel: [T10."MainProgram" w1953 w2003 T10."Erase ATR Table"] -> w1860
      tunnel: [FALSE TRUE FALSE FALSE] -> w1858
      tunnel: [w1864 w1947 w1997 w2801] -> w1856
      tunnel: w1857 -> [_ w1966 w2001 _]
      tunnel: [w1904 refnum<visa-resource-name> refnum ("VISA resource name") w1998 w2806] -> w1855
      tunnel: w1854 -> [w1904 w1976 w1999 _]
      tunnel: [w1891 refnum<queue> refnum ("queue out") w1993 w2799] -> w1853
      tunnel: [w1890 refnum<vi> refnum ("Config_CANAT") w1994 w2802] -> w1852
      tunnel: w1851 -> [w1891 w1978 w1996 w2799]
      tunnel: w1850 -> [w1890 w1957 w1995 _]
      tunnel: w1849 -> [w1889 w1970 w1992 w2798]
      tunnel: [w1889 refnum<queue> refnum ("queue out") w1991 w2798] -> w1848
      tunnel: w1847 -> [_ _ w1990 _]
      tunnel: w1846 -> [_ _ w1989 _]
      tunnel: w1845 -> [w1878 w1960 w1988 w2795]
      tunnel: [w1878 w1960 w1987 w2795] -> w1844
      tunnel: w1843 -> [w1868 _ w1986 _]
      tunnel: w1842 -> [_ _ w1985 _]
      frame "Erase ATR Table", Default {
        w1872 = "Marvin" ("section")
        w1885 = refnum<visa-resource-name> "COM4" ("VISA resource name")
        w1899 = FALSE ("Visible")
        n726 = property on="Serial Com" class="Bool"(error in=errorcluster {"status"=FALSE, "code"=0, "source"=""} ("error out"), "Visible"=TRUE) -> (error out=w1886:errorcluster)  [unwired: 1 in, 1 out]
        n727 = property on="VISA Marvin" class="VISAName"(error in=w1886, "Visible"=w1899, "Value"=w1885) -> (error out=w1901:errorcluster)  [unwired: 1 in, 1 out]
        n728 = property on="VISA Marvin" class="VISAName"(error in=w1886, "Value"=w1885) -> ()  [unwired: 1 in, 2 out]
        n729 = case shown="False" w1896 {
          tunnel: [string[][] [["1", "Communication Test", "", "", "", "", ""], ["1.1", "Serial RS-232", "N/A", "-", "", "", ""], ["1.2", "CAN Bus", "N/A", "-", "", "", ""], ["", "", "", "", "", "", ""], ["2", "Temperature Sensor Calibration Test", "", "", "", "", ""], ["2.1", "Sensor Reading Analog Offset", "0", "+/-0.100", ".", "", ""], ["", "", "", "", "", "", ""], ["3", "Motor Temp. Test", "", "", "", "", ""], ["3.1", "60 Degree", "60", "+/-3.00", "C", "", ""], ["3.2", "90 Degree", "90", "+/-3.00", "C", "", ""], ["3.3", "120 Degree", "120", "+/-3.00", "C", "", ""], ["", "", "", "", "", "", ""], ["4", "Enable Test", "", "", "", "", ""], ["4.1", "Fan Speed at Opened Enable ", "5000", "+/-200.0", "rpm", "", ""], ["4.2", "Fan Speed at Opened Enable ", "0", "+/-200.0", "rpm", "", ""], ["4.3", "Fan Speed at Closed Enable ", "5000", "+/-200.0", "rpm", "", ""], ["4.4", "Motor Rotation Direction", "Counter-clockwise (Inlet)", "-", "", "", ""], ["", "", "", "", "", "", ""], ["5", "Speed Command Test", "", "", "", "", ""], ["5.1", "Fan Speed", "6000", "+/-200.0", "rpm", "", ""], ["5.2", "Fan Speed", "11500", "+/-200.0", "rpm", "", ""], ["5.3", "Fan Speed", "12100", "+/-200.0", "rpm", "", ""], ["", "", "", "", "", "", ""], ["6", "Stop Time Test ", "", "", "", "", ""], ["6.1", "Motor Stop time", "< 50", "-", "sec", "", ""], ["", "", "", "", "", "", ""], ["7", "Burn-in Test", "", "", "", "", ""], ["7.1", "DC Input Current", "50", "+/-5.000", "A", "", ""], ["7.2", "Fan Speed", "15100", "+/-200.0", "rpm", "", ""], ["7.3", "Ambient Temperature", "25", "+/-13.00", "C", "", ""], ["7.4", "After 10 min of operation", "", "-", "C", "", ""], ["7.5", "After 20 min of operation", "", "-", "C", "", ""], ["7.6", "After 30 min of operation", "", "-", "C", "", ""], ["", "", "", "", "", "", ""], ["8", "Visual Inspection", "", "", "", "", ""], ["8.1", "Verification of Components Not Installed", "N/A", "-", "", "", ""], ["", "", "", "", "", "", ""], ["9", "Manufacturing Defects", "N/A", "-", "", "", ""], ["", "", "", "", "", "", ""], ["10", "Power Supply Testing", "", "", "", "", ""], ["10.1", "Input Current Drawn", "", "", "", "", ""], ["10.2", "DC Input Current", "< 150", "-", "mA", "", ""], ["", "", "", "", "", "", ""], ["11", "Power Supply Voltages", "", "", "", "", ""], ["11.1", "12V", "12.0", "+/-0.500", "V", "", ""], ["11.2", "5V", "5.0", "+/-0.200", "V", "", ""], ["11.3", "3.3V", "3.3", "+/-0.100", "V", "", ""], ["11.4", "1.8V", "1.8", "+/-0.100", "V", "", ""], ["", "", "", "", "", "", ""], ["12", "Functional Test Procedure", "", "", "", "", ""], ["12.1", "Weight Check", "4180", "+/-10.00", "gr", "", ""], ["", "", "", "", "", "", ""], ["13", "Insulation Resistance Test", "", "", "", "", ""], ["13.1", "J3.B to Chassis", "> 1M", "-", "ohms", "", ""], ["13.2", "J1.16 to Chassis", "> 100K", "-", "ohms", "", ""], ["", "", "", "", "", "", ""], ["14", "Bonding Resistance", "", "", "", "", ""], ["14.1", "J1 Body to Chassis", "< 2m", "-", "ohms", "", ""], ["14.2", "J2  Body to Chassis", "< 2m", "-", "ohms", "", ""], ["14.3", "J3  Body to Chassis", "< 2m", "-", "ohms", "", ""], ["", "", "", "", "", "", ""], ["15", "CANbus Resistance Test", "", "", "", "", ""], ["15.1", "J1.17 to J1.18", "> 10K", "-", "ohms", "", ""], ["", "", "", "", "", "", ""], ["16", "Sealing Test", "N/A", "-", "", "", ""], ["", "", "", "", "", "", ""], ["17", "Performances Tests", "", "", "", "", ""], ["17.1", "Reverse Polarity Test", "", "", "", "", ""], ["17.2", "DC Input Current", "< 1", "-", "mA", "", ""]] ("ArrAHU 2") string[][] [["1", "Communication Test", "", "", "", "", ""], ["1.1", "Serial RS-232", "N/A", "-", "", "", ""], ["1.2", "CAN Bus", "N/A", "-", "", "", ""], ["", "", "", "", "", "", ""], ["2", "Temperature Sensor Calibration Test", "", "", "", "", ""], ["2.1", "Sensor Reading Analog Offset", "0", "+/-0.100", ".", "", ""], ["", "", "", "", "", "", ""], ["3", "Motor Temp. Test", "", "", "", "", ""], ["3.1", "60 Degree", "60", "+/-3.00", "C", "", ""], ["3.2", "90 Degree", "90", "+/-3.00", "C", "", ""], ["3.3", "120 Degree", "120", "+/-3.00", "C", "", ""], ["", "", "", "", "", "", ""], ["4", "Enable Test", "", "", "", "", ""], ["4.1", "Fan Speed at Opened Enable ", "5000", "+/-200.0", "rpm", "", ""], ["4.2", "Fan Speed at Opened Enable ", "0", "+/-200.0", "rpm", "", ""], ["4.3", "Fan Speed at Closed Enable ", "5000", "+/-200.0", "rpm", "", ""], ["4.4", "Motor Rotation Direction", "Counter-clockwise (Inlet)", "-", "", "", ""], ["", "", "", "", "", "", ""], ["5", "Speed Command Test", "", "", "", "", ""], ["5.1", "Fan Speed", "6000", "+/-200.0", "rpm", "", ""], ["5.2", "Fan Speed", "11500", "+/-200.0", "rpm", "", ""], ["5.3", "Fan Speed", "15100", "+/-200.0", "rpm", "", ""], ["", "", "", "", "", "", ""], ["6", "Stop Time Test ", "", "", "", "", ""], ["6.1", "Motor Stop time", "< 50", "-", "sec", "", ""], ["", "", "", "", "", "", ""], ["7", "Temperature Control Algorithm Test", "", "", "", "", ""], ["7.1", "Tair <   68 ± 2 oC", "6000", "+/-200.0", "rpm", "", ""], ["7.2", "Measured Temp.", "", "", "C", "", ""], ["7.3", "Tair >= 68 ± 2 oC", "11500", "+/-200.0", "rpm", "", ""], ["7.4", "Transition Temp.", "", "", "C", "", ""], ["7.5", "Tair >= 88 ± 2 oC", "15100", "+/-400.0", "rpm", "", ""], ["7.6", "Transition Temp.", "", "", "C", "", ""], ["7.7", "Tair <= 80 ± 2 oC", "11500", "+/-200.0", "rpm", "", ""], ["7.8", "Transition Temp.", "", "", "C", "", ""], ["7.9", "Tair <= 60 ± 2 oC", "6000", "+/-200.0", "rpm", "", ""], ["7.10", "Transition Temp.", "", "", "C", "", ""], ["", "", "", "", "", "", ""], ["8", "Burn-in Test", "", "", "", "", ""], ["8.1", "DC Input Current", "50", "+/-5.000", "A", "", ""], ["8.2", "Fan Speed", "15100", "+/-200.0", "rpm", "", ""], ["8.3", "Ambient Temperature", "25", "+/-13.00", "C", "", ""], ["8.4", "After 10 min of operation", "", "-", "C", "", ""], ["8.5", "After 20 min of operation", "", "-", "C", "", ""], ["8.6", "After 30 min of operation", "", "-", "C", "", ""], ["", "", "", "", "", "", ""], ["9", "Auxiliary", "", "", "", "", ""], ["9.1", "Auxiliary Cooling Fan ON", "60", "+/-2.00", "C", "", ""], ["9.2", "Fan status", "ON", "-", "-", "", ""], ["9.3", "Auxiliary Cooling Fan OFF", "55", "+/-2.00", "C", "", ""], ["9.4", "Fan status", "OFF", "-", "-", "", ""], ["", "", "", "", "", "", ""], ["10", "Visual Inspection", "", "", "", "", ""], ["10.1", "Verification of Components Not Installed", "N/A", "-", "", "", ""], ["", "", "", "", "", "", ""], ["11", "Manufacturing Defects", "N/A", "-", "", "", ""], ["", "", "", "", "", "", ""], ["12", "Power Supply Testing", "", "", "", "", ""], ["12.1", "Input Current Drawn", "", "", "", "", ""], ["12.2", "DC Input Current", "< 150", "-", "mA", "", ""], ["", "", "", "", "", "", ""], ["13", "Power Supply Voltages", "", "", "", "", ""], ["13.1", "12V", "12.0", "+/-0.500", "V", "", ""], ["13.2", "5V", "5.0", "+/-0.200", "V", "", ""], ["13.3", "3.3V", "3.3", "+/-0.100", "V", "", ""], ["13.4", "1.8V", "1.8", "+/-0.100", "V", "", ""], ["", "", "", "", "", "", ""], ["14", "Functional Test Procedure", "", "", "", "", ""], ["14.1", "Weight Check", "4180", "+/-10.00", "gr", "", ""], ["", "", "", "", "", "", ""], ["15", "Insulation Resistance Test", "", "", "", "", ""], ["15.1", "J3.B to Chassis", "> 1M", "-", "ohms", "", ""], ["15.2", "J1.16 to Chassis", "> 100K", "-", "ohms", "", ""], ["", "", "", "", "", "", ""], ["16", "Bonding Resistance", "", "", "", "", ""], ["16.1", "J1 Body to Chassis", "< 2m", "-", "ohms", "", ""], ["16.2", "J2  Body to Chassis", "< 2m", "-", "ohms", "", ""], ["16.3", "J3  Body to Chassis", "< 2m", "-", "ohms", "", ""], ["", "", "", "", "", "", ""], ["17", "CANbus Resistance Test", "", "", "", "", ""], ["17.1", "J1.17 to J1.18", "> 10K", "-", "ohms", "", ""], ["", "", "", "", "", "", ""], ["18", "Sealing Test", "N/A", "-", "", "", ""], ["", "", "", "", "", "", ""], ["19", "Performances Tests", "", "", "", "", ""], ["19.1", "Reverse Polarity Test", "", "", "", "", ""], ["19.2", "DC Input Current", "< 1", "-", "mA", "", ""]] ("ArrEbay 2")] -> w1897
          tunnel: ["AHU" "EBAY"] -> w1895
          tunnel: [w1919 w1931] -> w1892
          tunnel: w1893 -> [w1920 w1931]
          tunnel: [w1915 u8 95] -> w1865
          frame False {
            (unwired) string[][] [["6.1", "Visual Inspection", "", "", "", "", ""], ["6.1.1", "Verification of Components Not Installed", "N/A", "-", "", "", ""], ["", "", "", "", "", "", ""], ["6.1.2", "Manufacturing Defects", "N/A", "-", "", "", ""], ["", "", "", "", "", "", ""], ["6.2", "Power Supply Testing", "", "", "", "", ""], ["6.2.1", "Input Current Drawn", "", "", "", "", ""], ["6.2.1.1", "DC Input Current", "< 150", "-", "mA", "", ""], ["", "", "", "", "", "", ""], ["6.2.2", "Power Supply Voltages", "", "", "", "", ""], ["6.2.2.1", "12V", "12.0", "+/-0.500", "V", "", ""], ["6.2.2.2", "5V", "5.0", "+/-0.200", "V", "", ""], ["6.2.2.3", "3.3V", "3.3", "+/-0.100", "V", "", ""], ["6.2.2.4", "1.8V", "1.8", "+/-0.100", "V", "", ""], ["", "", "", "", "", "", ""], ["7", "Functional Test Procedure", "", "", "", "", ""], ["7.1", "Weight Check", "3800", "+/-100.0", "gr", "", ""], ["", "", "", "", "", "", ""], ["7.2", "Insulation Resistance Test", "", "", "", "", ""], ["7.2.1", "J3.B to Chassis", "> 1M", "-", "W", "", ""], ["7.2.2", "J1.16 to Chassis", "> 100K", "-", "W", "", ""], ["", "", "", "", "", "", ""], ["7.2", "Bonding Resistance", "", "", "", "", ""], ["7.2.3", "J1 Body to Chassis", "< 2m", "-", "W", "", ""], ["7.2.4", "J2  Body to Chassis", "< 2m", "-", "W", "", ""], ["7.2.5", "J3  Body to Chassis", "< 2m", "-", "W", "", ""], ["", "", "", "", "", "", ""], ["7.2.1", "CANbus Resistance Test", "", "", "", "", ""], ["7.2.1.1", "J1.17 to J1.18", "> 10K", "-", "W", "", ""], ["", "", "", "", "", "", ""], ["7.3", "Sealing Test", "N/A", "-", "", "", ""], ["", "", "", "", "", "", ""], ["7.4", "Communication Test", "", "", "", "", ""], ["7.4.1", "Serial RS-232", "N/A", "-", "", "", ""], ["7.4.2", "CAN Bus", "N/A", "-", "", "", ""], ["", "", "", "", "", "", ""], ["7.5", "Performances Tests", "", "", "", "", ""], ["7.5.1", "Reverse Polarity Test", "", "", "", "", ""], ["7.5.1.1", "DC Input Current", "< 1", "-", "mA", "", ""], ["", "", "", "", "", "", ""], ["7.5.2", "Enable Test", "", "", "", "", ""], ["7.5.2.1", "Fan Speed at Opened Enable ", "5000", "+/-200.0", "rpm", "", ""], ["7.5.2.2", "Fan Speed at Opened Enable ", "0", "+/-200.0", "rpm", "", ""], ["7.5.2.3", "Fan Speed at Closed Enable ", "5000", "+/-200.0", "rpm", "", ""], ["7.5.2.4", "Motor Rotation Direction", "Counter-clockwise (Inlet)", "-", "", "", ""], ["", "", "", "", "", "", ""], ["7.5.3", "Stop Time Test ", "", "", "", "", ""], ["7.5.3.1", "Motor Stop time", "< 50", "-", "sec", "", ""], ["", "", "", "", "", "", ""], ["7.5.4", "Speed Command Test", "", "", "", "", ""], ["7.5.4.1", "Fan Speed", "6000", "+/-200.0", "rpm", "", ""], ["7.5.4.2", "Fan Speed", "9000", "+/-200.0", "rpm", "", ""], ["7.5.4.3", "Fan Speed", "12100", "+/-200.0", "rpm", "", ""], ["", "", "", "", "", "", ""], ["7.5.5", "Temperature Sensor Calibration Test", "", "", "", "", ""], ["7.5.5.1", "Sensor Reading Analog Offset", "0", "+/-0.100", ".", "", ""], ["", "", "", "", "", "", ""], ["7.5.6", "Burn-in Test", "", "", "", "", ""], ["7.5.6.1", "DC Input Current", "28", "+/-3.000", "A", "", ""], ["7.5.6.2", "Fan Speed", "12100", "+/-200.000", "rpm", "", ""], ["7.5.6.3", "Ambient Temperature", "25", "+/-13.00", "C", "", ""], ["7.5.6.4", "After 10 min of operation", "", "", "C", "", ""], ["7.5.6.5", "After 20 min of operation", "", "", "C", "", ""], ["7.5.6.6", "After 30 min of operation", "", "", "C", "", ""], ["", "", "", "", "", "", ""], ["9", "Motor Temp Test", "", "", "", "", ""], ["9.1", "60 C", "60", "+/-3.000", "C", "", ""], ["9.2", "90 C", "90", "+/-3.000", "C", "", ""], ["9.3", "120 C", "120", "+/-3.000", "C", "", ""]] ("data")
            n730 = while {
              shift-right: [w1927] -> w1919
              shift-left: w1920 -> [w1928]
              tunnel: [w1922] -> w1918
              stop <- w1926 stop-if-true
              n731 = call "AHU UUT (subVI).vi"("error in (no error)"=w1928) -> ("AHU 47"=w1923:bool, "AHU 63"=w1922:bool, "OK"=w1925:bool, "error out"=w1927:errorcluster)  [unwired: 15 in]
              n732 = Exclusive Or(1:w1923, 2:w1922) -> (0:w1924:bool)
              n733 = And(x=w1925, y=w1924) -> (x .and. y?=w1926:bool)
            }
            n734 = Select(t=u8 63, s=w1918, f=u8 47) -> (s? t:f=w1915:u8)
          }
          frame True {
            (unwired) string[][] [["6.1", "Visual Inspection", "", "", "", "", ""], ["6.1.1", "Verification of Components Not Installed", "N/A", "-", "", "", ""], ["", "", "", "", "", "", ""], ["6.1.2", "Manufacturing Defects", "N/A", "-", "", "", ""], ["", "", "", "", "", "", ""], ["6.2", "Power Supply Testing", "", "", "", "", ""], ["6.2.1", "Input Current Drawn", "", "", "", "", ""], ["6.2.1.1", "DC Input Current", "< 150", "-", "mA", "", ""], ["", "", "", "", "", "", ""], ["6.2.2", "Power Supply Voltages", "", "", "", "", ""], ["6.2.2.1", "12V", "12.0", "+/-0.500", "V", "", ""], ["6.2.2.2", "5V", "5.0", "+/-0.200", "V", "", ""], ["6.2.2.3", "3.3V", "3.3", "+/-0.100", "V", "", ""], ["6.2.2.4", "1.8V", "1.8", "+/-0.100", "V", "", ""], ["", "", "", "", "", "", ""], ["7", "Functional Test Procedure", "", "", "", "", ""], ["7.1", "Weight Check", "4180", "+/-10.00", "gr", "", ""], ["", "", "", "", "", "", ""], ["7.2", "Insulation Resistance Test", "", "", "", "", ""], ["7.2.1", "J3.B to Chassis", "> 1M", "-", "W", "", ""], ["7.2.2", "J1.16 to Chassis", "> 100K", "-", "W", "", ""], ["", "", "", "", "", "", ""], ["7.2", "Bonding Resistance", "", "", "", "", ""], ["7.2.3", "J1 Body to Chassis", "< 2m", "-", "W", "", ""], ["7.2.4", "J2  Body to Chassis", "< 2m", "-", "W", "", ""], ["7.2.5", "J3  Body to Chassis", "< 2m", "-", "W", "", ""], ["", "", "", "", "", "", ""], ["7.2.1", "CANbus Resistance Test", "", "", "", "", ""], ["7.2.1.1", "J1.17 to J1.18", "> 10K", "-", "W", "", ""], ["", "", "", "", "", "", ""], ["7.3", "Sealing Test", "N/A", "-", "", "", ""], ["", "", "", "", "", "", ""], ["7.4", "Communication Test", "", "", "", "", ""], ["7.4.1", "Serial RS-232", "N/A", "-", "", "", ""], ["7.4.2", "CAN Bus", "N/A", "-", "", "", ""], ["", "", "", "", "", "", ""], ["7.5", "Performances Tests", "", "", "", "", ""], ["7.5.1", "Reverse Polarity Test", "", "", "", "", ""], ["7.5.1.1", "DC Input Current", "< 1", "-", "mA", "", ""], ["", "", "", "", "", "", ""], ["7.5.2", "Enable Test", "", "", "", "", ""], ["7.5.2.1", "Fan Speed at Opened Enable ", "5000", "+/-200.0", "rpm", "", ""], ["7.5.2.2", "Fan Speed at Opened Enable ", "0", "+/-200.0", "rpm", "", ""], ["7.5.2.3", "Fan Speed at Closed Enable ", "5000", "+/-200.0", "rpm", "", ""], ["7.5.2.4", "Motor Rotation Direction", "Counter-clockwise (Inlet)", "-", "", "", ""], ["", "", "", "", "", "", ""], ["7.5.3", "Stop Time Test ", "", "", "", "", ""], ["7.5.3.1", "Motor Stop time", "< 50", "-", "sec", "", ""], ["", "", "", "", "", "", ""], ["7.5.4", "Speed Command Test", "", "", "", "", ""], ["7.5.4.1", "Fan Speed", "6000", "+/-200.0", "rpm", "", ""], ["7.5.4.2", "Fan Speed", "11500", "+/-200.0", "rpm", "", ""], ["7.5.4.3", "Fan Speed", "15100", "+/-200.0", "rpm", "", ""], ["", "", "", "", "", "", ""], ["7.5.5", "Temperature Sensor Calibration Test", "", "", "", "", ""], ["7.5.5.1", "Sensor Reading Analog Offset", "0", "+/-0.100", ".", "", ""], ["", "", "", "", "", "", ""], ["7.5.6", "Temperature Control Algorithm Test", "", "", "", "", ""], ["7.5.6.1", "Tair <   68 ± 2 oC", "6000", "+/-200.0", "rpm", "", ""], ["7.5.6.2", "Measured Temp.", "", "", "C", "", ""], ["7.5.6.3", "Tair >= 68 ± 2 oC", "11500", "+/-200.0", "rpm", "", ""], ["7.5.6.4", "Transition Temp.", "", "", "C", "", ""], ["7.5.6.5", "Tair >= 88 ± 2 oC", "15100", "+/-400.0", "rpm", "", ""], ["7.5.6.6", "Transition Temp.", "", "", "C", "", ""], ["7.5.6.7", "Tair <= 80 ± 2 oC", "11500", "+/-200.0", "rpm", "", ""], ["7.5.6.8", "Transition Temp.", "", "", "C", "", ""], ["7.5.6.9", "Tair <= 60 ± 2 oC", "6000", "+/-200.0", "rpm", "", ""], ["7.5.6.10", "Transition Temp.", "", "", "C", "", ""], ["", "", "", "", "", "", ""], ["7.5.7", "Burn-in Test", "", "", "", "", ""], ["7.5.7.1", "DC Input Current", "50", "+/-5.000", "A", "", ""], ["7.5.7.2", "Fan Speed", "15100", "+/-200.0", "rpm", "", ""], ["7.5.7.3", "Ambient Temperature", "25", "+/-13.00", "C", "", ""], ["7.5.7.4", "After 10 min of operation", "", "-", "C", "", ""], ["7.5.7.5", "After 20 min of operation", "", "-", "C", "", ""], ["7.5.7.6", "After 30 min of operation", "", "-", "C", "", ""], ["", "", "", "", "", "", ""], ["8", "Auxiliary", "", "", "", "", ""], ["8.1", "Auxiliary Cooling Fan ON", "60", "+/-2.00", "C", "", ""], ["8.2", "Fan status", "ON", "-", "-", "", ""], ["8.3", "Auxiliary Cooling Fan OFF", "55", "+/-2.00", "C", "", ""], ["8.4", "Fan status", "OFF", "-", "-", "", ""], ["", "", "", "", "", "", ""], ["9", "Motor Temp. Test", "", "", "", "", ""], ["9.1", "60 Degree", "60", "+/-3.00", "C", "", ""], ["9.2", "90 Degree", "90", "+/-3.00", "C", "", ""], ["9.3", "120 Degree", "120", "+/-3.00", "C", "", ""]] ("data")
          }
        }
        "UUT" <- w1895
        "UUT" <- w1865
        n735 = property on="Status" class="Bool (strict)"(error in=w1901, "Value"=w1899) -> (error out=w1894:errorcluster)  [unwired: 1 in, 1 out]
        n736 = flat-sequence {
          tunnel: [w1911] -> w1896
          tunnel: w1894 -> [w1909]
          tunnel: [w1909] -> w1893
          frame #0 {
            n737 = Two Button Dialog(message="Please seect the Unit Under Test.", 1:"AHU" ("F button name (\"Cancel\")"), 2:"EBAY" ("T button name (\"OK\")")) -> (T button?=w1911:bool)
          }
        }
        n738 = for {
          tunnel: w1897 -> [w1937] mode=indexing
          tunnel: w1892 -> [w1935]
          tunnel: [w1934] -> w1888
          tunnel: w1897 -> [w1933]
          i -> [w1936]
          n739 = for {
            tunnel: w1937 -> [_] mode=indexing
            tunnel: w1936 -> [w1943]
            tunnel: w1935 -> [w1940]
            tunnel: [w1939] -> w1934
            tunnel: w1933 -> [w1938]
            i -> [w1944]
            n740 = Bundle By Name(cluster=T19 {"Row"=0, "Column"=0} ("Active Cell:Active Cell"), "Row"=w1943, "Column"=w1944) -> (w1942:T19)
            n741 = control-ref of="ATR"() -> (w1941:refnum<vi>)
            n742 = property class="Tbl (strict)"(reference=w1941, error in=w1940, "Active Cell"=w1942, "Cell BG Color"=u32 16777226, "Value"=w1938) -> (error out=w1939:errorcluster)  [unwired: 1 out]
          }
        }
        n743 = call "COM EvolutionBoard.vi"("error in (no error)"=w1888, "VISA resource name 2"=refnum<visa-resource-name> "COM1" ("VISA resource name")) -> ("error out"=w1884:errorcluster, "VISA resource name out"=w1883:refnum<visa-resource-name>)  [unwired: 8 in]
        n744 = call "TesterOption (SubVI).vi"("2 Options"=FALSE, "error in (no error)"=w1884, "On/Off"=FALSE, "Tester Option"=T11."Venable", "VISA Refnum in"=w1883) -> ("error out"=w1864:errorcluster, "VISA Refnum out"=→"VISA Tester":refnum<visa-resource-name>)  [unwired: 5 in]
        n745 = case shown="95" w1865 {
          tunnel: ["AHU Software Version" ("key") "EBAY Software Version" ("key")] -> w1874
          tunnel: ["AHU Serial Number" ("key") "EBAY Serial Number" ("key")] -> w1875
          frame 47, 63, Default {
          }
          frame 95 {
          }
        }
        n746 = call <vilib>:"Open Config Data.vi"("create file if necessary (T)"=FALSE, "configuration file path"=w1868) -> ("error out"=w1869:errorcluster, "refnum"=w1870:T24)  [unwired: 1 in, 7 out]
        n747 = call-poly <vilib>:"Read Key.vi"("section"=w1872, "error in (no error)"=w1869, "key"=w1874, "refnum"=w1870) -> ("error out"=w1876:errorcluster, "value"=→"UUT SoftwareVer":string, "refnum out"=w1873:T24)  [unwired: 2 in, 3 out]
        n748 = call-poly <vilib>:"Read Key.vi"("section"=w1872, "error in (no error)"=w1876, "key"=w1875, "refnum"=w1873) -> ("error out"=w1863:errorcluster, "value"=w1861:string, "refnum out"=w1862:T24)  [unwired: 2 in, 3 out]
        n749 = call <vilib>:"Close Config Data.vi"("error in (no error)"=w1863, "refnum"=w1862) -> ()  [unwired: 8 in, 2 out]
        n750 = Decimal String To Number(string=w1861) -> (number=w1866:i32)  [unwired: 2 in, 1 out]
        n751 = Increment(x=w1866) -> (x+1=→"Next SN":i32)
      }
      frame "Stop" {
        n752 = flat-sequence {
          tunnel: w1966 -> [w1982]
          tunnel: [w1981] -> w1959
          frame #0 {
            n753 = control-ref of="Pannel User Message"() -> (w1984:refnum<vi>)
            n754 = property class="Str"(reference=w1984, error in=w1982, "Value"="Program Stopped...\r\nPlease turn OFF All Power sinks") -> (error out=w1981:errorcluster)  [unwired: 1 out]
          }
        }
        n755 = control-ref of="VISA Tester"() -> (w1968:refnum<vi>)
        n756 = property class="VISAName"(reference=w1968, error in=w1959) -> ("Value"=w1965:refnum<visa-resource-name>)  [unwired: 2 out]
        n757 = call "Clear CAN Buffer.vi"("error in (no error)"=w1959, "Cluster in"=w1957) -> ("error out"=w1958:errorcluster)  [unwired: 8 in, 1 out]
        n758 = call "Close CAN Device.vi"("error in (no error)"=w1958, "Cluster in"=w1957) -> ()  [unwired: 8 in, 2 out]
        n759 = VISA Close(VISA resource name=w1976, error in (no error)=w1959) -> (error out=w1969:errorcluster)
        n760 = call "TesterOption (SubVI).vi"("2 Options"=FALSE, "On/Off"=FALSE, "Tester Option"=T11."Power", "VISA Refnum in"=w1965) -> ("error out"=w1952:errorcluster, "VISA Refnum out"=w1964:refnum<visa-resource-name>)  [unwired: 6 in]
        n761 = VISA Close(VISA resource name=w1964, error in (no error)=w1952) -> (error out=w1949:errorcluster)
        n762 = Flush Queue(queue=w1970, error in (no error)=w1969) -> (queue out=w1972:refnum<queue>, error out=w1971:errorcluster)  [unwired: 1 out]
        n763 = Flush Queue(queue=w1978, error in (no error)=w1969) -> (queue out=w1977:refnum<queue>, error out=w1979:errorcluster)  [unwired: 1 out]
        n764 = property on="Refresh Button" class="Bool (strict)"() -> ("Value"=w1956:bool)  [unwired: 2 in, 2 out]
        n765 = Release Queue(queue=w1972, error in (no error)=w1971) -> (error out=w1950:errorcluster)  [unwired: 1 in, 2 out]
        n766 = Release Queue(queue=w1977, error in (no error)=w1979) -> (error out=w1951:errorcluster)  [unwired: 1 in, 2 out]
        n767 = Select(t=T10."Initialize", s=w1956, f=T10."Stop") -> (s? t:f=w1953:T10)
        n768 = Merge Errors(w1951, w1950, w1949) -> (w1948:errorcluster)
        n769 = call <vilib>:"Clear Errors.vi"("error in (no error)"=w1948) -> ("error out"=w1947:errorcluster)  [unwired: 5 in, 1 out]
      }
      frame "MainProgram" {
        n770 = event shown="[12] \"Settings\": Value Change" {
          selector: w1990 -> [_ _ _ _ _ _ _ _ _ _ _ _ _]
          dyn-events: _ -> [_ _ _ _ _ _ _ _ _ _ _ _ _]
          timeout: 50 -> [_ _ _ _ _ _ _ _ _ _ _ _ _]
          tunnel: [T10."MainProgram" T10."MainProgram" T10."MainProgram" T10."MainProgram" T10."MainProgram" T10."MainProgram" T10."MainProgram" w2548 T10."MainProgram" T10."MainProgram" T10."MainProgram" T10."Stop" T10."MainProgram"] -> w2003
          tunnel: [w2009 w2122 w2176 w2183 w2192 w2210 w2217 w2608 w2663 w2676 w2684 w2764 w2770] -> w1997
          tunnel: w2001 -> [w2013 w2122 w2175 w2185 w2192 w2210 w2225 w2608 w2664 w2675 w2683 w2764 w2775]
          tunnel: [w2022 w2096 w2177 w2184 w2193 w2208 w2213 w2556 w2661 w2673 w2685 w2762 w2768] -> w1998
          tunnel: w1999 -> [w2022 w2096 w2177 w2184 w2193 w2208 w2213 w2556 w2661 w2673 _ w2762 w2768]
          tunnel: w1996 -> [w2015 w2128 w2171 w2180 w2189 w2207 w2222 w2588 w2660 w2672 w2688 w2761 w2773]
          tunnel: w1995 -> [w2010 w2127 w2172 w2181 w2190 w2206 w2223 w2587 w2659 w2671 w2687 w2760 w2766]
          tunnel: [w2012 w2127 w2172 w2181 w2190 w2206 w2223 w2587 w2659 w2671 w2687 w2760 w2766] -> w1994
          tunnel: [w2014 w2128 w2171 w2180 w2189 w2207 w2222 w2588 w2660 w2672 w2688 w2761 w2773] -> w1993
          tunnel: w1992 -> [w2007 w2126 w2170 w2179 w2188 w2205 w2221 w2586 w2658 w2670 w2686 w2759 w2772]
          tunnel: [w2007 w2126 w2170 w2179 w2188 w2205 w2216 w2586 w2658 w2670 w2686 w2759 w2772] -> w1991
          tunnel: w1989 -> [_ _ _ _ _ _ _ w2554 _ _ _ _ _]
          tunnel: w1988 -> [w2008 w2125 w2169 w2178 w2187 w2203 w2211 w2561 w2657 w2669 w2681 w2758 w2771]
          tunnel: [w2008 w2125 w2169 w2178 w2187 w2203 w2211 w2560 w2657 w2669 w2681 w2758 w2771] -> w1987
          tunnel: w1986 -> [_ w2123 _ _ _ _ _ w2559 _ _ _ _ _]
          tunnel: w1985 -> [_ w2094 _ _ _ _ _ _ _ _ _ _ _]
          event Timeout {
            n771 = event-data() -> ()  [unwired: 1 in, 3 out]
            n772 = property class="Clust (strict)"(reference=w2010, error in=w2013) -> (reference out=w2012:refnum<vi>, error out=w2011:errorcluster, "Value"=w2019:T7)
            n773 = Unbundle By Name(w2019) -> ("DevType"=w2020:T2, "CanIndex"=w2017:T1)
            n774 = call "VCI_Receive.vi"("CANIndex"=w2017, "DevIndex"=u32 0, "DevType"=w2020) -> ("Recieve"=w2016:T25[])  [unwired: 3 in, 5 out]
            n775 = Empty Array?(array=w2016) -> (empty?=w2018:bool)
            n776 = case shown="True" w2018 {
              tunnel: w2017 -> [w2059 _]
              tunnel: w2012 -> [w2057 _]
              tunnel: w2015 -> [w2056 w2091]
              tunnel: w2011 -> [w2055 w2090]
              tunnel: w2016 -> [w2060 _]
              tunnel: [w2050 w2090] -> w2009
              tunnel: [w2049 w2091] -> w2014
              frame False {
                n777 = call "Demo_MakeDispBuff.vi"("Channel"=w2059, "Type"=enum16{"接收", "发送"}."接收", "OBJs"=w2060) -> ("Buffer"=w2058:T26)
                n778 = for {
                  N: 3 -> [_]
                  tunnel: w2058 -> [w2074]
                  tunnel: w2057 -> [w2073]
                  tunnel: w2056 -> [w2064]
                  tunnel: w2055 -> [w2063]
                  tunnel: [w2066] -> w2053 mode=indexing
                  tunnel: [w2064] -> w2052
                  tunnel: [w2063] -> w2051
                  i -> [w2062]
                  n779 = property class="Clust (strict)"(reference=w2073) -> ("Value"=w2071:T7)  [unwired: 1 in, 2 out]
                  n780 = Index Array(array=w2074, index=w2062) -> (element=w2067:T27)
                  n781 = Unbundle By Name(w2067) -> ("Channel"=w2069:T1, "VCI_CAN_OBJ"=w2072:T25)  [unwired: 2 out]
                  n782 = Unbundle By Name(w2071) -> ("CanIndex"=w2070:T1)
                  n783 = Equal?(x=w2070, y=w2069) -> (x = y?=w2068:bool)
                  n784 = case shown="True" w2068 {
                    tunnel: w2072 -> [_ w2085]
                    tunnel: [w2075 w2081] -> w2066
                    tunnel: T21 {"ID"=0, "MSGTYPE"=0, "LEN"=0, "aDATA"=[]} ("Msg") -> [w2075 w2080]
                    frame False {
                    }
                    frame True {
                      n785 = Unbundle By Name(w2085) -> ("ID"=w2079:u32, "DataLen"=w2084:u8, "Data"=w2082:u8[])
                      n786 = Bundle By Name(cluster=w2080, "ID"=w2079, "MSGTYPE"=u8 0, "LEN"=w2084, "aDATA"=w2082) -> (w2081:T21)
                      n787 = Unbundle By Name(w2081) -> ("ID"=w2077:u32)
                      n788 = Split Number(x=w2077) -> (lo(x)=w2078:u16)  [unwired: 1 out]
                      n789 = Split Number(x=w2078) -> (lo(x)=w2076:u8)  [unwired: 1 out]
                      n790 = case shown="63" w2076 {
                        tunnel: ["EBAY 5F" "" "AHU 3F" "AHU 2F"] -> _
                        frame 95 {
                        }
                        frame Default {
                        }
                        frame 63 {
                        }
                        frame 47 {
                        }
                      }
                    }
                  }
                }
                n791 = Enqueue Element(queue=w2052, element=w2053, error in (no error)=w2051) -> (queue out=w2049:refnum<queue>, error out=w2050:errorcluster)  [unwired: 2 out]
              }
              frame True {
              }
            }
            n792 = disable-structure shown="Disabled" {
              frame Disabled {
                n793 = property on="SpeedResult" class="Bool (strict)"() -> ("Value"=w2036:bool)  [unwired: 2 in, 2 out]
                n794 = property on="VenableResult" class="Bool (strict)"() -> ("Value"=w2034:bool)  [unwired: 2 in, 2 out]
                n795 = property on="VenableDirectionResult" class="Bool (strict)"() -> ("Value"=w2035:bool)  [unwired: 2 in, 2 out]
                n796 = property on="ComTestResult" class="Bool (strict)"() -> ("Value"=w2033:bool)  [unwired: 2 in, 2 out]
                n797 = property on="AuxiOFFResult" class="Bool (strict)"() -> ("Value"=w2037:bool)  [unwired: 2 in, 2 out]
                n798 = property on="AuxiONResult" class="Bool (strict)"() -> ("Value"=w2038:bool)  [unwired: 2 in, 2 out]
                n799 = property on="VisualInspectionResult" class="Bool (strict)"() -> ("Value"=w2040:bool)  [unwired: 2 in, 2 out]
                n800 = property on="SensCalResult" class="Bool (strict)"() -> ("Value"=w2039:bool)  [unwired: 2 in, 2 out]
                n801 = property on="BurnDC" class="Bool (strict)"() -> ("Value"=w2041:bool)  [unwired: 2 in, 2 out]
                n802 = property on="BurnTemp" class="Bool (strict)"() -> ("Value"=w2042:bool)  [unwired: 2 in, 2 out]
                n803 = property on="BurnSpeed" class="Bool (strict)"() -> ("Value"=w2043:bool)  [unwired: 2 in, 2 out]
                n804 = property on="BurnResult" class="Bool (strict)"() -> ("Value"=w2044:bool)  [unwired: 2 in, 2 out]
                n805 = property on="StopTimeResult" class="Bool (strict)"() -> ("Value"=w2045:bool)  [unwired: 2 in, 2 out]
                n806 = property on="MotorTempResult" class="Bool (strict)"() -> ("Value"=w2046:bool)  [unwired: 2 in, 2 out]
                n807 = property on="TempControlResult" class="Bool (strict)"() -> ("Value"=w2047:bool)  [unwired: 2 in, 2 out]
                n808 = Build Array(w2033, w2034, w2035, w2036, w2037, w2038, w2039, w2040, w2041, w2042, w2043, w2044, w2045, w2046, w2047) -> (w2032:bool[])
                n809 = And Array Elements(Boolean array=w2032) -> (logical AND=w2048:bool)
                n810 = Not(x=w2048) -> ()  [unwired: 1 out]
              }
              frame Enabled {
              }
            }
            n811 = disable-structure shown="Disabled" {
              disable-tunnel: w2007 -> [w2027 _]
              frame Disabled {
                n812 = Preview Queue Element(queue=w2027) -> (element=w2026:T8)  [unwired: 2 in, 3 out]
                n813 = Unbundle By Name(w2026) -> ("Array Test"=w2025:T16)
                n814 = for {
                  tunnel: w2025 -> [w2030] mode=indexing
                  tunnel: [w2028] -> w2024 mode=indexing
                  n815 = Equal?(x=w2030, y=T20."Empty") -> (x = y?=w2028:bool)
                }
                n816 = And Array Elements(Boolean array=w2024) -> ()  [unwired: 1 out]
              }
              frame Enabled {
              }
            }
            n817 = property on="Automation" class="Bool (strict)"() -> ("Value"=w2004:bool)  [unwired: 2 in, 2 out]
            n818 = property on="Start" class="Bool (strict)"() -> ("Value"=w2006:bool)  [unwired: 2 in, 2 out]
            n819 = Or(x=w2004, y=w2006) -> (x .or. y?=w2005:bool)
            n820 = case shown="False" w2005 {
              frame False {
                n821 = property on="Pannel User Message" class="Str"("Value"="You can press start to execute(s) test(s).") -> ()  [unwired: 2 in, 2 out]
              }
              frame True {
              }
            }
          }
          event "SetSN": Value Change {
            n822 = event-data() -> ()  [unwired: 1 in, 6 out]
            n823 = property on="SpeedResult" class="Bool (strict)"() -> ("Value"=w2105:bool)  [unwired: 2 in, 2 out]
            n824 = property on="VenableResult" class="Bool (strict)"() -> ("Value"=w2103:bool)  [unwired: 2 in, 2 out]
            n825 = property on="VenableDirectionResult" class="Bool (strict)"() -> ("Value"=w2104:bool)  [unwired: 2 in, 2 out]
            n826 = property on="ComTestResult" class="Bool (strict)"() -> ("Value"=w2102:bool)  [unwired: 2 in, 2 out]
            n827 = property on="UUT" class="DigNum (strict)"() -> ("Value"=w2100:u8)  [unwired: 2 in, 2 out]
            n828 = property on="Current SN" class="DigNum (strict)"(error in=w2122) -> ("Value"=w2121:i32)  [unwired: 1 in, 2 out]
            n829 = case shown="95" w2100 {
              tunnel: [w2165 w2168] -> w2116
              tunnel: [w2165 w2167] -> w2107
              tunnel: [w2165 w2166] -> w2106
              frame 47, 63, Default {
                w2165 = TRUE ("Value")
              }
              frame 95 {
                n830 = property on="AuxiOFFResult" class="Bool (strict)"() -> ("Value"=w2166:bool)  [unwired: 2 in, 2 out]
                n831 = property on="AuxiONResult" class="Bool (strict)"() -> ("Value"=w2167:bool)  [unwired: 2 in, 2 out]
                n832 = property on="TempControlResult" class="Bool (strict)"() -> ("Value"=w2168:bool)  [unwired: 2 in, 2 out]
              }
            }
            n833 = property on="VisualInspectionResult" class="Bool (strict)"() -> ("Value"=w2109:bool)  [unwired: 2 in, 2 out]
            n834 = property on="SensCalResult" class="Bool (strict)"() -> ("Value"=w2108:bool)  [unwired: 2 in, 2 out]
            n835 = Equal To 0?(x=w2121) -> (x = 0?=w2118:bool)
            n836 = Equal?(x=w2121, y=-1) -> (x = y?=w2119:bool)
            n837 = Or(x=w2119, y=w2118) -> (x .or. y?=w2099:bool)
            n838 = property on="BurnDC" class="Bool (strict)"() -> ("Value"=w2110:bool)  [unwired: 2 in, 2 out]
            n839 = property on="BurnTemp" class="Bool (strict)"() -> ("Value"=w2111:bool)  [unwired: 2 in, 2 out]
            n840 = property on="BurnSpeed" class="Bool (strict)"() -> ("Value"=w2112:bool)  [unwired: 2 in, 2 out]
            n841 = property on="BurnResult" class="Bool (strict)"() -> ("Value"=w2113:bool)  [unwired: 2 in, 2 out]
            n842 = property on="StopTimeResult" class="Bool (strict)"() -> ("Value"=w2114:bool)  [unwired: 2 in, 2 out]
            n843 = property on="MotorTempResult" class="Bool (strict)"() -> ("Value"=w2115:bool)  [unwired: 2 in, 2 out]
            n844 = property on="Automation" class="Bool (strict)"() -> ("Value"=w2092:bool)  [unwired: 2 in, 2 out]
            n845 = Build Array(w2102, w2103, w2104, w2105, w2106, w2107, w2108, w2109, w2110, w2111, w2112, w2113, w2114, w2115, w2116) -> (w2101:bool[])
            n846 = And Array Elements(Boolean array=w2101) -> (logical AND=w2117:bool)
            n847 = Not(x=w2117) -> (.not. x?=w2098:bool)
            n848 = Select(t=w2098, s=w2092, f=w2094) -> (s? t:f=w2097:bool)
            n849 = And(x=w2099, y=w2097) -> (x .and. y?=w2095:bool)
            n850 = case shown="True" w2095 {
              tunnel: w2123 -> [_ w2158]
              tunnel: w2096 -> [_ w2151]
              tunnel: w2092 -> [w2131 _]
              tunnel: [w2130 w2142] -> w2093
              frame False {
                n851 = case shown="True" w2131 {
                  tunnel: [w2132 w2133] -> w2130
                  frame False {
                    n852 = call "Display Message to User9"() -> ("error out"=w2132:errorcluster)  [unwired: 10 in, 1 out]
                  }
                  frame True {
                    n853 = call "Display Message to User3"() -> ("error out"=w2133:errorcluster)  [unwired: 10 in, 1 out]
                  }
                }
              }
              frame True {
                w2150 = FALSE ("SetSN")
                n854 = property on="Next SN" class="DigNum (strict)"() -> ("Value"=w2147:i32)  [unwired: 2 in, 2 out]
                n855 = property on="VISA Tester" class="VISAName"() -> ("Value"=w2140:refnum<visa-resource-name>)  [unwired: 2 in, 2 out]
                n856 = call "TesterOption (SubVI).vi"("2 Options"=FALSE, "On/Off"=FALSE, "Tester Option"=T11."Venable", "VISA Refnum in"=w2140) -> ("error out"=w2135:errorcluster)  [unwired: 6 in, 1 out]
                n857 = call <vilib>:"Clear Errors.vi"("error in (no error)"=w2135) -> ("error out"=w2136:errorcluster)  [unwired: 5 in, 1 out]
                n858 = Number To Decimal String(number=w2147) -> (decimal integer string=w2134:string)  [unwired: 1 in]
                "UUT SN Report" <- w2134
                n859 = Search and Replace String(input string="EP=1\r\nSN=0\r\n" ("write buffer"), search string="0", replace string=w2134) -> (result string=w2153:string)  [unwired: 5 in, 3 out]
                n860 = call "SerialMarvinSendGet.vi"("error in (no error)"=w2136, "Clear Log"=FALSE, "write buffer"=w2153, "VISA resource name"=w2151) -> ("error out"=w2141:errorcluster)  [unwired: 6 in, 1 out]
                n861 = property on="UUT" class="DigNum (strict)"(error in=w2141) -> ("Value"=w2159:u8)  [unwired: 1 in, 2 out]
                n862 = case shown="47, 63, Default" w2159 {
                  tunnel: ["AHU Serial Number" ("key") "EBAY Serial Number" ("key")] -> w2162
                  frame 47, 63, Default {
                  }
                  frame 95 {
                  }
                }
                n863 = call <vilib>:"Open Config Data.vi"("create file if necessary (T)"=FALSE, "configuration file path"=w2158) -> ("error out"=w2156:errorcluster, "refnum"=w2157:T24)  [unwired: 1 in, 7 out]
                n864 = call-poly <vilib>:"Write Key.vi"("section"="Marvin", "error in (no error)"=w2156, "value"=w2134, "key"=w2162, "refnum"=w2157) -> ("error out"=w2145:errorcluster, "refnum out"=w2144:T24)  [unwired: 4 in, 1 out]
                n865 = call <vilib>:"Close Config Data.vi"("error in (no error)"=w2145, "refnum"=w2144) -> ("error out"=w2143:errorcluster)  [unwired: 8 in, 1 out]
                n866 = property on="SetSN" class="Bool (strict)"(error in=w2143, "Value"=w2150) -> (error out=w2149:errorcluster)  [unwired: 1 in, 1 out]
                n867 = property on="Automation" class="Bool (strict)"(error in=w2149, "Value"=w2150) -> (error out=w2148:errorcluster)  [unwired: 1 in, 1 out]
                n868 = Increment(x=w2147) -> (x+1=w2146:i32)
                n869 = property on="Next SN" class="DigNum (strict)"(error in=w2148, "Value"=w2146) -> (error out=w2142:errorcluster)  [unwired: 1 in, 1 out]
              }
            }
            n870 = case shown="True" w2092 {
              tunnel: w2093 -> [_ _]
              frame False {
              }
              frame True {
                w2129 = TRUE ("Value (Signaling)")
                n871 = property on="Report" class="Bool (strict)"("Val(Sgnl)"=w2129, "Value"=w2129) -> ()  [unwired: 2 in, 2 out]
              }
            }
          }
          event "ATR": Mouse Enter {
            n872 = event-data() -> ()  [unwired: 1 in, 4 out]
            n873 = call-poly <vilib>:"Set Cursor.vi"("error in (no error)"=w2175, "icon"=u16 1) -> ("error out"=w2176:errorcluster)  [unwired: 8 in, 1 out]
          }
          event "ATR": Mouse Leave {
            n874 = event-data() -> ()  [unwired: 1 in, 4 out]
            n875 = call-poly <vilib>:"Set Cursor.vi"("error in (no error)"=w2185, "icon"=u16 0) -> ("error out"=w2183:errorcluster)  [unwired: 8 in, 1 out]
          }
          event "ATR": Mouse Down? {
            n876 = event-data() -> ("Coords"=w2200:T28)  [unwired: 1 in, 4 out]
            n877 = invoke on="ATR" class="Tbl (strict)" method="Point To Row Column"("Point"=w2200) -> ("InBounds"=w2196:bool, "CellPosition"=w2195:T19)  [unwired: 5 in, 4 out]
            n878 = Greater Than 0?(x=w2195) -> (x > 0?=w2199:cluster{"Row":bool, "Column":bool})
            n879 = Cluster To Array(cluster=w2199) -> (array=w2198:bool[])
            n880 = Or Array Elements(Boolean array=w2198) -> (logical OR=w2197:bool)
            n881 = Or(x=w2196, y=w2197) -> (x .or. y?=w2194:bool)
            n882 = event-data("Discard?"=w2194) -> ()  [unwired: 1 in, 1 out]
          }
          event Panel Close? {
            w2202 = TRUE ("Stop Button")
            n883 = event-data() -> ("VIRef"=w2204:refnum<vi>)  [unwired: 1 in, 3 out]
            n884 = Close Reference(reference=w2204) -> ()  [unwired: 1 in, 1 out]
            n885 = property on="Stop Button" class="Bool (strict)"("Value"=w2202, "Val(Sgnl)"=w2202) -> ()  [unwired: 2 in, 2 out]
            n886 = event-data("Discard?"=TRUE) -> ()  [unwired: 1 in, 1 out]
          }
          event "Start": Value Change {
            w2212 = T16 [] items=["Auxiliary", "Temp Sens Cal", "Com Test", "Enable Test", "Speed Command", "Stop Time", "Temp Control", "Burn in", "Visual Inspec", "Empty"]
            n887 = event-data() -> ()  [unwired: 1 in, 2 out]
            n888 = property on="UUT" class="Str"(error in=w2225) -> ("Value"=w2224:string)  [unwired: 1 in, 2 out]
            n889 = while {
              tunnel: w2224 -> [w2241]
              tunnel: [w2240] -> w2219
              tunnel: [w2239] -> w2218
              shift-right: [w2232] -> _
              shift-left: enum16{"Stop", "Tests", "Bit test", "Start"}."Start" -> [w2238]
              tunnel: w2213 -> [w2237]
              tunnel: w2212 -> [w2231]
              stop <- w2230 stop-if-true
              n890 = control-ref of="Pannel User Message"() -> (w2236:refnum<vi>)
              n891 = control-ref of="Stop Button"() -> (w2235:refnum<vi>)
              n892 = control-ref of="Motor Speed RPM"() -> (w2233:refnum<vi>)
              n893 = control-ref of="Stop Burn-in"() -> (w2234:refnum<vi>)
              n894 = property on="Status" class="Bool (strict)"() -> (error out=w2227:errorcluster, "Value"=w2229:bool)  [unwired: 2 in, 1 out]
              n895 = property on="VISA Tester" class="VISAName"() -> ("Value"=w2228:refnum<visa-resource-name>)  [unwired: 2 in, 2 out]
              n896 = case shown="\"Start\"" w2238 {
                tunnel: w2241 -> [_ w2256 w2366 _]
                tunnel: [w2246 w2255 w2401 w2505] -> w2240
                tunnel: [w2242 w2254 w2364 w2504] -> w2239
                tunnel: w2237 -> [_ _ w2382 w2510]
                tunnel: w2236 -> [_ _ _ w2509]
                tunnel: w2235 -> [_ _ _ w2508]
                tunnel: w2234 -> [_ _ _ w2507]
                tunnel: w2233 -> [_ _ _ w2506]
                tunnel: [w2245 w2253 w2369 w2500] -> w2232
                tunnel: w2231 -> [w2246 _ w2401 w2505]
                tunnel: [w2244 w2252 FALSE FALSE] -> w2230
                tunnel: w2229 -> [_ _ _ w2502]
                tunnel: w2228 -> [_ _ w2383 _]
                tunnel: w2227 -> [w2242 _ _ _]
                frame "Stop", Default {
                  n897 = property on="Start" class="Bool (strict)"(error in=w2242, "Value"=FALSE ("Start")) -> ()  [unwired: 1 in, 2 out]
                  n898 = flat-sequence {
                    tunnel: [enum16{"Stop", "Tests", "Bit test", "Start"}."Stop"] -> w2245
                    tunnel: w2242 -> [_]
                    tunnel: [TRUE] -> w2244
                    frame #0 {
                    }
                  }
                }
                frame "Tests" {
                  w2249 = FALSE ("Stop Burn-in")
                  w2251 = T18."Disabled and Grayed Out" ("Disabled")
                  n899 = case shown="\"AHU\", Default" w2256 {
                    tunnel: [w2271 w2320] -> w2255
                    tunnel: [w2270 w2319] -> w2254
                    tunnel: [w2259 w2307] -> w2250
                    frame "AHU", Default {
                      n900 = call "Load Program Process AHU.vi"() -> ("Speed Command Test"=w2264:bool, "Enable Test"=w2265:bool, "Burn-in Test"=w2262:bool, "Auxiliary"=w2260:bool, "Temperature Sensor Calibration Test"=w2267:bool, "Communication Test"=w2266:bool, "Stop Time Test"=w2263:bool, "Visual Inspection"=w2261:bool, "OK"=w2268:bool, "Automation"=w2259:bool, "error out"=w2270:errorcluster)  [unwired: 8 in, 9 out]
                      n901 = Or(x=w2268, y=w2259) -> (x .or. y?=w2269:bool)
                      n902 = case shown="True" w2269 {
                        tunnel: [w2272 w2282] -> w2271
                        tunnel: w2259 -> [_ w2281]
                        tunnel: w2267 -> [_ w2280]
                        tunnel: w2266 -> [_ w2279]
                        tunnel: w2265 -> [_ w2278]
                        tunnel: w2264 -> [_ w2277]
                        tunnel: w2263 -> [_ w2276]
                        tunnel: w2262 -> [_ w2275]
                        tunnel: w2261 -> [_ w2274]
                        tunnel: w2260 -> [_ w2273]
                        frame False {
                          w2272 = T16 [] items=["Auxiliary", "Temp Sens Cal", "Com Test", "Enable Test", "Speed Command", "Stop Time", "Temp Control", "Burn in", "Visual Inspec", "Empty"]
                        }
                        frame True {
                          n903 = case shown="False" w2281 {
                            tunnel: [w2305 w2306] -> w2282
                            tunnel: w2280 -> [w2287 _]
                            tunnel: w2279 -> [w2286 _]
                            tunnel: w2278 -> [w2288 _]
                            tunnel: w2277 -> [w2285 _]
                            tunnel: w2276 -> [w2284 _]
                            tunnel: w2275 -> [w2298 _]
                            tunnel: w2274 -> [w2283 _]
                            tunnel: w2273 -> [_ _]
                            frame False {
                              w2291 = T20."Empty" ("f")
                              n904 = Select(t=T20."Com Test" ("f"), s=w2286, f=w2291) -> (s? t:f=w2297:T20)
                              n905 = Select(t=T20."Temp Sens Cal" ("f"), s=w2287, f=w2291) -> (s? t:f=w2296:T20)
                              n906 = Select(t=T20."Stop Time" ("f"), s=w2284, f=w2291) -> (s? t:f=w2295:T20)
                              n907 = Select(t=T20."Enable Test" ("f"), s=w2288, f=w2291) -> (s? t:f=w2294:T20)
                              n908 = Select(t=T20."Speed Command" ("f"), s=w2285, f=w2291) -> (s? t:f=w2293:T20)
                              n909 = Select(t=T20."Burn in" ("f"), s=w2298, f=w2291) -> (s? t:f=w2292:T20)
                              n910 = Select(t=T20."Visual Inspec" ("f"), s=w2283, f=w2291) -> (s? t:f=w2289:T20)
                              n911 = Build Array(w2297, w2296, w2295, w2294, w2293, w2292, w2289) -> (w2305:T16)
                            }
                            frame True {
                              w2306 = T16 [enum."Com Test", enum."Temp Sens Cal", enum."Stop Time", enum."Enable Test", enum."Speed Command", enum."Burn in", enum."Visual Inspec"] items=["Auxiliary", "Temp Sens Cal", "Com Test", "Enable Test", "Speed Command", "Stop Time", "Temp Control", "Burn in", "Visual Inspec", "Empty"]
                            }
                          }
                        }
                      }
                    }
                    frame "EBAY" {
                      n912 = call "Load Program Process EBAY.vi"() -> ("Speed Command Test"=w2313:bool, "Enable Test"=w2314:bool, "Burn-in Test"=w2311:bool, "Temperature Control Algorithm Test"=w2310:bool, "Auxiliary"=w2308:bool, "Temperature Sensor Calibration Test"=w2316:bool, "Communication Test"=w2315:bool, "Stop Time Test"=w2312:bool, "Visual Inspection"=w2309:bool, "OK"=w2317:bool, "Automation"=w2307:bool, "error out"=w2319:errorcluster)  [unwired: 8 in, 8 out]
                      n913 = Or(x=w2317, y=w2307) -> (x .or. y?=w2318:bool)
                      n914 = case shown="True" w2318 {
                        tunnel: [w2321 w2332] -> w2320
                        tunnel: w2307 -> [_ w2331]
                        tunnel: w2316 -> [_ w2330]
                        tunnel: w2315 -> [_ w2329]
                        tunnel: w2314 -> [_ w2328]
                        tunnel: w2313 -> [_ w2327]
                        tunnel: w2312 -> [_ w2326]
                        tunnel: w2311 -> [_ w2325]
                        tunnel: w2310 -> [_ w2324]
                        tunnel: w2309 -> [_ w2323]
                        tunnel: w2308 -> [_ w2322]
                        frame False {
                          w2321 = T16 [] items=["Auxiliary", "Temp Sens Cal", "Com Test", "Enable Test", "Speed Command", "Stop Time", "Temp Control", "Burn in", "Visual Inspec", "Empty"]
                        }
                        frame True {
                          n915 = case shown="False" w2331 {
                            tunnel: [w2361 w2362] -> w2332
                            tunnel: w2330 -> [w2337 _]
                            tunnel: w2329 -> [w2336 _]
                            tunnel: w2328 -> [w2335 _]
                            tunnel: w2327 -> [w2334 _]
                            tunnel: w2326 -> [w2333 _]
                            tunnel: w2325 -> [w2339 _]
                            tunnel: w2324 -> [w2338 _]
                            tunnel: w2323 -> [w2352 _]
                            tunnel: w2322 -> [w2343 _]
                            frame False {
                              w2341 = T20."Empty" ("f")
                              n916 = Select(t=T20."Com Test" ("f"), s=w2336, f=w2341) -> (s? t:f=w2351:T20)
                              n917 = Select(t=T20."Temp Sens Cal" ("f"), s=w2337, f=w2341) -> (s? t:f=w2350:T20)
                              n918 = Select(t=T20."Stop Time" ("f"), s=w2333, f=w2341) -> (s? t:f=w2349:T20)
                              n919 = Select(t=T20."Enable Test" ("f"), s=w2335, f=w2341) -> (s? t:f=w2348:T20)
                              n920 = Select(t=T20."Speed Command" ("f"), s=w2334, f=w2341) -> (s? t:f=w2347:T20)
                              n921 = Select(t=T20."Temp Control" ("f"), s=w2338, f=w2341) -> (s? t:f=w2346:T20)
                              n922 = Select(t=T20."Burn in" ("f"), s=w2339, f=w2341) -> (s? t:f=w2345:T20)
                              n923 = Select(t=T20."Visual Inspec" ("f"), s=w2352, f=w2341) -> (s? t:f=w2344:T20)
                              n924 = Select(t=T20."Auxiliary" ("f"), s=w2343, f=w2341) -> (s? t:f=w2340:T20)
                              n925 = Build Array(w2351, w2350, w2349, w2348, w2347, w2346, w2345, w2340, w2344) -> (w2361:T16)
                            }
                            frame True {
                              w2362 = T16 [enum."Com Test", enum."Temp Sens Cal", enum."Stop Time", enum."Enable Test", enum."Speed Command", enum."Temp Control", enum."Burn in", enum."Auxiliary", enum."Visual Inspec"] items=["Auxiliary", "Temp Sens Cal", "Com Test", "Enable Test", "Speed Command", "Stop Time", "Temp Control", "Burn in", "Visual Inspec", "Empty"]
                            }
                          }
                        }
                      }
                    }
                  }
                  "Automation" <- w2250
                  n926 = flat-sequence {
                    tunnel: [enum16{"Stop", "Tests", "Bit test", "Start"}."Tests"] -> w2253
                    tunnel: [TRUE] -> w2252
                    frame #0 {
                    }
                  }
                  n927 = property on="Stop Button" class="Bool (strict)"("Value"=w2249) -> ()  [unwired: 2 in, 2 out]
                  n928 = property on="Stop Burn-in" class="Bool (strict)"("Value"=w2249) -> ()  [unwired: 2 in, 2 out]
                  n929 = property on="Start" class="Bool (strict)"("DisabledEnum"=w2251) -> ()  [unwired: 2 in, 2 out]
                  n930 = property on="Report" class="Bool (strict)"("DisabledEnum"=w2251) -> ()  [unwired: 2 in, 2 out]
                }
                frame "Bit test" {
                  # "Stop"
                  n931 = call "SerialMarvinSendGet.vi"("write buffer"="TA[1]\r\n", "VISA resource name"=w2382) -> ("error out"=w2395:errorcluster, "read buffer"=w2398:string)  [unwired: 8 in]
                  n932 = Fract/Exp String To Number(string=w2398) -> (number=w2397:dbl)  [unwired: 3 in, 1 out]
                  n933 = Less Or Equal?(x=w2397, y=100.0) -> (x <= y?=w2380:bool)
                  n934 = call "TesterOption (SubVI).vi"("On/Off 2"=FALSE, "Tester Option 2"=T11."Venable", "2 Options"=TRUE, "error in (no error)"=w2395, "On/Off"=TRUE, "Tester Option"=T11."25C", "VISA Refnum in"=w2383) -> ("error out"=w2385:errorcluster)  [unwired: 3 in, 1 out]
                  n935 = call "Time Delay5"("error in (no error)"=w2385) -> ("error out"=w2384:errorcluster)  [unwired: 10 in]
                  n936 = call "SerialMarvinSendGet.vi"("error in (no error)"=w2384, "write buffer"="TA[2]\r\n", "VISA resource name"=w2382) -> ("error out"=w2381:errorcluster, "read buffer"=w2387:string)  [unwired: 7 in]
                  n937 = case shown="\"AHU\"" w2366 {
                    tunnel: w2383 -> [w2431 _ w2459]
                    tunnel: w2382 -> [_ _ w2462]
                    tunnel: w2381 -> [w2432 w2450 w2461]
                    tunnel: [w2425 w2450 w2457] -> w2368
                    tunnel: [w2422 "" w2452] -> w2375
                    tunnel: [w2421 bool[] [] w2451] -> w2373
                    frame "AHU" {
                      n938 = call "TesterOption (SubVI).vi"("On/Off 2"=FALSE, "Tester Option 2"=T11."Venable", "2 Options"=TRUE, "error in (no error)"=w2432, "On/Off"=TRUE, "Tester Option"=T11."K17", "VISA Refnum in"=w2431) -> ("error out"=w2434:errorcluster)  [unwired: 3 in, 1 out]
                      n939 = call "Time Delay7"("error in (no error)"=w2434) -> ("error out"=w2433:errorcluster)  [unwired: 10 in]
                      n940 = call "GetADCTester (SubVI).vi"("error in (no error)"=w2433, "GetADCTester"=T13."Current", "TimeToGet"=5, "VISA Refnum in"=w2431) -> ("error out"=w2425:errorcluster, "ADCValOutput Single"=w2427:dbl)  [unwired: 5 in, 1 out]
                      n941 = Less Or Equal?(x=w2427, y=50.0) -> (x <= y?=w2426:bool)
                      n942 = Build Array(w2426) -> (w2421:bool[])
                      n943 = for {
                        tunnel: w2421 -> [w2447] mode=indexing
                        tunnel: string[] ["CURRENT OPERATION FAILED!"] -> [w2443] mode=indexing
                        shift-right: [w2445] -> w2422
                        shift-left: "" -> [w2444]
                        n944 = Concatenate Strings(w2443, "  TEST FAILED!" ("string"), "\r\n") -> (w2440:string)
                        n945 = Select(t=w2440, s=w2447, f=w2444) -> (s? t:f=w2446:string)
                        n946 = Concatenate Strings(w2444, w2446) -> (w2445:string)
                      }
                    }
                    frame Default {
                    }
                    frame "EBAY" {
                      w2460 = T29 [enum."Fan", enum."Current"] items=["Term1", "Term2", "Current", "Fan", "TempCPU"]
                      n947 = call "TesterOption (SubVI).vi"("On/Off 2"=FALSE, "Tester Option 2"=T11."Venable", "2 Options"=TRUE, "error in (no error)"=w2461, "On/Off"=TRUE, "Tester Option"=T11."K17", "VISA Refnum in"=w2459) -> ("error out"=w2464:errorcluster)  [unwired: 3 in, 1 out]
                      n948 = call "Time Delay6"("error in (no error)"=w2464) -> ("error out"=w2463:errorcluster)  [unwired: 10 in]
                      n949 = call "SerialMarvinSendGet.vi"("error in (no error)"=w2463, "write buffer"="TA[3]\r\n", "VISA resource name"=w2462) -> ("error out"=w2458:errorcluster, "read buffer"=w2466:string)  [unwired: 7 in]
                      n950 = Fract/Exp String To Number(string=w2466) -> (number=w2467:dbl)  [unwired: 3 in, 1 out]
                      n951 = for {
                        tunnel: w2460 -> [w2491] mode=indexing
                        tunnel: w2459 -> [w2490]
                        tunnel: w2458 -> [w2488]
                        tunnel: [w2487] -> w2457
                        tunnel: [w2484] -> w2455 mode=indexing
                        i -> [w2485]
                        n952 = call "GetADCTester (SubVI).vi"("error in (no error)"=w2488, "GetADCTester"=w2491, "TimeToGet"=0, "VISA Refnum in"=w2490) -> ("error out"=w2487:errorcluster, "ADCValOutput Single"=w2486:dbl)  [unwired: 5 in, 1 out]
                        n953 = case shown="1" w2485 {
                          tunnel: w2486 -> [w2494 w2497 _]
                          tunnel: [w2492 w2495 FALSE] -> w2484
                          frame 1 {
                            n954 = Less Or Equal?(x=w2494, y=50.0) -> (x <= y?=w2492:bool)
                          }
                          frame 0 {
                            n955 = Greater Or Equal?(x=w2497, y=2200.0) -> (x >= y?=w2495:bool)
                          }
                          frame Default {
                          }
                        }
                      }
                      n956 = Less Or Equal?(x=w2467, y=100.0) -> (x <= y?=w2456:bool)
                      n957 = Build Array (concatenate)(w2456, w2455) -> (w2451:bool[])
                      n958 = for {
                        tunnel: w2451 -> [w2474] mode=indexing
                        tunnel: string[] ["TA[3] OPERATION FAILED!", "EBAY FAN OPERATION FAILED!", "CURRENT OPERATION FAILED!"] -> [w2477] mode=indexing
                        shift-right: [w2479] -> w2452
                        shift-left: "" -> [w2478]
                        n959 = Concatenate Strings(w2477, "\r\n") -> (w2475:string)
                        n960 = case shown="False" w2474 {
                          tunnel: [w2482 w2483] -> w2479
                          tunnel: w2478 -> [w2481 w2483]
                          tunnel: w2475 -> [w2480 _]
                          frame False {
                            n961 = Concatenate Strings(w2481, w2480) -> (w2482:string)
                          }
                          frame True {
                          }
                        }
                      }
                    }
                  }
                  n962 = Fract/Exp String To Number(string=w2387) -> (number=w2388:dbl)  [unwired: 3 in, 1 out]
                  n963 = Less Or Equal?(x=w2388, y=100.0) -> (x <= y?=w2379:bool)
                  n964 = Build Array(w2380, w2379) -> (w2374:bool[])
                  n965 = for {
                    tunnel: w2374 -> [w2410] mode=indexing
                    tunnel: string[] ["TA[1] OPERATION FAILED!", "TA[2] OPERATION FAILED!"] -> [w2414] mode=indexing
                    shift-right: [w2416] -> w2376
                    shift-left: "" -> [w2415]
                    tunnel: w2368 -> [w2411]
                    tunnel: [w2411] -> w2367
                    n966 = Concatenate Strings(w2414, "\r\n") -> (w2412:string)
                    n967 = case shown="False" w2410 {
                      tunnel: [w2419 w2420] -> w2416
                      tunnel: w2415 -> [w2418 w2420]
                      tunnel: w2412 -> [w2417 _]
                      frame False {
                        n968 = Concatenate Strings(w2418, w2417) -> (w2419:string)
                      }
                      frame True {
                      }
                    }
                  }
                  n969 = Build Array (concatenate)(w2374, w2373) -> (w2372:bool[])
                  n970 = And Array Elements(Boolean array=w2372) -> (logical AND=w2363:bool)
                  n971 = case shown="False" w2363 {
                    tunnel: w2376 -> [w2408 _]
                    tunnel: w2375 -> [w2407 _]
                    tunnel: w2367 -> [w2405 w2409]
                    tunnel: [w2405 w2409] -> w2365
                    frame False {
                      n972 = Concatenate Strings(w2408, w2407) -> (w2406:string)
                      n973 = One Button Dialog(message=w2406) -> ()  [unwired: 1 in, 1 out]
                    }
                    frame True {
                    }
                  }
                  n974 = case shown="True" w2363 {
                    tunnel: w2365 -> [w2403 w2404]
                    tunnel: [w2402 w2404] -> w2364
                    frame False {
                      n975 = call "Display Message to User6"("error in (no error)"=w2403) -> ("error out"=w2402:errorcluster)  [unwired: 9 in, 1 out]
                    }
                    frame True {
                    }
                  }
                  n976 = Select(t=enum16{"Stop", "Tests", "Bit test", "Start"}."Tests", s=w2363, f=enum16{"Stop", "Tests", "Bit test", "Start"}."Tests") -> (s? t:f=w2369:enum16{"Stop", "Tests", "Bit test", "Start"})
                }
                frame "Start" {
                  n977 = case shown="True" w2502 {
                    tunnel: w2510 -> [_ w2537]
                    tunnel: w2509 -> [_ w2528]
                    tunnel: w2508 -> [_ w2524]
                    tunnel: w2507 -> [_ w2522]
                    tunnel: w2506 -> [_ w2521]
                    tunnel: [FALSE w2520] -> w2501
                    tunnel: [w2516 w2519] -> w2504
                    tunnel: [FALSE TRUE] -> w2499
                    frame False {
                      n978 = call "Display Message to User5"() -> ("error out"=w2516:errorcluster)  [unwired: 10 in, 1 out]
                    }
                    frame True {
                      n979 = property on="VISA Tester" class="VISAName"() -> (error out=w2535:errorcluster, "Value"=w2534:refnum<visa-resource-name>)  [unwired: 2 in, 1 out]
                      n980 = call "TesterOption (SubVI).vi"("2 Options"=FALSE, "error in (no error)"=w2535, "On/Off"=FALSE, "Tester Option"=T11."Venable", "VISA Refnum in"=w2534) -> ("error out"=w2530:errorcluster)  [unwired: 5 in, 1 out]
                      n981 = call "Write panel message (SubVI).vi"("Stop BurnIn"=w2522, 4:"rpm"=w2521, 5:"rpm"=FALSE ("rpm"), "PrintTime"=FALSE, "Stop"=w2524, "error in (no error)"=w2530, "Time to wait"=3.0, "Strin"="TESTER BIT TEST OPERATION IN PROCESS", "String in"=w2528) -> ("error out"=w2529:errorcluster)  [unwired: 2 in]
                      n982 = property on="UUT SoftwareVer" class="Str"() -> ("Value"=w2518:string)  [unwired: 2 in, 2 out]
                      n983 = call "SerialMarvinSendGet.vi"("error in (no error)"=w2529, "write buffer"="VR\r\n", "VISA resource name"=w2537) -> ("error out"=w2519:errorcluster, "read buffer"=w2536:string)  [unwired: 7 in]
                      n984 = Equal?(x=w2536, y=w2518) -> (x = y?=w2520:bool)
                    }
                  }
                  n985 = case shown="False" w2501 {
                    tunnel: [enum16{"Stop", "Tests", "Bit test", "Start"}."Stop" enum16{"Stop", "Tests", "Bit test", "Start"}."Bit test"] -> w2500
                    tunnel: w2499 -> [w2511 _]
                    frame False {
                      n986 = case shown="True" w2511 {
                        frame False {
                        }
                        frame True {
                          n987 = call "Display Message to User4"() -> ()  [unwired: 10 in, 2 out]
                        }
                      }
                    }
                    frame True {
                    }
                  }
                }
              }
            }
            n988 = Bundle By Name(cluster=T8 {"VISA"="COM1", "Array Test"=[]}, "VISA"=w2213, "Array Test"=w2219) -> (w2215:T8)
            n989 = Enqueue Element(queue=w2221, element=w2215, error in (no error)=w2218) -> (queue out=w2216:refnum<queue>, error out=w2217:errorcluster)  [unwired: 2 out]
          }
          event "Report", "Stop Button": Value Change {
            w2567 = "Marvin" ("section")
            n990 = event-data() -> ("CtlRef"=w2552:refnum<vi>)  [unwired: 1 in]
            n991 = local read "UUT"() -> (w2563:string)
            n992 = call <vilib>:"Application Directory.vi"() -> ("Application Directory"=w2595:path)
            n993 = Build Path(base path=w2595, name or relative path="Reports") -> (appended path=w2598:path)
            n994 = property on="Status" class="Bool (strict)"() -> ("Value"=w2557:bool)  [unwired: 2 in, 2 out]
            n995 = case shown="\"EBAY\", Default" w2563 {
              tunnel: ["REV EBAY" ("key") "REV AHU" ("key")] -> w2565
              frame "EBAY", Default {
              }
              frame "AHU" {
              }
            }
            n996 = call <vilib>:"Check if File or Folder Exists.vi"("path"=w2598) -> ("error out"=w2596:errorcluster, "file or folder exists?"=w2599:bool, "dup path"=w2597:path)  [unwired: 8 in]
            n997 = case shown="False" w2599 {
              tunnel: w2596 -> [w2654 w2655]
              tunnel: w2597 -> [w2653 w2656]
              tunnel: [w2652 w2656] -> w2604
              tunnel: [w2651 w2655] -> w2601
              frame False {
                n998 = Create Folder(path (use dialog)=w2653, error in=w2654) -> (created path=w2652:path, error out=w2651:errorcluster)  [unwired: 1 in, 1 out]
              }
              frame True {
              }
            }
            n999 = case shown="True" w2557 {
              tunnel: [w2611 w2620] -> w2584
              tunnel: [w2611 w2619] -> w2562
              tunnel: w2556 -> [_ w2613]
              tunnel: [w2611 w2612] -> w2553
              tunnel: [w2611 w2615] -> w2555
              tunnel: [w2611 w2614] -> w2546
              frame False {
                w2611 = "N_A" ("read buffer")
                n1000 = disable-structure shown="Disabled" {
                  frame Disabled {
                    n1001 = call "Display Message to User7"() -> ()  [unwired: 10 in, 2 out]
                  }
                  frame Enabled {
                  }
                }
              }
              frame True {
                n1002 = property on="UUT SN Report" class="Str"() -> ("Value"=w2612:string)  [unwired: 2 in, 2 out]
                n1003 = call "SerialMarvinSendGet.vi"("write buffer"="VR\r\n", "VISA resource name"=w2613) -> ("error out"=w2616:errorcluster, "read buffer"=w2615:string)  [unwired: 8 in]
                n1004 = property on="UUT" class="DigNum (strict)"(error in=w2616) -> ("Value"=w2618:u8)  [unwired: 1 in, 2 out]
                n1005 = case shown="95, Default" w2618 {
                  tunnel: ["414-8005_95_EBAY_" " 413-8005_47_AHU" " 413-8005_63_AHU"] -> w2620
                  tunnel: ["EBAY 414-8005           " "AHU-L (47) 413-8005-1" "AHU-R (63) 413-8005-2"] -> w2619
                  tunnel: ["414-8005-95" " 413-8005-1-47" " 413-8005-2-63"] -> w2614
                  frame 95, Default {
                  }
                  frame 47 {
                  }
                  frame 63 {
                  }
                }
              }
            }
            n1006 = Get Date/Time String(want seconds? (F)=TRUE) -> (date string=w2600:string)  [unwired: 2 in, 1 out]
            n1007 = call <vilib>:"Open Config Data.vi"("create file if necessary (T)"=FALSE, "configuration file path"=w2559) -> ("refnum"=w2574:T24)  [unwired: 1 in, 8 out]
            n1008 = property on="Logger Path" class="Path"(error in=w2601, "Value"=w2604, "StartPath"=w2604) -> (error out=w2602:errorcluster)  [unwired: 1 in, 1 out]
            n1009 = Search and Replace String(replace all?=TRUE ("replace all? (F)"), input string=w2600, search string="/") -> (result string=w2581:string)  [unwired: 5 in, 3 out]
            n1010 = call-poly <vilib>:"Read Key.vi"("section"=w2567, "key"=w2565, "refnum"=w2574) -> ("error out"=w2569:errorcluster, "value"=w2572:string, "refnum out"=w2571:T24)  [unwired: 5 in, 1 out]
            n1011 = property on="Logger Path" class="Path"(error in=w2602) -> (error out=w2577:errorcluster, "StartPath"=w2580:path)  [unwired: 1 in, 1 out]
            n1012 = call-poly <vilib>:"Read Key.vi"("section"=w2567, "error in (no error)"=w2569, "key"="Tester Software Ver", "refnum"=w2571) -> ("error out"=w2566:errorcluster, "value"=w2564:string, "refnum out"=w2570:T24)  [unwired: 4 in, 1 out]
            n1013 = Concatenate Strings("ATR" ("string"), w2584, w2553, "_", w2581, ".docx" ("string")) -> (w2578:string)
            n1014 = call <vilib>:"Close Config Data.vi"("error in (no error)"=w2566, "refnum"=w2570) -> ()  [unwired: 8 in, 2 out]
            n1015 = Build Path(base path=w2580, name or relative path=w2578) -> (appended path=w2579:path)
            n1016 = call "HeaderuRayon.vi"("Tester Software Ver"=w2564, "UUTHeader"=w2563, "UUT"=w2562, "S/N"=w2553, "VR"=w2555, "Oper."=w2554) -> ("HEADER1"=w2605:string)
            n1017 = Concatenate Strings("  Rev-" ("string"), w2572) -> (w2558:string)
            n1018 = while {
              tunnel: w2578 -> [w2636]
              tunnel: w2580 -> [w2633]
              shift-right: [w2635] -> w2576
              shift-left: w2579 -> [w2634]
              shift-right: [w2631] -> w2560
              shift-left: w2561 -> [w2632]
              tunnel: w2577 -> [w2637]
              tunnel: [w2638] -> _
              stop <- w2630 continue-if-true
              n1019 = call <vilib>:"Check if File or Folder Exists.vi"("error in (no error)"=w2637, "path"=w2634) -> ("error out"=w2638:errorcluster, "file or folder exists?"=w2630:bool)  [unwired: 7 in, 1 out]
              n1020 = case shown="True" w2630 {
                tunnel: w2636 -> [_ w2650]
                tunnel: w2632 -> [_ w2642]
                tunnel: [w2640 w2647] -> w2635
                tunnel: w2634 -> [w2640 _]
                tunnel: w2633 -> [_ w2648]
                tunnel: [1 w2641] -> w2631
                frame False {
                }
                frame True {
                  w2643 = ".docx" ("search string")
                  n1021 = Search and Replace String(input string=w2650, search string=w2643) -> (result string=w2649:string)  [unwired: 6 in, 3 out]
                  n1022 = Number To Decimal String(number=w2642) -> (decimal integer string=w2645:string)  [unwired: 1 in]
                  n1023 = call <vilib>:"Space Constant.vi"() -> ("String"=w2644:string)
                  n1024 = Concatenate Strings(w2649, w2644, w2645, w2643) -> (w2646:string)
                  n1025 = Build Path(base path=w2648, name or relative path=w2646) -> (appended path=w2647:path)
                  n1026 = Increment(x=w2642) -> (x+1=w2641:i32)
                }
              }
            }
            n1027 = Open/Create/Replace File(file path (use dialog)=w2576, operation (0:open)=T22."create") -> (error out=w2590:errorcluster)  [unwired: 4 in, 2 out]
            n1028 = control-ref of="ATR"() -> (w2606:refnum<vi>)
            n1029 = property class="Tbl (strict)"(reference=w2606, error in=w2590) -> ("Value"=w2607:string[][])  [unwired: 2 out]
            n1030 = call "MarvinReport.vi"("HEADER1"=w2605, "ATR Or"=w2606, "Steps   pfull"=w2607, "Footer UUT"=w2546, "pageNum"=3, "FILE NAME"=w2578, "Report Folder"=w2576, "REV"=w2558, "Test-Conductor"=w2554) -> ("error out"=w2541:errorcluster)  [unwired: 5 in, 1 out]
            n1031 = call <vilib>:"Clear Errors.vi"("error in (no error)"=w2541) -> ("error out"=w2540:errorcluster)  [unwired: 5 in, 1 out]
            n1032 = property class="Bool (strict)"(reference=w2552, error in=w2540) -> ("BoolText.Text"=w2551:string)  [unwired: 2 out]
            n1033 = Equal?(x=w2551, y="Report") -> (x = y?=w2545:bool)
            n1034 = Select(t=T10."MainProgram", s=w2545, f=T10."Stop") -> (s? t:f=w2548:T10)
            n1035 = Select(t="Save Report...", s=w2545, f="Program Stopped...\r\nPlease turn OFF All Power sinks") -> (s? t:f=w2543:string)
            n1036 = property on="Report" class="Bool (strict)"(error in=w2540, "Value"=FALSE ("Report")) -> ()  [unwired: 1 in, 2 out]
            n1037 = property on="Pannel User Message" class="Str"("Value"=w2543) -> ()  [unwired: 2 in, 2 out]
          }
          event "Help Button": Value Change {
            n1038 = event-data() -> ()  [unwired: 1 in, 6 out]
            n1039 = vi-ref "Help.vi"() -> (w2666:refnum<vi>)
            n1040 = invoke class="VI" method="FP.Open"(reference=w2666, error in=w2664, "Activate"=TRUE ("Activate?"), "State"=T23."Standard") -> (error out=w2665:errorcluster)  [unwired: 1 in, 4 out]
            n1041 = call "Help.vi"("error in"=w2665) -> ("error out"=w2663:errorcluster)  [unwired: 7 in]
          }
          event "Serial Com": Value Change {
            n1042 = event-data() -> ()  [unwired: 1 in, 6 out]
            n1043 = property on="Serial Com" class="Bool"(error in=w2675, "Visible"=FALSE) -> (error out=w2679:errorcluster)  [unwired: 1 in, 1 out]
            n1044 = property on="VISA Marvin" class="VISAName"(error in=w2679, "Visible"=TRUE) -> (error out=w2676:errorcluster)  [unwired: 1 in, 1 out]
          }
          event "VISA Marvin": Value Change {
            n1045 = event-data() -> ()  [unwired: 1 in, 6 out]
            n1046 = control-ref of="This VI"() -> (w2691:refnum<vi>)
            n1047 = property on="Pannel User Message" class="Str"(error in=w2683, "Value"="Serial connection in process" ("Pannel User Message")) -> ()  [unwired: 1 in, 2 out]
            n1048 = call "Serial InitMarvin.vi"("error in (no error)"=w2683, "VI reference (current VI)"=w2691, "VISA Refnum in"="VISA Marvin") -> ("error out"=w2682:errorcluster, "Boolean"=w2680:bool)  [unwired: 7 in]
            n1049 = property on="VISA Marvin" class="VISAName"(error in=w2682, "Visible"=FALSE) -> (error out=w2694:errorcluster)  [unwired: 1 in, 1 out]
            n1050 = property on="Serial Com" class="Bool"(error in=w2694, "Visible"=TRUE) -> (error out=w2690:errorcluster)  [unwired: 1 in, 1 out]
            n1051 = case shown="True" w2680 {
              tunnel: w2690 -> [w2697 w2709]
              tunnel: "VISA Marvin" -> [w2698 w2706]
              tunnel: [w2698 w2705] -> w2685
              tunnel: [w2697 w2704] -> w2684
              frame False {
              }
              frame True {
                n1052 = call "SerialMarvinSendGet.vi"("error in (no error)"=w2709, "Clear Log"=FALSE, "write buffer"="VC\r\n", "VISA resource name"=w2706) -> ("error out"=w2708:errorcluster, "read buffer"=w2702:string)  [unwired: 6 in]
                n1053 = Decimal String To Number(string=w2702) -> (number=w2701:i32)  [unwired: 2 in, 1 out]
                n1054 = Less Or Equal?(x=w2701, y=50) -> (x <= y?=w2699:bool)
                n1055 = property on="Status" class="Bool (strict)"("Value"=w2699) -> ()  [unwired: 2 in, 2 out]
                n1056 = case shown="True" w2699 {
                  tunnel: w2708 -> [w2710 w2733]
                  tunnel: w2706 -> [w2711 w2732]
                  tunnel: [w2711 w2723] -> w2705
                  tunnel: [w2710 w2717] -> w2704
                  frame False {
                  }
                  frame True {
                    n1057 = call <vilib>:"Clear Errors.vi"("error in (no error)"=w2733) -> ("error out"=w2734:errorcluster)  [unwired: 5 in, 1 out]
                    n1058 = control-ref of="ATR"() -> (w2720:refnum<vi>)
                    n1059 = VISA Flush I/O Buffer(VISA resource name=w2732, error in (no error)=w2734) -> (VISA resource name out=w2723:refnum<visa-resource-name>, error out=w2731:errorcluster)  [unwired: 1 in]
                    n1060 = call "Display Message to User2"("error in (no error)"=w2731) -> ("error out"=w2730:errorcluster, "Yes"=w2729:bool)  [unwired: 9 in]
                    n1061 = case shown="True" w2729 {
                      tunnel: w2730 -> [w2735 w2757]
                      tunnel: [w2735 w2736] -> w2728
                      tunnel: w2723 -> [_ w2754]
                      frame False {
                      }
                      frame True {
                        w2742 = FALSE ("2 Options")
                        n1062 = property on="UUT" class="DigNum (strict)"() -> ("Value"=w2756:u8)  [unwired: 2 in, 2 out]
                        n1063 = call "SetParam.vi"("RS"=TRUE, "error in (no error)"=w2757, "Param to Set in"=w2756, "Visa"=w2754) -> ("error out"=w2737:errorcluster)  [unwired: 7 in]
                        n1064 = control-ref of="Pannel User Message"() -> (w2753:refnum<vi>)
                        n1065 = control-ref of="Stop Burn-in"() -> (w2751:refnum<vi>)
                        n1066 = control-ref of="Stop Button"() -> (w2752:refnum<vi>)
                        n1067 = control-ref of="Motor Speed RPM"() -> (w2750:refnum<vi>)
                        n1068 = property on="VISA Tester" class="VISAName"() -> ("Value"=w2746:refnum<visa-resource-name>)  [unwired: 2 in, 2 out]
                        n1069 = call "TesterOption (SubVI).vi"("2 Options"=w2742, "error in (no error)"=w2737, "On/Off"=FALSE, "Tester Option"=T11."Power", "VISA Refnum in"=w2746) -> ("error out"=w2747:errorcluster, "VISA Refnum out"=w2749:refnum<visa-resource-name>)  [unwired: 5 in]
                        n1070 = call "Write panel message (SubVI).vi"("Stop BurnIn"=w2751, "rpm"=w2750, "PrintTime"=TRUE, "Stop"=w2752, "error in (no error)"=w2747, "Time to wait"=20.0, "Strin"="Restart the UUT\nPlease wait...", "String in"=w2753) -> ("error out"=w2748:errorcluster)  [unwired: 3 in]
                        n1071 = call "TesterOption (SubVI).vi"("2 Options"=w2742, "error in (no error)"=w2748, "On/Off"=FALSE, "Tester Option"=T11."Venable", "VISA Refnum in"=w2749) -> ("error out"=w2736:errorcluster)  [unwired: 5 in, 1 out]
                      }
                    }
                    n1072 = call "Find_Number_LineMARVIN.vi"("Test Paragraph"="7.5.5.1", "TableIn"=w2720) -> ("Line number"=w2721:i32)  [unwired: 3 in, 3 out]
                    n1073 = call "SerialMarvinSendGet.vi"("error in (no error)"=w2728, "write buffer"="SN\r\n", "VISA resource name"=w2723) -> ("error out"=w2724:errorcluster, "read buffer"=w2712:string)  [unwired: 7 in]
                    n1074 = call "SerialMarvinSendGet.vi"("error in (no error)"=w2724, "write buffer"="AO[1]\r\n", "VISA resource name"=w2723) -> ("error out"=w2718:errorcluster, "read buffer"=w2719:string)  [unwired: 7 in]
                    n1075 = Fract/Exp String To Number(string=w2719) -> (number=w2714:dbl)  [unwired: 3 in, 1 out]
                    n1076 = In Range and Coerce(upper limit=0.1 ("x"), x=w2714, lower limit=-0.1) -> (In Range?=w2713:bool)  [unwired: 1 out]
                    n1077 = call "PassOrFail (SubVI).vi"("index (row)"=w2721, "error in (no error)"=w2718, "Data in"=w2714, "Pass?Fail"=w2713, "Table in"=w2720) -> ("error out"=w2717:errorcluster)  [unwired: 6 in]
                    n1078 = property on="UUT SN Report" class="Str"("Value"=w2712) -> ()  [unwired: 2 in, 2 out]
                    n1079 = Decimal String To Number(string=w2712) -> (number=→"Current SN":i32)  [unwired: 2 in, 1 out]
                  }
                }
              }
            }
          }
          event "Refresh Button": Value Change {
            n1080 = event-data() -> ()  [unwired: 1 in, 6 out]
          }
          event "Settings": Value Change {
            n1081 = event-data() -> ()  [unwired: 1 in, 6 out]
            n1082 = control-ref of="VISA Tester"() -> (w2767:refnum<vi>)
            n1083 = control-ref of="UUT"() -> (w2765:refnum<vi>)
            n1084 = property on="Status" class="Bool (strict)"() -> ("Value"=w2769:bool)  [unwired: 2 in, 2 out]
            n1085 = case shown="True" w2769 {
              tunnel: w2775 -> [_ w2787]
              tunnel: [w2776 w2782] -> w2770
              tunnel: w2768 -> [_ w2781]
              tunnel: w2767 -> [_ w2780]
              tunnel: w2766 -> [_ w2779]
              tunnel: w2765 -> [_ w2778]
              frame False {
                n1086 = call "Display Message to User8"() -> ("error out"=w2776:errorcluster)  [unwired: 10 in, 1 out]
              }
              frame True {
                n1087 = vi-ref "Calibration (SubVI).vi"() -> (w2786:refnum<vi>)
                n1088 = invoke class="VI" method="FP.Open"(reference=w2786, error in=w2787, "Activate"=TRUE ("Activate?"), "State"=T23."Standard") -> (error out=w2783:errorcluster)  [unwired: 1 in, 4 out]
                n1089 = call "Calibration (SubVI).vi"("VISA UUT"=w2781, "error constant"=w2783, "UUT"=w2778, "CAN Cluster in"=w2779, "Visa Tester"=w2780) -> ("error constant 2"=w2782:errorcluster, "AO[1]Meas"=→"Cal":dbl)  [unwired: 5 in]
              }
            }
          }
        }
      }
      frame "Initialize" {
        w2791 = FALSE ("Visible")
        w2792 = FALSE ("Visible")
        w2793 = FALSE ("Visible")
        w2794 = FALSE ("Visible")
        w2806 = refnum<visa-resource-name> "COM1" ("VISA resource name")
        w2796 = FALSE ("Visible")
        w2788 = FALSE ("Serial Status")
        n1090 = property on="ComTestResult" class="Bool (strict)"("Value"=w2794) -> ()  [unwired: 2 in, 2 out]
        n1091 = property on="VenableResult" class="Bool (strict)"("Value"=w2794) -> ()  [unwired: 2 in, 2 out]
        n1092 = property on="VenableDirectionResult" class="Bool (strict)"("Value"=w2794) -> ()  [unwired: 2 in, 2 out]
        n1093 = property on="SpeedResult" class="Bool (strict)"("Value"=w2794) -> ()  [unwired: 2 in, 2 out]
        n1094 = property on="Serial Com" class="Bool"(error in=errorcluster {"status"=FALSE, "code"=0, "source"=""} ("error out"), "Visible"=TRUE) -> (error out=w2808:errorcluster)  [unwired: 1 in, 1 out]
        n1095 = property on="AuxiOFFResult" class="Bool (strict)"("Value"=w2793) -> ()  [unwired: 2 in, 2 out]
        n1096 = property on="AuxiONResult" class="Bool (strict)"("Value"=w2793) -> ()  [unwired: 2 in, 2 out]
        n1097 = property on="VisualInspectionResult" class="Bool (strict)"("Value"=w2793) -> ()  [unwired: 2 in, 2 out]
        n1098 = property on="SensCalResult" class="Bool (strict)"("Value"=w2793) -> ()  [unwired: 2 in, 2 out]
        n1099 = property on="VISA Marvin" class="VISAName"(error in=w2808, "Visible"=w2796, "Value"=w2806) -> (error out=w2797:errorcluster)  [unwired: 1 in, 1 out]
        n1100 = property on="Stop Burn-in" class="Bool (strict)"(error in=w2797, "Visible"=w2796) -> (error out=w2789:errorcluster)  [unwired: 1 in, 1 out]
        n1101 = property on="BurnDC" class="Bool (strict)"("Value"=w2792) -> ()  [unwired: 2 in, 2 out]
        n1102 = property on="BurnTemp" class="Bool (strict)"("Value"=w2792) -> ()  [unwired: 2 in, 2 out]
        n1103 = property on="BurnSpeed" class="Bool (strict)"("Value"=w2792) -> ()  [unwired: 2 in, 2 out]
        n1104 = property on="BurnResult" class="Bool (strict)"("Value"=w2792) -> ()  [unwired: 2 in, 2 out]
        n1105 = property on="Refresh Button" class="Bool (strict)"(error in=w2789, "Value"=FALSE ("Refresh Button")) -> ()  [unwired: 1 in, 2 out]
        n1106 = property on="StopTimeResult" class="Bool (strict)"("Value"=w2791) -> ()  [unwired: 2 in, 2 out]
        n1107 = property on="MotorTempResult" class="Bool (strict)"("Value"=w2791) -> ()  [unwired: 2 in, 2 out]
        n1108 = property on="TempControlResult" class="Bool (strict)"("Value"=w2791) -> ()  [unwired: 2 in, 2 out]
        n1109 = property on="Automation" class="Bool (strict)"("Value"=w2791) -> ()  [unwired: 2 in, 2 out]
        n1110 = flat-sequence {
          tunnel: w2789 -> [w2811]
          tunnel: [w2810] -> w2804
          tunnel: [w2814] -> w2803
          tunnel: w2804 -> [w2814]
          tunnel: [w2826] -> w2802
          tunnel: w2803 -> [w2827]
          tunnel: [w2827] -> w2801
          frame #0 {
            n1111 = control-ref of="This VI"() -> (w2812:refnum<vi>)
            n1112 = invoke class="VI" method="Default Vals.Reinit All"(reference=w2812, error in=w2811) -> (error out=w2810:errorcluster)  [unwired: 1 in, 2 out]
          }
          frame #1 {
            w2817 = u32 4294967295  # AccMask
            w2813 = T4 0 items=["使用Flash参数", "使用界面设置参数"] ("InitFlag")
            w2815 = T6 0 items=["normal operation", "Listen-only mode", "test mode"]  # Mode
            w2816 = T5 3 items=["接收所有类型"=1, "只接收标准帧"=2, "只接收扩展帧"=3] ("Fliter")
            w2821 = u8 10 items=["5k bps"=1, "10k bps"=2, "20k bps"=3, "40k bps"=4, "50k bps"=5, "80k bps"=6, "100k bps"=7, "125k bps"=8, "200k bps"=9, "250k bps"=10, "400k bps"=11, "500k bps"=12, "666k bps"=13, "800k bps"=14, "1000k bps"=15, "33.33k bps"=16, "66.66k bps"=17, "83.33k bps"=18]  # kBaudRate
            w2818 = u32 0  # AccCode
            w2819 = T2 4 items=["USB-CAN"=3, "USB-CAN2"=4] ("DevType")
            w2820 = T7 {"DevType"=3, "DevIndex"=0, "CanIndex"=0, "VCI_INIT_CONFIG"={"AccCode"=0, "AccMask"=0, "InitFlag"=1, "Fliter"=7, "Timing0"=0, "Timing1"=0, "Mode"=0}}  # Config
            # "CANalystII"
            n1113 = call "Demo_GetT0T1.vi"("kBaudRate"=w2821) -> ("Timing0"=w2823:u8, "Timing1"=w2824:u8)
            n1114 = Bundle By Name(cluster=w2820, "DevType"=w2819, "CanIndex"="Channel 2", "VCI_INIT_CONFIG.AccCode"=w2818, "VCI_INIT_CONFIG.AccMask"=w2817, "VCI_INIT_CONFIG.InitFlag"=w2813, "VCI_INIT_CONFIG.Fliter"=w2816, "VCI_INIT_CONFIG.Timing0"=w2823, "VCI_INIT_CONFIG.Timing1"=w2824, "VCI_INIT_CONFIG.Mode"=w2815) -> (→"Config_CANAT":T7)
          }
          frame #2 {
            w2828 = u16 284 items=["1M"=20, "500K"=28, "250K"=284, "125K"=796, "100K"=17199, "50K"=18223, "20K"=21295, "10K"=26415, "5K"=32639] ("baud in")
            n1115 = control-ref of="Config_CANAT"() -> (w2826:refnum<vi>)
            n1116 = call "InitCAN_ATII.vi"("Config"=w2826) -> ("Sts"=→"CAN Status":bool)
            n1117 = call "ChangeCANBaud.vi"("baud in"=w2828, "reference"=w2826) -> ()
          }
        }
        "Status" <- w2788
        "Test Failed" <- w2788
      }
    }
  }
  n1118 = property on="Settings" class="Bool (strict)"("Visible"=w3) -> ()  [unwired: 2 in, 2 out]
  n1119 = property on="Cal" class="DigNum (strict)"("Visible"=w3) -> ()  [unwired: 2 in, 2 out]
  n1120 = disable-structure shown="Disabled" {
    frame Disabled {
      w2830 = T18."Disabled and Grayed Out" ("Disabled")
      w2831 = FALSE ("Start")
      n1121 = property on="VISA Tester" class="VISAName" props=["Value"]() -> ()  [unwired: 2 in, 3 out]
      n1122 = property on="Current SN" class="DigNum (strict)" props=["Value"]() -> ()  [unwired: 2 in, 3 out]
      n1123 = property on="UUT" class="DigNum (strict)" props=["Value"]() -> ()  [unwired: 2 in, 3 out]
      n1124 = property on="Status" class="Bool (strict)" props=["Value"]() -> ()  [unwired: 2 in, 3 out]
      n1125 = property on="UUT SoftwareVer" class="Str" props=["Value"]() -> ()  [unwired: 2 in, 3 out]
      n1126 = property on="Next SN" class="DigNum (strict)" props=["Value"]() -> ()  [unwired: 3 in, 2 out]
      n1127 = property on="Start" class="Bool (strict)"("Value"=w2831, "DisabledEnum"=w2830) -> ()  [unwired: 2 in, 2 out]
      n1128 = property on="Report" class="Bool (strict)"("Value"=w2831, "DisabledEnum"=w2830) -> ()  [unwired: 2 in, 2 out]
    }
    frame Enabled {
    }
  }
  n1129 = disable-structure shown="Disabled" {
    frame Disabled {
      (unwired) 0.02003173828125 ("x")
      n1130 = control-ref of="Stop Burn-in"() -> ()  [unwired: 1 out]
      n1131 = control-ref of="Stop Button"() -> ()  [unwired: 1 out]
      n1132 = control-ref of="Motor Speed RPM"() -> ()  [unwired: 1 out]
      n1133 = control-ref of="Config_CANAT"() -> ()  [unwired: 1 out]
      n1134 = control-ref of="UUT"() -> ()  [unwired: 1 out]
      n1135 = call "GetADCTester (SubVI).vi"() -> ()  [unwired: 9 in, 3 out]
      n1136 = call "CANSendMotorSpeed.vi"() -> ()  [unwired: 11 in, 1 out]
      n1137 = control-ref of="Config_CANAT"() -> ()  [unwired: 1 out]
      n1138 = call "Find_Number_LineMARVIN.vi"() -> ()  [unwired: 5 in, 4 out]
      n1139 = property on="UUT" class="DigNum (strict)" props=["Value"]() -> ()  [unwired: 2 in, 3 out]
      n1140 = control-ref of="UUT"() -> ()  [unwired: 1 out]
      n1141 = call "DegToDAC (SubVI).vi"() -> ()  [unwired: 10 in, 2 out]
      n1142 = call "Write panel message (SubVI).vi"() -> ()  [unwired: 11 in, 1 out]
      n1143 = property on="VISA Tester" class="VISAName" props=["Value"]() -> ()  [unwired: 2 in, 3 out]
      n1144 = control-ref of="ATR"() -> ()  [unwired: 1 out]
      n1145 = call "TesterOption (SubVI).vi"() -> ()  [unwired: 10 in, 2 out]
      n1146 = call "TesterOption (SubVI).vi"() -> ()  [unwired: 10 in, 2 out]
      n1147 = call "PassOrFail (SubVI).vi"() -> ()  [unwired: 11 in, 1 out]
    }
    frame Enabled {
    }
  }
  n1148 = disable-structure shown="Disabled" {
    frame Disabled {
      n1149 = flat-sequence {
        frame #0 {
          n1150 = call "CANSendMotorSpeed.vi"("Remote"=TRUE, "Motor Speed RPM"=u16 0) -> ("error out"=w2833:errorcluster, "UUT"=w2836:refnum<vi>)  [unwired: 8 in]
          n1151 = property on="VISA Tester" class="VISAName"() -> ("Value"=w2832:refnum<visa-resource-name>)  [unwired: 2 in, 2 out]
          n1152 = call "TesterOption (SubVI).vi"("error in (no error)"=w2833, "On/Off"=FALSE, "Tester Option"=T11."Power", "VISA Refnum in"=w2832) -> ()  [unwired: 6 in, 2 out]
        }
      }
    }
    frame Enabled {
    }
  }
  "Pannel User Message" <- w1
